vi "Cascade front panel 64.vi"() -> ()   [LabVIEW 2016]
uses:
  controls/KPro Header Control 1.ctl
  sdi_12/SDI-12/Sonde Vertical Graph.ctl
  controls/Vertical Chart.ctl
  sdi_12/Groundwater header.ctl
  controls/MCC DAQ Setup.ctl
  controls/Aux Sensor.ctl
  KPRO_2016 subvis/Control 2.ctl
  KPRO_2016 subvis/Graph Controls 2.ctl
  KPRO_2016 subvis/Ik control.ctl
  controls/MCC DAQ Readings.ctl
  controls/Kpro pressure measurement cluster.ctl
  controls/Kpro hydraulic measurement cluster.ctl
  Cascade/Waterloo DAQ/controls/Sonde Data Array Control 1.ctl
  Cascade/Waterloo DAQ/controls/Sonde Data Control 1.ctl
  sdi_12/Sonde Value Percent Tol.ctl
  activeXtest/activeXtest 2015 Folder/sample data row cluster.ctl
  activeXtest/activeXtest 2015 Folder/sonde cluster.ctl
  controls/Display Control 1.ctl
  KPRO_2016 subvis/Sensor Physical Measurements.ctl
  KPRO_2016 subvis/SS Control 7.ctl
  <vilib>/Utility/NIReport.llb/NI_report.lvclass
  controls/Action Control 1.ctl
  <extravilib>/ChannelInstances/One Element Stream-t'Action Control 1.ctl'/Instantiate.vi
  <extravilib>/ChannelInstances/One Element Stream-t'Action Control 1.ctl'/EndpointRead.vi
  KPRO_2016 subvis/Kpro Globals.vi
  <vilib>/Utility/file.llb/Write Delimited Spreadsheet (DBL).vi
  <vilib>/Utility/file.llb/Write Delimited Spreadsheet (string).vi
  <vilib>/ULx/Create Channel.llb/ULx Create Channel (AI-Voltage-Basic).vi
  <userlib>/_OpenG.lib/file/file.llb/Build Path - Traditional__ogtk.vi
  <userlib>/_OpenG.lib/file/file.llb/File Exists - Scalar__ogtk.vi
  <userlib>/_OpenG.lib/file/file.llb/Strip Path - Traditional__ogtk.vi
  KPRO_2016 subvis/Global_SIM_switch.vi
  <extravilib>/ChannelInstances/One Element Stream-t'Action Control 1.ctl'/Endpoint.vi
  C:/Program Files/National Instruments/LabVIEW 2016/vi.lib/ULx/ULx_LV.dll
  Program Files/National Instruments/LabVIEW 2016/vi.lib/ULx/ULx_LV.dll
  <vilib>/Utility/config.llb/NI_LVConfig.lvlib
  <extravilib>/ChannelInstances/One Element Stream-t'Action Control 1.ctl'.lvlib
panel:
  out "Zero Pressure\nIndicator":bool
  in  "Zero\nPressure":bool caption="Zero Pressure"
  in  "enable_IKMGS_file":bool
  in  "enable_slug_file":bool
  in  "enable_kpro_file":bool=TRUE
  in  "Simulate AD6B":bool
  out "KPRO Test\nIndicator":bool
  in  "Record DTW File":bool
  in  "Zero In-Line Pressure\n(F = leave as is)":bool=TRUE
  in  "Corrected Pressure Cluster":T1
  in  "Create Excel Files":bool
  out "Tab Page":i32
  out "Sonde Data":string[][](array[string])
  out "Current \nDepth (m)":sgl=-30.661383 format="%.2f"
  out "Sonde Recording":string[][](array[string])
  out "Column of Volume":i32
  in  "Input Variables and Slopes 2":T2={"Total Volume"=0.0, "String Pot Slope"=1.6619999408721924, "Flow Slope"=39.040000915527344, "Up Hole Pressure Slope"=48.27000045776367, "Depth to Water Table"=-0.0, "Atmospheric Pressure"=32.22022530555725, "DH Pressure Trans Slope"=42.0, "DH Pressure Offset"=0.0, "Up Hole  Pressure Offset"=0.0, "Aux 1 Slope"=1.0, "Aux 2 Slope"=1.0, "Aux 3 Slope"=1.0, "Aux 1 Offset"=0.0, "Aux 2 Offset"=0.0, "Aux 3 Offset"=0.0, "String Pot Offset"=0.0, "Flow Offset"=0.0, "Reservoir Pressure"=-0.004827000045779073, "Height of Sample Box"=0.0} {"Height of Sample Box" format="%.2f"; "Reservoir Pressure" format="%.2f"; "Flow Offset" format="%.2f"; "String Pot Offset" format="%.2f"; "Aux 3 Offset" format="%.2f"; "Aux 2 Offset" format="%.2f"; "Aux 1 Offset" format="%.2f"; "Aux 3 Slope" format="%.2f"; "Aux 2 Slope" format="%.2f"; "Aux 1 Slope" format="%.2f"; "Up Hole  Pressure Offset" format="%.2f"; "DH Pressure Offset" format="%.2f"; "DH Pressure Trans Slope" format="%.2f"; "Atmospheric Pressure" format="%.2f"; "Depth to Water Table" format="%.2f"; "Up Hole Pressure Slope" format="%.2f"; "Flow Slope" format="%.2f"; "String Pot Slope" format="%.2f"; "Total Volume" format="%.2f"}
  out "Select Worksheet Index":i32
  out "Number of Sample Sheets":i32
  out "NI_report out":refnum<class "NI_report.lvclass">
  out "Sonde":bool
  out "DAQ":bool
  in  "Depth mode":bool=TRUE caption="Use \nIncrement"
  in  "Increment Depth":bool
  in  "Finish Tests":bool
  in  "Start KPRO":bool
  in  "stop":bool
  in  "Write Data to Spreadsheet":bool
  in  "Sonde Sample Not Collected":bool
  in  "Record Single Sample":bool
  in  "Sample Sheet Data Row Cluster 2":T3={"Head\nPressure"=0.0, "Depth"=0.0, "comment "="", "Sonde Data Cluster"={"Cumulative\nVolume (ml)"=100.0, "Specific\nCond (mS)"=2.0, "Dissolved\nOxygen mg/L"=3.0, "pH"=4.0, "ORP"=5.0, "Temp deg C"=26.0, "Salinity"=7.0}, "Aux1"=0.0, "Aux2"=0.0, "Aux3"=0.0} {"Sonde Data Cluster"."Salinity" format="%_3g"; "Sonde Data Cluster"."Temp deg C" format="%_2g"; "Sonde Data Cluster"."ORP" format="%_4g"; "Sonde Data Cluster"."pH" format="%_4g"; "Sonde Data Cluster"."Dissolved\nOxygen mg/L" format="%_4g"; "Sonde Data Cluster"."Specific\nCond (mS)" format="%_4g"; "Sonde Data Cluster"."Cumulative\nVolume (ml)" format="%#_4g"; "Depth" format="%#.3g"; "Head\nPressure" format="%#.4g"}
  out "Current Time (s)":dbl
  in  "Tab Control":T5(tab)
  out "Height of Box Global":dbl
  out "Depth to Water Table Global":dbl
  out "Reservoir Pressure Global":dbl
  out "Atmospheric Pressure Global":dbl
  out "Current Depth Global":dbl
  out "Increment Global":dbl
  out "Distance Global":dbl
  out "Profile ID":string
  out "KPRO Box Global":dbl
  out "Ion Offset Global":dbl
  out "Ion Slope Global":dbl
  out "Flow Slope Global":dbl
  out "Pressure Slope Global":dbl
  out "String Pot  Slope Global":dbl
  in  "Config File Path":path=path "C:/Cascade/Data/config files/DAQ Setup Config.ini"
  in  "Read Configuration File?":bool
  in  "Save Configuration File?":bool
  out "12V Voltage Monitor":dbl format="%_3f"
  out "Found Quanta Sonde Com Port":refnum<visa-resource-name>
  out "Quanta Sonde found?":bool
  out "H-4191 Adapter found":bool
  out "Sonde Communication Error Out":errorcluster
  in  "Search for Comm Ports?":bool=TRUE
  in  "USB Serial Port Manual Entry":refnum<visa-resource-name>="COM13"
  in  "Sonde Parameters \nTolerance Limits":T6={"SC %"=10.0, "DO %"=10.0, "pH % "=10.0, "ORP % "=10.0, "Temp % "=10.0, "Salinity %"=10.0} {"Salinity %" format="%_2f%%"; "Temp %" format="%_2f%%"; "ORP %" format="%_2f%%"; "pH %" format="%_2f%%"; "DO %" format="%_2f%%"; "SC %" format="%_2f%%"}
  in  "Sonde Parameters \nInitial Values":T7 {"Salinity Initial" format="%_2f"; "Temp Initial" format="%_2f"; "ORP  Initial" format="%_2f"; "pH Initial" format="%_2f"; "DO Initial" format="%_2f"; "SC Initial" format="%_2f"}
  out "Sensor  Real \nMeasurements":T8 {"9V Monitor" format="%#.3g"; "Aux 3" format="%#.3g"; "Aux 2" format="%#.3g"; "Aux 1" format="%#.3g"; "String Pot" format="%#.3g"; "Top String Pot" format="%#_4g"; "Downhole Pressure" format="%#_4g"; "Flow" format="%#_4g"; "Uphole Pressure" format="%#_4g"}
  in  "MCC USB-DAQ Setup":T9={"Device Name in InstaCal"="Dev0", "Omega Pressure Sensor"={"DAQ Channel"=2.0, "Input Voltage Range"=1, "Enabled"=TRUE, "Description"="Uphole Pressure"}, "McMillian 102 Flowmeter"={"DAQ Channel"=11.0, "Input Voltage Range"=0, "Enabled"=TRUE, "Description"="Flow"}, "DHT Pressure Sensor"={"DAQ Channel"=3.0, "Input Voltage Range"=1, "Enabled"=TRUE, "Description"="Downhole Pressure"}, "Top String Pot"={"DAQ Channel"=0.0, "Input Voltage Range"=0, "Enabled"=TRUE, "Description"="Top String Pot"}, "String Pot Signal"={"DAQ Channel"=1.0, "Input Voltage Range"=0, "Enabled"=TRUE, "Description"="String Pot"}, "Aux Sensor 1"={"DAQ Channel"=5.0, "Input Voltage Range"=1, "Enabled"=TRUE, "Description"="Aux 1"}, "Aux Sensor 2"={"DAQ Channel"=6.0, "Input Voltage Range"=1, "Enabled"=TRUE, "Description"="Aux 2"}, "Aux Sensor 3"={"DAQ Channel"=7.0, "Input Voltage Range"=1, "Enabled"=TRUE, "Description"="Aux 3"}, "Voltage Monitor"={"DAQ Channel"=8.0, "Input Voltage Range"=0, "Enabled"=TRUE, "Description"="9V Monitor"}} {"Voltage Monitor"."Input Voltage Range" items=["+/-10 V Range", "+/-5 V Range", "+/-2.5V Range", "+/-1.25 V Range", "+/-0.625 V Range", "+/-0.3125 V Range", "+/-0.1562V Range", "+/-0.078125 V Range"]; "Aux Sensor 3"."Input Voltage Range" items=["+/-10 V Range", "+/-5 V Range", "+/-2.5V Range", "+/-1.25 V Range", "+/-0.625 V Range", "+/-0.3125 V Range", "+/-0.1562V Range", "+/-0.078125 V Range"]; "Aux Sensor 2"."Input Voltage Range" items=["+/-10 V Range", "+/-5 V Range", "+/-2.5V Range", "+/-1.25 V Range", "+/-0.625 V Range", "+/-0.3125 V Range", "+/-0.1562V Range", "+/-0.078125 V Range"]; "Aux Sensor 1"."Input Voltage Range" items=["+/-10 V Range", "+/-5 V Range", "+/-2.5V Range", "+/-1.25 V Range", "+/-0.625 V Range", "+/-0.3125 V Range", "+/-0.1562V Range", "+/-0.078125 V Range"]; "String Pot Signal"."Input Voltage Range" items=["+/-10 V Range", "+/-5 V Range", "+/-2.5V Range", "+/-1.25 V Range", "+/-0.625 V Range", "+/-0.3125 V Range", "+/-0.1562V Range", "+/-0.078125 V Range"]; "Top String Pot"."Input Voltage Range" items=["+/-10 V Range", "+/-5 V Range", "+/-2.5V Range", "+/-1.25 V Range", "+/-0.625 V Range", "+/-0.3125 V Range", "+/-0.1562V Range", "+/-0.078125 V Range"]; "DHT Pressure Sensor"."Input Voltage Range" items=["+/-10 V Range", "+/-5 V Range", "+/-2.5V Range", "+/-1.25 V Range", "+/-0.625 V Range", "+/-0.3125 V Range", "+/-0.1562V Range", "+/-0.078125 V Range"]; "McMillian 102 Flowmeter"."Input Voltage Range" items=["+/-10 V Range", "+/-5 V Range", "+/-2.5V Range", "+/-1.25 V Range", "+/-0.625 V Range", "+/-0.3125 V Range", "+/-0.1562V Range", "+/-0.078125 V Range"]; "Omega Pressure Sensor"."Input Voltage Range" items=["+/-10 V Range", "+/-5 V Range", "+/-2.5V Range", "+/-1.25 V Range", "+/-0.625 V Range", "+/-0.3125 V Range", "+/-0.1562V Range", "+/-0.078125 V Range"]}
  out "Rate":dbl=1000.0 caption="Channel\nSample Rate (Hz)"
  out "Number \nof Channels":u16
  in  "DAQ \nData Rate S/s":dbl=3720.0 format="%#_13g"
  out "Descriptions":string[](array[string])
  out "Raw Voltages":dbl[](array[numeric])
  out "9V Voltage Monitor":dbl format="%#_3g"
  in  "Record DAQ Raw Voltages":bool
  out "Sensor Voltage Cluster":T11 {"9V Monitor" format="%#.3g"; "Aux 3" format="%#_3g"; "Aux 2" format="%#.3g"; "Aux 1" format="%#.3g"; "String Pot" format="%#.3g"; "Top String Pot" format="%#_3g"; "Downhole Pressure" format="%#.3g"; "Flow" format="%#_3g"; "Uphole Pressure" format="%-#1.3g"}
  out "Worksheet Names":string[](array[string])
  out "row max value":i32
  out "last occupied cell's name":string
  out "column max value":i32
  in  "Current Sample Sheet":string="Sample 1"
  out "Columns":i32[](array[numeric])
  in  "Header path":path=path "C:/Cascade/templates/Fields for Excel sheets.xlsx"
  in  "template file path":path=path "C:/Cascade/templates/Groundwater Profiling Log_empty_labview_template.xlsx"
  in  "Data File Directory":path=path "C:/Cascade/Data/Excel Reports"
  in  "Excel report file path":path=path "C:/Cascade/Data/Excel Reports/Groundwater Profiling Log_ara1.xlsx"
  in  "Clear Groundwater Header Values":bool
  in  "Groundwater Header":T12
  out "Data Setup Indicator":string
  in  "Start Initialization":bool
  in  "Input Variables and Slopes":T2={"Total Volume"=0.0, "String Pot Slope"=1.6619999408721924, "Flow Slope"=39.040000915527344, "Up Hole Pressure Slope"=48.27000045776367, "Depth to Water Table"=-0.0, "Atmospheric Pressure"=32.22022530555725, "DH Pressure Trans Slope"=42.0, "DH Pressure Offset"=0.0, "Up Hole  Pressure Offset"=0.0, "Aux 1 Slope"=1.0, "Aux 2 Slope"=1.0, "Aux 3 Slope"=1.0, "Aux 1 Offset"=0.0, "Aux 2 Offset"=0.0, "Aux 3 Offset"=0.0, "String Pot Offset"=0.0, "Flow Offset"=0.0, "Reservoir Pressure"=-0.004827000045779073, "Height of Sample Box"=0.0} {"Height of Sample Box" format="%.2f"; "Reservoir Pressure" format="%.2f"; "Flow Offset" format="%.2f"; "String Pot Offset" format="%.2f"; "Aux 3 Offset" format="%.2f"; "Aux 2 Offset" format="%.2f"; "Aux 1 Offset" format="%.2f"; "Aux 3 Slope" format="%.2f"; "Aux 2 Slope" format="%.2f"; "Aux 1 Slope" format="%.2f"; "Up Hole  Pressure Offset" format="%.2f"; "DH Pressure Offset" format="%.2f"; "DH Pressure Trans Slope" format="%.2f"; "Atmospheric Pressure" format="%.2f"; "Depth to Water Table" format="%.2f"; "Up Hole Pressure Slope" format="%.2f"; "Flow Slope" format="%.2f"; "String Pot Slope" format="%.2f"; "Total Volume" format="%.2f"}
  out "appended path":path
  out "Down hole Pressure Transducer CSV data  path":path
  in  "Static IK path":path
  in  "Slopes File Path":path=path "C:/Cascade/Data/Output Files/slopes.csv"
  out "Output File Path":path
  out "KPRO SessionOutput File Path":path
  in  "Slopes History File Path":path=path "C:/Cascade/Data/Output Files/slopes-cal-record.csv"
  out "Sonde Recording Error file":path
  out "IK Recording Error file":path
  out "Sonde Output File Path":path
  out "KPRO Cumulative Output File Path":path
  in  "Temporary Data Files Directory":path=path "C:/Cascade/Data/Output Files"
  in  "Update Sonde":bool
  in  "Sonde Data Array":T13 {"Salinity"."%" format="%_2f%%"; "Salinity"."Value" format="%_4g"; "Temperature"."%" format="%_2f%%"; "Temperature"."Value" format="%_4g"; "ORP"."%" format="%_2f%%"; "ORP"."Value" format="%_4g"; "pH"."%" format="%_2f%%"; "pH"."Value" format="%_4g"; "Dissolved Oxygen"."%" format="%_2f%%"; "Dissolved Oxygen"."Value" format="%_4g"; "Sp. Conductance"."%" format="%_2f%%"; "Sp. Conductance"."Value" format="%_4g"; "Cumulative\nVolume" format="%#_4g"}
  out "Table Label":string="Data from Sample  %d from Excel File"
  out "Sonde Array Size":i32
  in  "Current Sonde Sample":i32=1
  out "Sonde Data Display":T16
  out "Temperature":cluster{"Y":dbl[], "Y":dbl[]}[](graph)
  in  "Record  Sonde Reason":bool
  in  "Select Reasons to Record Data":u16(ring) items=["Per Client Request", "Timed Out", "Sample stopped flowing", "Equipment Issue"]
  out "Sonde Recording Failure Path":path
  in  "Sonde IK Recording Failure Path":path
  out "Recording Reason Sonde array":string[][](array[string])
  out "IK Reason array":string[][](array[string])
  in  "Sonde Calibration History File":path
  out "SC Reference (uS/cm) Calibration Response":T18
  out "DO Reference % Calibration Response":T18
  out "Salinity Reference Calibration Response":T18
  out "ORP Reference Calibration Response":T18
  out "pH Reference Calibration Response":T18
  out "pH Zero Calibration Response":T18
  in  "Salinity \nReference":dbl
  in  "SC \nReference (uS/cm)":dbl
  in  "DO Reference %":dbl
  in  "ORP Reference":dbl
  in  "pH Reference":dbl
  in  "pH Zero":dbl
  in  "Record  SC Calibration":bool
  in  "Record DO Calibration":bool
  in  "Record Salinity Calibration":bool
  in  "Record ORP Calibration":bool
  in  "Record pH Calibration Reference":bool
  in  "Record pH Calibration Zero":bool
  out "KPRO Finish\nIndicator":bool
  in  "Input Depths \nand Parameters Cluster":T19={"Flow"=0.21081600494384767, "Zeroed \nPressure"=74.74207969932556, "Ik"=0.003788962123473114, "Current Depth"=-100.6, "Feet of Stainless"=40, "Start Depth"=0.0, "Abs Start Depth"=0.0} {"Abs Start Depth" format="%.2f"; "Start Depth" format="%.2f"; "Current Depth" format="%.2f"; "Ik" format="%.2f"; "Zeroed \nPressure" format="%.2f"; "Flow" format="%.2f"}
  out "Current Session":sgl[][](array[numeric]) format="%.2f"
  in  "KPRO session report header":T20=["Time(msecs)", "Uncorrected Depth", "Corrected Depth", "Drive_Rate", "Flow", "Feet_of Stainless", "Up Hole Pressure", "IK", "Corrected Pressure", "Atm Pressure", "Depth to water", "Height of box", "Res_Pressure", "Secs_since_1_JAN_1904", "Depth jumps more than 1_foot", "Down hole Pressure"]
  in  "Depth Cluster":T21
  out "Cumulative_data_from_file":sgl[][](array[numeric]) format="%.2f"
  in  "KPRO Culmulative \ntest report header 2":T20=["Time(msecs)", "Uncorrected Depth", "Corrected Depth", "Drive_Rate", "Flow", "Feet_of Stainless", "Up Hole Pressure", "IK", "Corrected Pressure", "Atm Pressure", "Depth to water", "Height of box", "Res_Pressure", "Secs_since_1_JAN_1904", "Depth jumps more than 1_foot", "Down hole Pressure"]
  out "Cumulative_data_ready":bool
  out "DHT IK":T22=0.003788962123473114 caption="Real Time - Depth vs. lk" format="%.2f"
  out "Depth to Water":sgl=-100.6 format="%.2f"
  out "Depth Rate\nft/min":T22 format="%#.2g"
  out "Ik":dbl=0.003788962123473114 caption="Real Time - Depth vs. lk" format="%.2f"
  out "Corrected\n Pressure (ft)":dbl format="%.2f"
  in  "New Depth":dbl min=-100.0 max=0.0
  in  "Update Depth":bool
  in  "Select Entry \nfor IK Log":u16(ring) items=["IK Increase", "IK stayed the Same", "IK decreased"]
  out "Large Depth IK Graph Cluster":T23={[0.003788962123473114, 0.0037174584307500765, 0.0037174584307500765, 0.0037174584307500765, 0.0037174584307500765, 0.003788962123473114], [-100.1, -100.2, -100.3, -100.4, -100.5, -100.6]}
  in  "Culmulative Graph Cluster":T24={"Cumulative - Depth vs. Ik"={[], []}, "Real Time - Depth vs. lk "={[0.003788962123473114, 0.0037174584307500765, 0.0037174584307500765, 0.0037174584307500765, 0.0037174584307500765, 0.003788962123473114], [-100.1, -100.2, -100.3, -100.4, -100.5, -100.6]}, "Cumulative - Depth vs. Drive Rate"={[], []}, "Real Time - Depth vs. Drive Rate"={[0.02036245163917736, 0.125, 0.16666666666666674, 0.16666666666666663, 0.16666666666666663, 0.16666666666666663], [-100.1, -100.2, -100.3, -100.4, -100.5, -100.6]}}
  out "Down hole Pressure (ft)":dbl format="%.2f"
  out "Flow":T22 format="%#.2g"
  out "Current Depth":sgl=-100.6 format="%.2f"
  in  "Read String Pot":bool=TRUE
  in  "Record IK Reason":bool
  out "Large Depth IK Graph":dbl(graph)
  out "DAQ Error":errorcluster
  out "Initialization Finished":bool=TRUE
  out "Stop":bool
  out "error out":errorcluster
  in  "error in (no error)":errorcluster
  out "producer loop":i32
  out "consumer loop":i32
  out "Active Channel Array":string[](array[string])
  out "Voltage Range":dbl[](array[numeric])
  out "delimited string":string
  out "Stop 2":bool
  out "output cluster":T4 caption="Cluster" {"Salinity" format="%_3g"; "Temp deg C" format="%_2g"; "ORP" format="%_4g"; "pH" format="%_4g"; "Dissolved\nOxygen mg/L" format="%_3g"; "Specific\nCond (mS)" format="%_4g"; "Cumulative\nVolume (ml)" format="%#_4g"}
  out "Serial Number/MISC":string
  out "subarray":string[][](array[string])
  out "Initialization":i32
  in  "Record Continuous Samples":bool
  # "Global Variables"
  # "ft. water"
  # "mL/min."
  # "ft. water"
  # "ft."
  # "ft."
  # "Instructions for Sonde Calibration:\n1.  Use the Record Single Point to Record the Data prior to start of\ncalibration procedure to record the initial points to the excel worksheet.\n2.  pH Calibration is a 2 step process:  A pH standard between 6.8 and 7.2 is treated as the “zero”\nand all other values are treated as the “slope”. First calibrate “zero”, then  add a second to calibrate “slope”. \n3.  Specific Conductance:  Wait for the specific conductance readings to stabilize in the calibration solution, which may\nrequire one or two minutes."
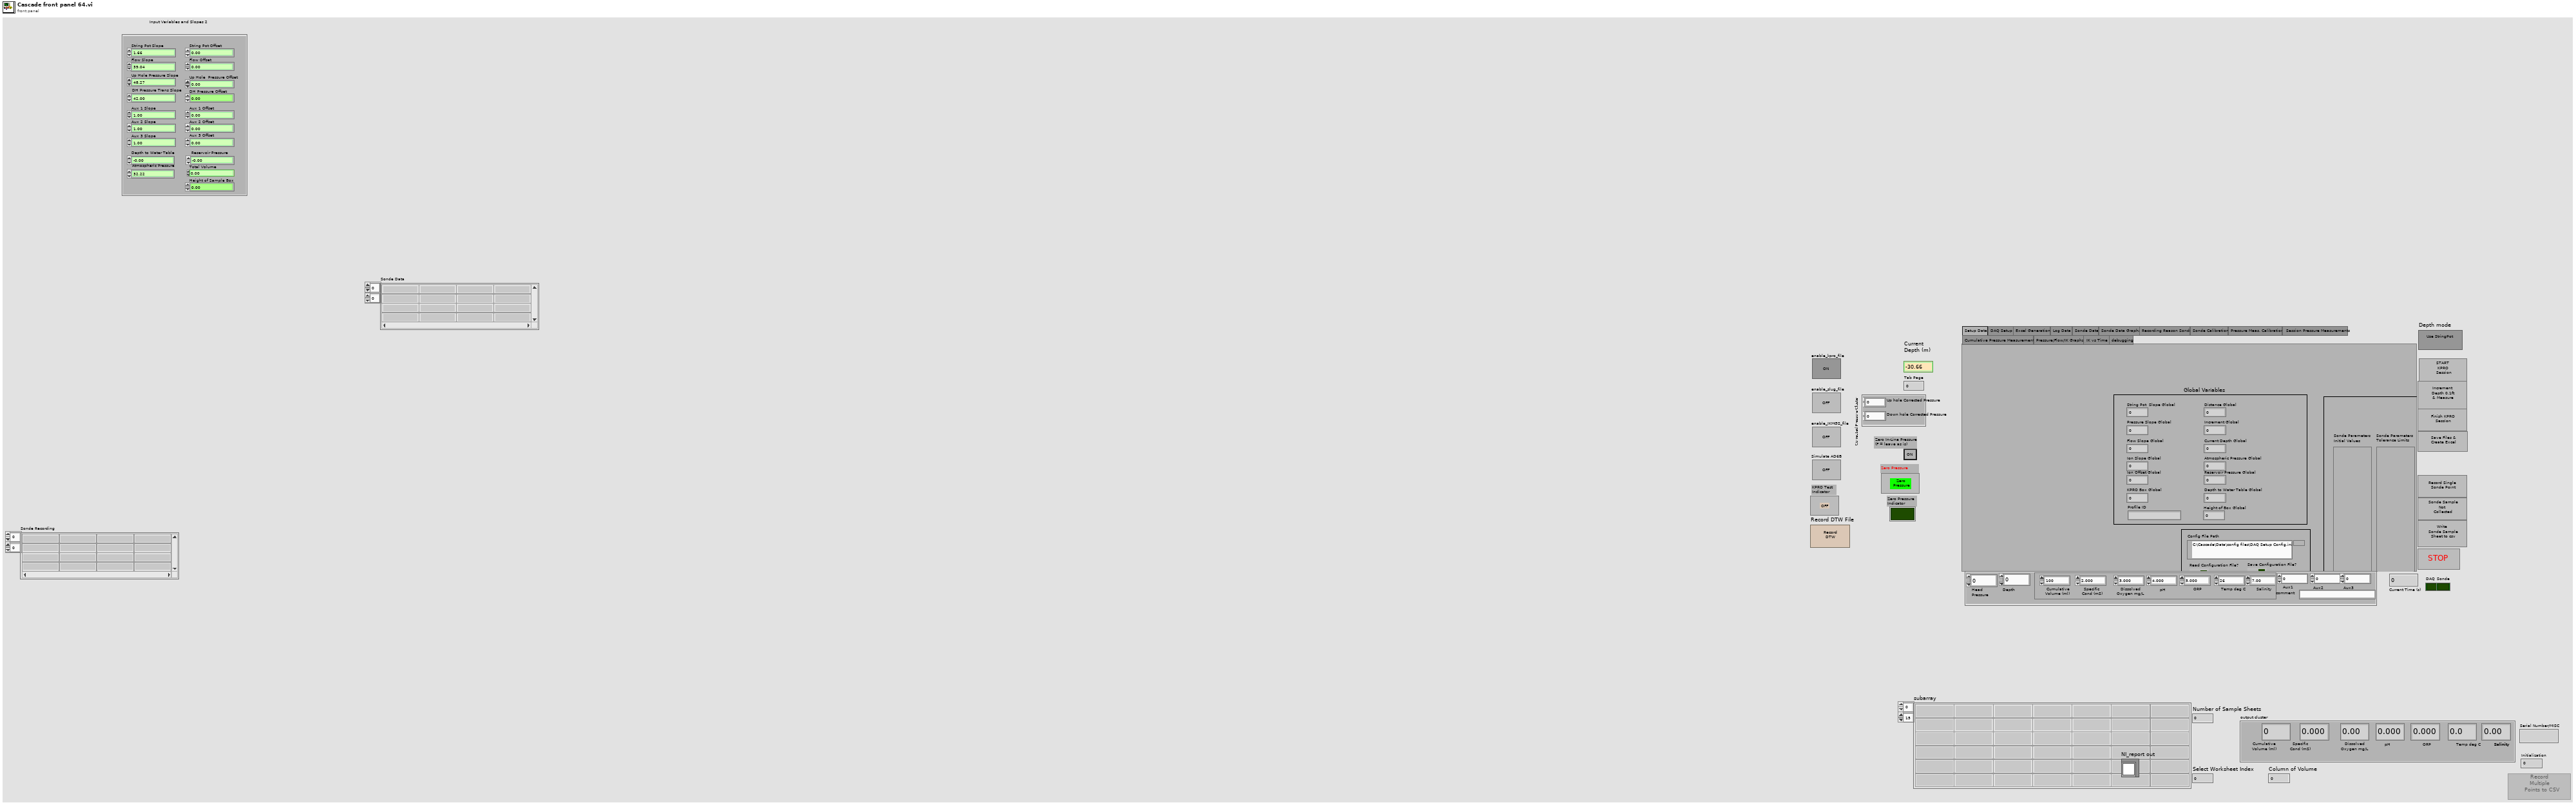
[diagram p1: front panel]
types:
  T1 = typedef "Kpro pressure measurement cluster.ctl" = cluster{"Up hole Corrected Pressure":dbl, "Down hole Corrected Pressure":dbl}
  T2 = typedef "Control 2.ctl" = cluster{"Total Volume":dbl, "String Pot Slope":dbl, "Flow Slope":dbl, "Up Hole Pressure Slope":dbl, "Depth to Water Table":dbl, "Atmospheric Pressure":dbl, "DH Pressure Trans Slope":dbl, "DH Pressure Offset":dbl, "Up Hole  Pressure Offset":dbl, "Aux 1 Slope":dbl, "Aux 2 Slope":dbl, "Aux 3 Slope":dbl, "Aux 1 Offset":dbl, "Aux 2 Offset":dbl, "Aux 3 Offset":dbl, "String Pot Offset":dbl, "Flow Offset":dbl, "Reservoir Pressure":dbl, "Height of Sample Box":dbl}
  T3 = typedef "sample data row cluster.ctl" = cluster{"Head\nPressure":dbl, "Depth":dbl, "comment ":string, "Sonde Data Cluster":T4, "Aux1":dbl, "Aux2":dbl, "Aux3":dbl}
  T4 = typedef "sonde cluster.ctl" = cluster{"Cumulative\nVolume (ml)":dbl, "Specific\nCond (mS)":dbl, "Dissolved\nOxygen mg/L":dbl, "pH":dbl, "ORP":dbl, "Temp deg C":dbl, "Salinity":dbl}
  T5 = enum32{"Setup Data", "DAQ Setup", "Excel Generation", "Log Data", "Sonde Data", "Sonde Data Graphs", "Recording Reason Sonde", "Sonde Calibration", "Pressure Meas. Calibration", " Session Pressure Measurements", "Cumulative Pressure Measurements", "Pressure/Flow/IK Graphs", "IK vs Time ", "debugging"}
  T6 = cluster{"SC %":dbl, "DO %":dbl, "pH % ":dbl, "ORP % ":dbl, "Temp % ":dbl, "Salinity %":dbl}
  T7 = cluster{"SC Initial ":dbl, "DO Initial ":dbl, "pH Initial  ":dbl, "ORP  Initial":dbl, "Temp Initial":dbl, "Salinity Initial ":dbl}
  T8 = typedef "Sensor Physical Measurements.ctl" = cluster{"Uphole Pressure":dbl, "Flow":dbl, "Downhole Pressure":dbl, "Top String Pot":dbl, "String Pot":dbl, "Aux 1":dbl, "Aux 2":dbl, "Aux 3":dbl, "9V Monitor":dbl}
  T9 = typedef "MCC DAQ Setup.ctl" = cluster{"Device Name in InstaCal":string, "Omega Pressure Sensor":T10, "McMillian 102 Flowmeter":T10, "DHT Pressure Sensor":T10, "Top String Pot":T10, "String Pot Signal":T10, "Aux Sensor 1":T10, "Aux Sensor 2":T10, "Aux Sensor 3":T10, "Voltage Monitor":T10}
  T10 = typedef "Aux Sensor.ctl" = cluster{"DAQ Channel":dbl, "Input Voltage Range":u16, "Enabled":bool, "Description":string}
  T11 = typedef "MCC DAQ Readings.ctl" = cluster{"Uphole Pressure":dbl, "Flow":dbl, "Downhole Pressure":dbl, "Top String Pot":dbl, "String Pot":dbl, "Aux 1":dbl, "Aux 2":dbl, "Aux 3":dbl, "9V Monitor":dbl}
  T12 = typedef "Groundwater header.ctl" = cluster{"Location":string, "Date Finished":string, "CTS":string, "sampler":string, "Kpro box Serial ":string, "Sonde Serial":string, "Drilling Contractor":string, "Ave Depth to Water":string, "Gas/Peri Pump":string, "Atmospheric Pressure":string, "KPRO N2 Pressure":string, "Gas Drive N2 Pressure":string, "Profile ID":string, "Client":string}
  T13 = typedef "Sonde Data Array Control 1.ctl" = T14[]
  T14 = typedef "Sonde Data Control 1.ctl" = cluster{"Head":dbl, "Depth":dbl, "Time":string, "Cumulative\nVolume":dbl, "Sp. Conductance":T15, "Dissolved Oxygen":T15, "pH":T15, "ORP":T15, "Temperature":T15, "Salinity":T15, "Final Tol.":bool, "Final":bool, "Time 2":timestamp, "Aux 1":dbl, "Aux 2":dbl, "Aux 3":dbl}
  T15 = typedef "Sonde Value Percent Tol.ctl" = cluster{"Value":dbl, "%":dbl, "Tol.":bool}
  T16 = typedef "Sonde Vertical Graph.ctl" = cluster{"pH":T17, "Conductance":T17, "Salinity":T17, "DO % Saturation":T17, "DO mg/L":T17, "ORP":T17}
  T17 = typedef "Vertical Chart.ctl" = cluster{"Y":dbl[], "Y":dbl[]}[]
  T18 = cluster{"Valid":bool, "Value":dbl, "\nString ":string}
  T19 = typedef "SS Control 7.ctl" = cluster{"Flow":dbl, "Zeroed \nPressure":dbl, "Ik":dbl, "Current Depth":sgl, "Feet of Stainless":i32, "Start Depth":sgl, "Abs Start Depth":sgl}
  T20 = typedef "KPro Header Control 1.ctl" = string[]
  T21 = typedef "Kpro hydraulic measurement cluster.ctl" = cluster{"Absolute Depth In":dbl, "Current Absolute Depth":dbl, "First Absolute Depth":dbl, "Previous Relative Depth":dbl, "Current Relative Depth":dbl, "First Relative Depth":dbl, "Last Filed Depth":dbl, "Total Volume In":dbl, "Total Volume Out":dbl, "Current Measurement Time":dbl, "Previous Measurement Time":dbl}
  T22 = typedef "Display Control 1.ctl" = dbl
  T23 = typedef "Ik control.ctl" = cluster{dbl[], dbl[]}
  T24 = typedef "Graph Controls 2.ctl" = cluster{"Cumulative - Depth vs. Ik":cluster{dbl[], dbl[]}, "Real Time - Depth vs. lk ":cluster{dbl[], dbl[]}, "Cumulative - Depth vs. Drive Rate":cluster{dbl[], dbl[]}, "Real Time - Depth vs. Drive Rate":cluster{dbl[], dbl[]}}
  T25 = typedef "NI_LVConfig.lvlib/Config Data RefNum.ctl" = refnum<k1>
  T26 = enum8{"Enabled", "Disabled", "Disabled and Grayed Out"}
  T27 = typedef "Action Control 1.ctl" = enum16{"TimeOut", "Continuous  Sonde Data", "Init", "Exit", "Acq. Single Sonde Point", "Write Sonde Sample Sheet", "Acq. DAQ data", "Sonde Sample Not Collected", "Record Sonde Reason", "pH Calibration Zero", "pH Calibration Standard", "ORP Calibration Standard", "Salinity Calibration Standard", "DO Calibration Standard", "SC Calibration Standard", "Increment Depth Manually", "Start KPRO Measurements", "Finish KPRO Measurements", "Update Depth", "IK vs Time", "Record IK Reason", "Create Excel Files"}
  T28 = typedef "One Element Stream-t'Action Control 1.ctl'.lvlib/)Channel.ctl" = refnum<queue>
  T29 = cluster{"Head":dbl, "Depth":dbl, "Time":string, "Cumulative\nVolume":dbl, "Sp. Conductance":T15, "Dissolved Oxygen":T15, "pH":T15, "ORP":T15, "Temperature":T15, "Salinity":T15, "Final Tol.":bool, "Final":bool, "Time 2":timestamp, "Aux 1":dbl, "Aux 2":dbl, "Aux 3":dbl}[]
  T30 = typedef "sonde cluster from excel.ctl" = cluster{"Head":dbl, "Depth":dbl, "Time":string, "Cumulative\nVolume":dbl, "Sp. Conductance":T15, "Dissolved Oxygen":T15, "pH":T15, "ORP":T15, "Temperature":T15, "Salinity":T15, "Final Tol.":bool, "Final":bool, "Time 2":timestamp, "Aux 1":dbl, "Aux 2":dbl, "Aux 3":dbl}
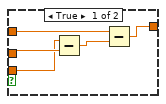
[diagram p9: hidden frame]
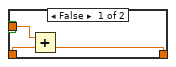
[diagram p16: hidden frame]
diagram:
  # "For calibrate command (XC) on SDI-12 address ‘a’, P is pH, C is specific conductance, S is\nsalinity or TDS, % is DO %Saturation, O is DO mg/L, R is ORP, D is depth, B is\nbarometric pressure, and t is TDS scale factor."
  n1 = flat-sequence {
    tunnel: [w20] -> w5
    tunnel: [w52] -> w7
    tunnel: w5 -> [w52]
    tunnel: [w48] -> w3
    tunnel: [w55] -> w14
    tunnel: w7 -> [w54]
    tunnel: [w55] -> w6
    tunnel: w14 -> [w108]
    tunnel: [w99] -> w12
    tunnel: [w103] -> w11
    tunnel: [w102] -> w8
    tunnel: [w100] -> w9
    tunnel: [w101] -> w10
    tunnel: [w104] -> _
    tunnel: [w106] -> w13
    tunnel: [w109] -> w2
    tunnel: [w110] -> w1
    frame #0 {
      n2 = invoke on="error out" class="Clust (strict)" method="Reinit To Default"(error in="error in (no error)") -> (error out=w18:errorcluster)  [unwired: 2 in, 2 out]
      n3 = flat-sequence {
        tunnel: [w24] -> w20
        tunnel: w18 -> [w23]
        frame #0 {
          n4 = case shown="False" "Read Configuration File?" {
            selector: "Read Configuration File?" -> [_ w31]
            tunnel: [w25 w36] -> w24
            tunnel: w23 -> [w25 w33]
            tunnel: "Config File Path" -> [_ w32]
            frame False {
            }
            frame True {
              n5 = call <vilib>:"Check if File or Folder Exists.vi"("error in (no error)"=w33, "path"=w32) -> ("error out"=w28:errorcluster, "file or folder exists?"=w29:bool, "dup path"=w27:path)  [unwired: 7 in]
              n6 = And(x=w31, y=w29) -> (x .and. y?=w30:bool)
              n7 = control-ref of="This VI"() -> (w34:refnum<vi>)
              n8 = case shown="True" w30 {
                selector: w30 -> [w37 _]
                tunnel: w27 -> [_ w42]
                tunnel: w28 -> [w38 w46]
                tunnel: [w38 w39] -> w35
                tunnel: w34 -> [_ w47]
                frame False {
                  n9 = local write "Read Configuration File?"(w37) -> ()
                }
                frame True {
                  n10 = call <vilib>:"Open Config Data.vi"("error in (no error)"=w46, "create file if necessary (T)"=FALSE, "configuration file path"=w42) -> ("error out"=w44:errorcluster, "refnum"=w45:T25)  [unwired: 6 in, 1 out]
                  n11 = call <userlib>:"Read Panel from INI__ogtk.vi"("error in (no error)"=w44, "VI ref"=w47, "refnum"=w45) -> ("error out"=w40:errorcluster, "refnum out"=w41:T25)  [unwired: 7 in]
                  n12 = call <vilib>:"Close Config Data.vi"("error in (no error)"=w40, "refnum"=w41) -> ("error out"=w39:errorcluster)  [unwired: 8 in, 1 out]
                }
              }
              n13 = call <vilib>:"Clear Errors.vi"("error in (no error)"=w35) -> ("error out"=w26:errorcluster)  [unwired: 5 in, 1 out]
              n14 = Merge Errors(w26) -> (w36:errorcluster)
            }
          }
        }
      }
    }
    frame #1 {
      n15 = control-ref of="Sonde Data Display"() -> ()  [unwired: 1 out]
      n16 = local write "Current Sonde Sample"(1 ("Current Sheet")) -> ()
      n17 = Get Date/Time In Seconds() -> (seconds since 1Jan1904=w49:timestamp)
      n18 = Get Date/Time In Seconds() -> (seconds since 1Jan1904=w48:timestamp)
      n19 = Subtract(x=w48, y=w49) -> (x-y=w50:dbl)
      n20 = To Double Precision Float(number=w50) -> (double precision float=→"Current Time (s)":dbl)
    }
    frame #2 {
      w66 = T26."Enabled" ("Disabled")
      w84 = T26."Disabled and Grayed Out" ("Disabled")
      n21 = invoke on="Current Sonde Sample" class="DigNum (strict)" method="Reinit To Default"(error in=w54) -> (error out=w78:errorcluster)  [unwired: 2 in, 2 out]
      n22 = local write "Initialization Finished"(FALSE ("Initialization Finished")) -> ()
      n23 = invoke on="Current Session" class="Arr (strict)" method="Reinit To Default"(error in=w54) -> ()  [unwired: 2 in, 3 out]
      n24 = invoke on="Sonde Sample Not Collected" class="Bool" method="Reinit To Default"(error in=w78) -> (error out=w81:errorcluster)  [unwired: 2 in, 2 out]
      n25 = invoke on="Record Continuous Samples" class="Bool" method="Reinit To Default"(error in=w81) -> (error out=w80:errorcluster)  [unwired: 2 in, 2 out]
      n26 = invoke on="Write Data to Spreadsheet" class="Bool" method="Reinit To Default"(error in=w80) -> (error out=w79:errorcluster)  [unwired: 2 in, 2 out]
      n27 = call "search for Quanta Sonde devices.vi"("VISA resource name"="USB Serial Port Manual Entry", "Search for Comm Ports?"="Search for Comm Ports?", "error in (no error)"=w54) -> ("12V monitor"=w65:dbl, "Com Port with Quanta Sonde devices"=w90:refnum<visa-resource-name>[], "Number of Quanta Sonde devices"=w89:i32, "Serial Number/MISC"=w68:string, "Number of Quanta Sonde devices > 0?"=→"Quanta Sonde found?":bool, "H-4191 Adapter found"=→"H-4191 Adapter found":bool, "Error Out"=w73:errorcluster)  [unwired: 4 in, 2 out]
      "12V Voltage Monitor" <- w65
      "Sonde Communication Error Out" <- w73
      "Serial Number/MISC" <- w68
      n28 = invoke on="Record Single Sample" class="Bool" method="Reinit To Default"(error in=w79) -> (error out=w58:errorcluster)  [unwired: 2 in, 2 out]
      n29 = property on="Record Continuous Samples" class="Bool"(error in=w58, "DisabledEnum"=w84) -> (error out=w85:errorcluster)  [unwired: 1 in, 1 out]
      n30 = local read "Groundwater Header"() -> (w67:T12)
      n31 = Greater Or Equal?(x=w65, y=11.75) -> (x >= y?=→"Sonde":bool)
      n32 = case shown="1" w89 {
        tunnel: w90 -> [_ w97]
        tunnel: [refnum<visa-resource-name> refnum ("RS232 Port Out") w95] -> w88
        frame 0, Default {
        }
        frame 1 {
          n33 = Index Array(array=w97, index=0) -> (element=w95:refnum<visa-resource-name>)
        }
      }
      "Found Quanta Sonde Com Port" <- w88
      n34 = property on="Record Single Sample" class="Bool"(error in=w85, "DisabledEnum"=w84) -> (error out=w86:errorcluster)  [unwired: 1 in, 1 out]
      n35 = invoke on="stop" class="Bool (strict)" method="Reinit To Default"(error in=w58) -> (error out=w83:errorcluster)  [unwired: 2 in, 2 out]
      n36 = Bundle By Name(cluster=w67, "Sonde Serial"=w68) -> (w69:T12)
      n37 = invoke on="Stop" class="Bool (strict)" method="Reinit To Default"(error in=w58) -> (error out=w75:errorcluster)  [unwired: 2 in, 2 out]
      n38 = property on="Sonde Sample Not Collected" class="Bool"(error in=w86, "DisabledEnum"=w84) -> (error out=w82:errorcluster)  [unwired: 1 in, 1 out]
      n39 = local write "Groundwater Header"(w69) -> ()
      n40 = property on="Write Data to Spreadsheet" class="Bool"(error in=w83, "DisabledEnum"=w84) -> (error out=w76:errorcluster)  [unwired: 1 in, 1 out]
      n41 = invoke on="Stop 2" class="Bool (strict)" method="Reinit To Default"(error in=w75) -> (error out=w74:errorcluster)  [unwired: 2 in, 2 out]
      n42 = call <vilib>:"Clear Errors.vi"("error in (no error)"=w73) -> ("error out"=w72:errorcluster)  [unwired: 5 in, 1 out]
      n43 = Merge Errors(w72, w74, w76, w82) -> (w56:errorcluster)
      n44 = flat-sequence {
        tunnel: [w93] -> w62
        tunnel: w56 -> [w93]
        frame #0 {
          n45 = local write "Tab Control"(T5."Log Data" ("Tab Control")) -> ()
        }
      }
      n46 = invoke on="Sonde Data Array" class="Arr (strict)" method="Reinit To Default"(error in=w62) -> (error out=w61:errorcluster)  [unwired: 2 in, 2 out]
      n47 = invoke on="Data Setup Indicator" class="Str" method="Reinit To Default"(error in=w61) -> (error out=w59:errorcluster)  [unwired: 2 in, 2 out]
      n48 = property on="Clear Groundwater Header Values" class="Bool"(error in=w59, "DisabledEnum"=w66) -> (error out=w60:errorcluster)  [unwired: 1 in, 1 out]
      n49 = property on="Start Initialization" class="Bool"(error in=w60, "DisabledEnum"=w66) -> (error out=w57:errorcluster)  [unwired: 1 in, 1 out]
      n50 = invoke on="Clear Groundwater Header Values" class="Bool" method="Reinit To Default"(error in=w57) -> (error out=w55:errorcluster)  [unwired: 2 in, 2 out]
    }
    frame #3 {
      n51 = while {
        tunnel: w108 -> [w129]
        tunnel: [w130] -> w105
        tunnel: [w135] -> _
        i -> [w135]
        stop <- w131 stop-if-true
        n52 = Get Date/Time In Seconds() -> (seconds since 1Jan1904=w120:timestamp)
        n53 = Format Date/Time String(seconds (now)=w120) -> (date/time string=w121:string)  [unwired: 2 in]
        n54 = local read "Groundwater Header"() -> (w128:T12)
        n55 = event shown="[1] \"Start Initialization\": Value Change" {
          selector: _ -> [_ _ _ _ _]
          dyn-events: _ -> [_ _ _ _ _]
          timeout: 100 -> [_ _ _ _ _]
          tunnel: [FALSE w154 TRUE ("Stop") w159 _] -> w124
          tunnel: w129 -> [_ _ _ _ w162]
          event Timeout {
            n56 = event-data() -> ()  [unwired: 1 in, 3 out]
          }
          event "Start Initialization": Value Change {
            n57 = event-data() -> ()  [unwired: 1 in, 3 out]
            n58 = case shown="True" "Start Initialization" {
              tunnel: [FALSE ("Stop") TRUE ("Stop")] -> w154
              frame False {
              }
              frame True {
                n59 = invoke on="Data Setup Indicator" class="Str" method="Reinit To Default"() -> ()  [unwired: 3 in, 3 out]
                n60 = invoke on="Start Initialization" class="Bool" method="Reinit To Default"() -> ()  [unwired: 3 in, 3 out]
              }
            }
          }
          event Panel Close? {
            n61 = event-data() -> ()  [unwired: 1 in, 4 out]
            n62 = event-data() -> ()  [unwired: 2 in, 1 out]
          }
          event "Stop": Value Change {
            n63 = event-data() -> ()  [unwired: 1 in, 6 out]
            n64 = local read "stop"() -> (w158:bool)
            n65 = case shown="True" w158 {
              selector: w158 -> [w160 _]
              tunnel: [w160 TRUE] -> w159
              tunnel: w158 -> [_ _]
              frame False {
              }
              frame True {
              }
            }
          }
          event "Clear Groundwater Header Values": Value Change {
            n66 = event-data() -> ()  [unwired: 1 in, 6 out]
            n67 = case shown="True" "Clear Groundwater Header Values" {
              tunnel: w162 -> [_ w164]
              frame False {
              }
              frame True {
                n68 = invoke on="Groundwater Header" class="Clust (strict)" method="Reinit To Default"(error in=w164) -> (error out=w165:errorcluster)  [unwired: 2 in, 2 out]
                n69 = flat-sequence {
                  tunnel: w165 -> [_]
                  frame #0 {
                    n70 = local read "Groundwater Header"() -> (w166:T12)
                    n71 = local read "Serial Number/MISC"() -> (w167:string)
                    n72 = Bundle By Name(cluster=w166, "Sonde Serial"=w167) -> (w168:T12)
                    n73 = local write "Groundwater Header"(w168) -> ()
                  }
                }
              }
            }
          }
        }
        n74 = Bundle By Name(cluster=w128, "Date Finished"=w121) -> (w122:T12)
        n75 = Cluster To Array(cluster=w122) -> (array=w127:string[])
        n76 = for {
          tunnel: w127 -> [w145] mode=indexing
          tunnel: [w140] -> w126 mode=indexing
          i -> [w142]
          n77 = call <vilib>:"Trim Whitespace.vi"("string"=w145) -> ("trimmed string"=w144:string)  [unwired: 1 in]
          n78 = Not Equal?(x=w144, y="") -> (x != y?=w141:bool)
          n79 = case shown="1" w142 {
            tunnel: w141 -> [w146 _]
            tunnel: [w146 TRUE] -> w140
            frame 0, Default {
            }
            frame 1 {
            }
          }
        }
        n80 = And Array Elements(Boolean array=w126) -> (logical AND=w118:bool)
        n81 = case shown="True" w118 {
          tunnel: ["  Empty fields in Header not allowed." ""] -> w117
          frame False {
          }
          frame True {
          }
        }
        n82 = Concatenate Strings("Hit the Start Key after Data Entry of Log Parameters and File Names." ("Data Setup Indicator"), w117) -> (→"Data Setup Indicator":string)
        n83 = call <userlib>:"Wait (ms)__ogtk.vi"("error in (no error)"=w129, "milliseconds to wait"=u32 100) -> ("error out"=w130:errorcluster)  [unwired: 8 in, 1 out]
        n84 = Quotient & Remainder(x=w135, y=100) -> (floor(x/y)=w132:i32)  [unwired: 1 out]
        n85 = case shown="1, Default" w132 {
          tunnel: w130 -> [w149 w151]
          frame 1, Default {
            n86 = property on="Data Setup Indicator" class="Str"(error in=w149, "Text.TextColor"=u32 0) -> ()  [unwired: 1 in, 2 out]
          }
          frame 0 {
            n87 = property on="Data Setup Indicator" class="Str"(error in=w151, "Text.TextColor"=u32 16716800) -> ()  [unwired: 1 in, 2 out]
          }
        }
        n88 = local read "stop"() -> (w123:bool)
        n89 = And(x=w118, y=w124) -> (x .and. y?=w125:bool)
        n90 = Compound Arithmetic op=OR(w130, w123, w125) -> (w131:bool)
      }
      n91 = invoke on="stop" class="Bool (strict)" method="Reinit To Default"(error in=w105) -> (error out=w98:errorcluster)  [unwired: 2 in, 2 out]
      n92 = flat-sequence {
        tunnel: w98 -> [w175]
        tunnel: [w169] -> w107
        frame #0 {
          w176 = T26."Disabled and Grayed Out" ("Disabled")
          n93 = local write "KPRO Finish\nIndicator"(FALSE ("KPRO Finish\nIndicator")) -> ()
          n94 = invoke on="Start KPRO" class="Bool" method="Reinit To Default"(error in=w175) -> (error out=w174:errorcluster)  [unwired: 2 in, 2 out]
          n95 = invoke on="Finish Tests" class="Bool" method="Reinit To Default"(error in=w174) -> (error out=w173:errorcluster)  [unwired: 2 in, 2 out]
          n96 = invoke on="Sonde Array Size" class="DigNum (strict)" method="Reinit To Default"() -> ()  [unwired: 3 in, 3 out]
          n97 = invoke on="Increment Depth" class="Bool" method="Reinit To Default"(error in=w173) -> (error out=w172:errorcluster)  [unwired: 2 in, 2 out]
          n98 = property on="Clear Groundwater Header Values" class="Bool"(error in=w172, "DisabledEnum"=w176) -> (error out=w171:errorcluster)  [unwired: 1 in, 1 out]
          n99 = property on="Start Initialization" class="Bool"(error in=w171, "DisabledEnum"=w176) -> (error out=w170:errorcluster)  [unwired: 1 in, 1 out]
          n100 = invoke on="Update Sonde" class="Bool (strict)" method="Reinit To Default"(error in=w170) -> (error out=w169:errorcluster)  [unwired: 2 in, 2 out]
        }
      }
      n101 = flat-sequence {
        tunnel: [w179] -> w110
        tunnel: [w179] -> w109
        tunnel: [w184] -> w106
        tunnel: w107 -> [w183]
        frame #0 {
          n102 = Unbundle By Name("Input Variables and Slopes") -> ("Depth to Water Table"=w189:dbl)
          n103 = local read "Input Depths \nand Parameters Cluster"() -> (w181:T19)
          n104 = Bundle By Name(cluster="Input Variables and Slopes", "Depth to Water Table"=w189) -> (w186:T2)
          n105 = call <vilib>:"Check if File or Folder Exists.vi"("error in (no error)"=w183, "path"="Slopes File Path") -> ("error out"=w182:errorcluster, "file or folder exists?"=w178:bool, "dup path"=w187:path)  [unwired: 7 in]
          n106 = case shown="True" w178 {
            tunnel: w187 -> [_ w205]
            tunnel: w186 -> [w193 w204]
            tunnel: [w193 w203] -> w185
            tunnel: w182 -> [w192 w199]
            tunnel: [w192 w199] -> w184
            frame False {
              n107 = local write "Data Setup Indicator"("Slope file not found." ("Data Setup Indicator")) -> ()
            }
            frame True {
              n108 = call "Get_SLOPE_data_from_file 2016.vi"("Slopes File Path"=w205) -> ("Last Aux 1 Slope"=w198:dbl, "Last_String_Pot_Slope"=w202:dbl, "DHT Offset"=w194:dbl, "DHT Slope"=w195:dbl, "Last_Flow_Slope"=w201:dbl, "Last Aux 2 Slope"=w197:dbl, "Last Aux 3 Slope"=w196:dbl, "Last_Pressure_Slope"=w200:dbl)  [unwired: 6 in, 1 out]
              n109 = Bundle By Name(cluster=w204, "String Pot Slope"=w202, "Flow Slope"=w201, "Up Hole Pressure Slope"=w200, "Aux 1 Slope"=w198, "Aux 2 Slope"=w197, "Aux 3 Slope"=w196, "DH Pressure Trans Slope"=w195, "DH Pressure Offset"=w194) -> (w203:T2)
            }
          }
          n110 = Unbundle By Name(w181) -> ("Feet of Stainless"=w179:i32)
          n111 = Bundle By Name(cluster=w181, "Feet of Stainless"=w179) -> (w180:T19)
          n112 = local write "Input Depths \nand Parameters Cluster"(w180) -> ()
          n113 = local write "Input Variables and Slopes"(w185) -> ()
        }
      }
      n114 = flat-sequence {
        tunnel: [w116] -> w104
        tunnel: [w115] -> w103
        tunnel: [w114] -> w102
        tunnel: [w113] -> w101
        tunnel: [w112] -> w100
        tunnel: [w111] -> w99
        frame #0 {
          n115 = local read "Column of Volume"() -> (w112:i32)
          n116 = local read "NI_report out"() -> (w111:refnum<class "NI_report.lvclass">)
          n117 = local read "Select Worksheet Index"() -> (w116:i32)
          n118 = local read "Number of Sample Sheets"() -> (w114:i32)
          n119 = local read "Columns"() -> (w113:i32[])
          n120 = local read "Worksheet Names"() -> (w115:string[])
        }
      }
    }
  }
  n121 = flat-sequence {
    tunnel: [w209] -> w17
    tunnel: w13 -> [w208]
    tunnel: [w207] -> w4
    frame #0 {
      w206 = Action_Control_1."Init"  # Event
      n122 = while {
        shift-right: [w217] -> w209
        shift-left: w208 -> [w217]
        shift-right: [w212] -> _
        shift-left: w206 -> [w210]
        tunnel: [w218] -> w207
        i -> [w216]
        stop <- w214 stop-if-true
        # "User Interface Producer Loop"
        n123 = First Call?() -> (First Call?: T/F=w211:bool)
        n124 = case shown="False" w211 {
          tunnel: w217 -> [w223 _]
          tunnel: [w221 FALSE ("Boolean")] -> w214
          tunnel: [w220 w415] -> w212
          tunnel: w210 -> [_ w415]
          frame False {
            w219 = Action_Control_1."TimeOut"  # Event
            n125 = event shown="[13] \"Sonde Sample Not Collected\": Value Change" {
              selector: _ -> [_ _ _ _ _ _ _ _ _ _ _ _ _ _ _ _ _ _ _ _]
              dyn-events: _ -> [_ _ _ _ _ _ _ _ _ _ _ _ _ _ _ _ _ _ _ _]
              timeout: 100 -> [_ _ _ _ _ _ _ _ _ _ _ _ _ _ _ _ _ _ _ _]
              tunnel: [w224 w230 w236 w249 w259 w268 w280 w292 w304 w316 w328 w341 w352 w362 w370 w378 w386 w395 w403 _] -> w220
              tunnel: [FALSE w229 w237 w250 w260 w269 w281 w293 w305 w317 w329 w340 w351 w363 w371 w379 w387 w396 w404 _] -> w221
              tunnel: w223 -> [_ w227 w239 w252 _ w271 w283 w295 w307 w319 w331 _ w348 _ _ _ _ _ _ _]
              tunnel: [_ w227 w238 w251 _ w270 w282 w294 w306 w318 w330 _ _ _ _ _ _ _ _ _] -> _
              tunnel: w219 -> [w224 w226 w235 w248 _ w267 w279 w291 w303 w315 w327 w339 w346 w360 w368 w377 w385 w394 w402 _]
              event Timeout {
                n126 = event-data() -> ()  [unwired: 1 in, 3 out]
              }
              event "stop": Value Change {
                n127 = event-data() -> ()  [unwired: 1 in, 6 out]
                n128 = case shown="False" "stop" {
                  tunnel: [w231 w233] -> w230
                  tunnel: [FALSE TRUE] -> w229
                  tunnel: w226 -> [w231 _]
                  frame False {
                  }
                  frame True {
                    w233 = Action_Control_1."Exit"  # Event
                  }
                }
              }
              event "Record DAQ Raw Voltages": Value Change {
                n129 = event-data() -> ()  [unwired: 1 in, 6 out]
                n130 = case shown="False" "Record DAQ Raw Voltages" {
                  tunnel: [w241 w244] -> w236
                  tunnel: [FALSE FALSE ("Boolean")] -> w237
                  tunnel: [w242 w245] -> w238
                  tunnel: w239 -> [w242 w245]
                  tunnel: w235 -> [w241 _]
                  frame False {
                  }
                  frame True {
                    w244 = Action_Control_1."Acq. DAQ data"  # Event
                  }
                }
              }
              event "Record pH Calibration Zero": Value Change {
                n131 = event-data() -> ()  [unwired: 1 in, 6 out]
                n132 = case shown="True" "Record pH Calibration Zero" {
                  tunnel: [w253 w256] -> w249
                  tunnel: [FALSE FALSE ("Boolean")] -> w250
                  tunnel: [w254 w257] -> w251
                  tunnel: w252 -> [w254 w257]
                  tunnel: w248 -> [w253 _]
                  frame False {
                  }
                  frame True {
                    w256 = Action_Control_1."pH Calibration Zero"  # Event
                  }
                }
              }
              event "Create Excel Files": Value Change {
                n133 = event-data() -> ()  [unwired: 1 in, 6 out]
                n134 = case shown="True" "Create Excel Files" {
                  selector: "Create Excel Files" -> [w263 _]
                  tunnel: [w263 TRUE] -> w260
                  tunnel: [w262 w264] -> w259
                  frame False {
                    w262 = Action_Control_1."TimeOut"  # Event
                  }
                  frame True {
                    w264 = Action_Control_1."Create Excel Files"  # Event
                  }
                }
              }
              event "Record pH Calibration Reference": Value Change {
                n135 = event-data() -> ()  [unwired: 1 in, 6 out]
                n136 = case shown="True" "Record pH Calibration Reference" {
                  tunnel: [w272 w275] -> w268
                  tunnel: [FALSE FALSE ("Boolean")] -> w269
                  tunnel: [w273 w276] -> w270
                  tunnel: w271 -> [w273 w276]
                  tunnel: w267 -> [w272 _]
                  frame False {
                  }
                  frame True {
                    w275 = Action_Control_1."pH Calibration Standard"  # Event
                  }
                }
              }
              event "Record ORP Calibration": Value Change {
                n137 = event-data() -> ()  [unwired: 1 in, 6 out]
                n138 = case shown="True" "Record ORP Calibration" {
                  tunnel: [w284 w287] -> w280
                  tunnel: [FALSE FALSE ("Boolean")] -> w281
                  tunnel: [w285 w288] -> w282
                  tunnel: w283 -> [w285 w288]
                  tunnel: w279 -> [w284 _]
                  frame False {
                  }
                  frame True {
                    w287 = Action_Control_1."ORP Calibration Standard"  # Event
                  }
                }
              }
              event "Record Salinity Calibration": Value Change {
                n139 = event-data() -> ()  [unwired: 1 in, 6 out]
                n140 = case shown="True" "Record Salinity Calibration" {
                  tunnel: [w296 w299] -> w292
                  tunnel: [FALSE FALSE ("Boolean")] -> w293
                  tunnel: [w297 w300] -> w294
                  tunnel: w295 -> [w297 w300]
                  tunnel: w291 -> [w296 _]
                  frame False {
                  }
                  frame True {
                    w299 = Action_Control_1."Salinity Calibration Standard"  # Event
                  }
                }
              }
              event "Record DO Calibration": Value Change {
                n141 = event-data() -> ()  [unwired: 1 in, 6 out]
                n142 = case shown="True" "Record DO Calibration" {
                  tunnel: [w308 w311] -> w304
                  tunnel: [FALSE FALSE ("Boolean")] -> w305
                  tunnel: [w309 w312] -> w306
                  tunnel: w307 -> [w309 w312]
                  tunnel: w303 -> [w308 _]
                  frame False {
                  }
                  frame True {
                    w311 = Action_Control_1."DO Calibration Standard"  # Event
                  }
                }
              }
              event "Record  SC Calibration": Value Change {
                n143 = event-data() -> ()  [unwired: 1 in, 6 out]
                n144 = case shown="True" "Record  SC Calibration" {
                  tunnel: [w320 w323] -> w316
                  tunnel: [FALSE FALSE ("Boolean")] -> w317
                  tunnel: [w321 w324] -> w318
                  tunnel: w319 -> [w321 w324]
                  tunnel: w315 -> [w320 _]
                  frame False {
                  }
                  frame True {
                    w323 = Action_Control_1."SC Calibration Standard"  # Event
                  }
                }
              }
              event "Increment Depth": Value Change {
                n145 = event-data() -> ()  [unwired: 1 in, 6 out]
                n146 = case shown="True" "Increment Depth" {
                  tunnel: [w332 w335] -> w328
                  tunnel: [FALSE FALSE ("Boolean")] -> w329
                  tunnel: [w333 w336] -> w330
                  tunnel: w331 -> [w333 w336]
                  tunnel: w327 -> [w332 _]
                  frame False {
                  }
                  frame True {
                    w335 = Action_Control_1."Increment Depth Manually"  # Event
                  }
                }
              }
              event "Record Single Sample": Value Change {
                n147 = event-data() -> ()  [unwired: 1 in, 6 out]
                n148 = case shown="True" "Record Single Sample" {
                  tunnel: [w342 w344] -> w341
                  tunnel: [FALSE FALSE] -> w340
                  tunnel: w339 -> [w342 _]
                  frame False {
                  }
                  frame True {
                    w344 = Action_Control_1."Acq. Single Sonde Point"  # Event
                  }
                }
              }
              event "Write Data to Spreadsheet": Value Change {
                n149 = event-data() -> ("OldVal"=w350:bool, "NewVal"=w353:bool)  [unwired: 1 in, 4 out]
                n150 = Not(x=w350) -> (.not. x?=w349:bool)
                n151 = And(x=w349, y=w353) -> (x .and. y?=w347:bool)
                n152 = case shown="True" w347 {
                  tunnel: [w354 w357] -> w352
                  tunnel: [FALSE FALSE ("Boolean")] -> w351
                  tunnel: [w355 w358] -> _
                  tunnel: w348 -> [w355 w358]
                  tunnel: w346 -> [w354 _]
                  frame False {
                  }
                  frame True {
                    w357 = Action_Control_1."Write Sonde Sample Sheet"  # Event
                  }
                }
              }
              event "Sonde Sample Not Collected": Value Change {
                n153 = event-data() -> ("NewVal"=w361:bool)  [unwired: 1 in, 5 out]
                n154 = case shown="True" w361 {
                  tunnel: [FALSE FALSE] -> w363
                  tunnel: [w364 w366] -> w362
                  tunnel: w360 -> [_ w366]
                  frame True {
                    w364 = Action_Control_1."Sonde Sample Not Collected"  # Event
                  }
                  frame False {
                  }
                }
              }
              event "Record  Sonde Reason": Value Change {
                n155 = event-data() -> ("NewVal"=w369:bool)  [unwired: 1 in, 5 out]
                n156 = case shown="True" w369 {
                  tunnel: [FALSE FALSE] -> w371
                  tunnel: [w372 w374] -> w370
                  tunnel: w368 -> [_ w374]
                  frame True {
                    w372 = Action_Control_1."Record Sonde Reason"  # Event
                  }
                  frame False {
                  }
                }
              }
              event "Start KPRO": Value Change {
                n157 = event-data() -> ()  [unwired: 1 in, 6 out]
                n158 = case shown="True" "Start KPRO" {
                  tunnel: [FALSE FALSE] -> w379
                  tunnel: [w381 w383] -> w378
                  tunnel: w377 -> [_ w383]
                  frame True {
                    w381 = Action_Control_1."Start KPRO Measurements"  # Event
                    n159 = local write "KPRO Finish\nIndicator"(FALSE ("KPRO Finish\nIndicator")) -> ()
                  }
                  frame False {
                  }
                }
              }
              event "Update Depth": Value Change {
                n160 = event-data() -> ()  [unwired: 1 in, 6 out]
                n161 = case shown="True" "Update Depth" {
                  tunnel: [FALSE FALSE] -> w387
                  tunnel: [w389 w391] -> w386
                  tunnel: w385 -> [_ w391]
                  frame True {
                    w389 = Action_Control_1."Update Depth"  # Event
                  }
                  frame False {
                  }
                }
              }
              event "Record IK Reason": Value Change {
                n162 = event-data() -> ()  [unwired: 1 in, 6 out]
                n163 = case shown="True" "Record IK Reason" {
                  tunnel: [FALSE FALSE] -> w396
                  tunnel: [w397 w399] -> w395
                  tunnel: w394 -> [_ w399]
                  frame True {
                    w397 = Action_Control_1."Record IK Reason"  # Event
                  }
                  frame False {
                  }
                }
              }
              event "Finish Tests": Value Change {
                n164 = event-data() -> ()  [unwired: 1 in, 6 out]
                n165 = case shown="True" "Finish Tests" {
                  tunnel: [FALSE FALSE] -> w404
                  tunnel: [w406 w408] -> w403
                  tunnel: w402 -> [_ w408]
                  frame True {
                    w406 = Action_Control_1."Finish KPRO Measurements"  # Event
                    "KPRO Finish\nIndicator" <- TRUE ("KPRO Finish\nIndicator")
                  }
                  frame False {
                  }
                }
              }
              event "Depth mode": Value Change {
                n166 = event-data() -> ()  [unwired: 1 in, 6 out]
                n167 = case shown="True" "Depth mode" {
                  tunnel: [FALSE ("Read String Pot") TRUE ("Read String Pot")] -> w410
                  frame False {
                  }
                  frame True {
                  }
                }
                n168 = local write "Read String Pot"(w410) -> ()
              }
            }
          }
          frame True {
          }
        }
        "Stop" <- w214
        n169 = local read "Stop"() -> (w215:bool)
        n170 = Or(x=w215, y=w214) -> ()  [unwired: 1 out]
        n171 = call <extravilib>:"Write With Abort.vi"("abort"=FALSE, "last element? (F)"=w214, "element"=w212) -> ("channel"=w218:T28)  [unwired: 6 in, 2 out]
        "producer loop" <- w216
      }
    }
  }
  n172 = flat-sequence {
    tunnel: [w441] -> w16
    tunnel: w13 -> [w440]
    tunnel: w12 -> [w417]
    tunnel: w11 -> [w439]
    tunnel: w10 -> [w437]
    tunnel: w9 -> [w436]
    tunnel: w8 -> [w434]
    tunnel: w6 -> [w433]
    tunnel: w4 -> [w432]
    tunnel: w3 -> [w430]
    tunnel: w2 -> [w429]
    tunnel: w1 -> [w428]
    frame #0 {
      w418 = dbl[][] []  # Cumulative Data over 1 string pot
      w419 = dbl[][] []  # Cumulative Sonde  Data Out
      w422 = T7 {"SC Initial "=0.0, "DO Initial "=0.0, "pH Initial  "=0.0, "ORP  Initial"=0.0, "Temp Initial"=0.0, "Salinity Initial "=0.0}  # Sonde Parameters  Initial Values
      w423 = FALSE  # Read String Pot
      w424 = T19 {"Flow"=0.21081600494384767, "Zeroed \nPressure"=74.74207969932556, "Ik"=0.003788962123473114, "Current Depth"=-100.6, "Feet of Stainless"=40, "Start Depth"=0.0, "Abs Start Depth"=0.0}  # Input Depths  and Parameters Cluster
      w425 = T21 {"Absolute Depth In"=0.0, "Current Absolute Depth"=0.0, "First Absolute Depth"=0.0, "Previous Relative Depth"=0.0, "Current Relative Depth"=0.0, "First Relative Depth"=0.0, "Last Filed Depth"=0.0, "Total Volume In"=0.0, "Total Volume Out"=0.0, "Current Measurement Time"=0.0, "Previous Measurement Time"=0.0}  # Depth Cluster
      w426 = dbl[][] []  # Cumulative Data From File
      w427 = dbl[] []  # Time Array
      w435 = cluster{"row":i32, "column":i32} {"row"=0, "column"=0}  # start of last occupied row
      w438 = 0  # row index
      n173 = Get Date/Time In Seconds() -> (seconds since 1Jan1904=w421:timestamp)
      n174 = To Double Precision Float(number=w421) -> (double precision float=w420:dbl)
      n175 = while {
        tunnel: w440 -> [w445]
        tunnel: [w489] -> w441
        tunnel: w432 -> [w469]
        shift-right: [w480] -> _
        shift-left: 1 ("Current Sonde Sample") -> [w444]
        tunnel: w439 -> [w482]
        tunnel: w437 -> [w488]
        tunnel: w436 -> [w487]
        shift-right: [w481] -> _
        shift-left: w438 -> [w486]
        shift-right: [w484] -> _
        shift-left: w435 -> [w483]
        tunnel: w434 -> [w479]
        shift-right: [w475] -> _
        shift-left: w427 -> [w476]
        shift-right: [w474] -> _
        shift-left: w426 -> [w473]
        tunnel: w420 -> [w472]
        tunnel: [w471] -> _
        tunnel: w433 -> [w459]
        shift-right: [w467] -> _
        shift-left: refnum<k24>[] [] -> [w458]
        tunnel: w430 -> [w443]
        shift-right: [w447] -> _
        shift-left: w429 -> [w448]
        shift-right: [w466] -> _
        shift-left: w428 -> [w466]
        shift-right: [w464] -> _
        shift-left: w423 -> [w463]
        shift-right: [w451] -> _
        shift-left: w425 -> [w462]
        shift-right: [w461] -> _
        shift-left: w424 -> [w460]
        shift-right: [w455] -> _
        shift-left: w422 -> [_]
        shift-right: [w453] -> _
        shift-left: w419 -> [w452]
        shift-right: [w450] -> _
        shift-left: w418 -> [w449]
        shift-right: [w485] -> _
        shift-left: w417 -> [w446]
        i -> [w456]
        stop <- w470 stop-if-true
        # "Consumer Data Handling Loop"
        n176 = flat-sequence {
          tunnel: [w493] -> w478
          tunnel: [w492] -> w477
          tunnel: w469 -> [w491]
          tunnel: [w490] -> w468
          frame #0 {
            n177 = call <extravilib>:"Read With Abort.vi"("abort"=FALSE, "channel"=w491) -> ("last element?"=w490:bool, "element"=w493:T27)  [unwired: 5 in, 3 out]
            n178 = feedback #1() -> (w492:T27)  [unwired: 1 in]
            n179 = feedback-in #1(w493) -> ()
          }
        }
        n180 = flat-sequence {
          tunnel: w445 -> [w511]
          tunnel: [w514] -> w465
          tunnel: w444 -> [w506]
          tunnel: w443 -> [w509]
          frame #0 {
            n181 = Get Date/Time In Seconds() -> (seconds since 1Jan1904=w507:timestamp)
            n182 = call <userlib>:"Wait (ms)__ogtk.vi"("error in (no error)"=w511, "milliseconds to wait"=u32 50) -> ("error out"=w510:errorcluster)  [unwired: 8 in, 1 out]
            n183 = Subtract(x=w507, y=w509) -> (x-y=w508:dbl)
            n184 = local write "Current Time (s)"(w508) -> ()
            n185 = call <vilib>:"Clear Errors.vi"("error in (no error)"=w510) -> ("error out"=w513:errorcluster)  [unwired: 5 in, 1 out]
            n186 = local write "Current Sonde Sample"(w506) -> ()
            n187 = Format Into String(format string="Data from Sample %d ", error in=w513, w506) -> (resulting string=→"Table Label":string, error out=w514:errorcluster)  [unwired: 1 in]
          }
        }
        n188 = flat-sequence {
          tunnel: w459 -> [w498]
          tunnel: w458 -> [w497]
          tunnel: [w496] -> w457
          tunnel: w456 -> [w495]
          frame #0 {
            n189 = case shown="1, Default" w495 {
              tunnel: w497 -> [w499 w505]
              tunnel: w498 -> [_ w504]
              tunnel: [w499 w502] -> w496
              frame 0 {
              }
              frame 1, Default {
                n190 = local read "Descriptions"() -> (w503:string[])
                n191 = call "Measure DAQ Voltages.vi"("error in (no error)"=w504, "Descriptions"=w503, "Array in"=w505) -> ("Raw Voltages"=w501:dbl[], "Array out"=w502:refnum<k24>[], "Sensor Cluster"=w500:T11)  [unwired: 6 in]
                n192 = local write "Sensor Voltage Cluster"(w500) -> ()
                n193 = local write "Raw Voltages"(w501) -> ()
              }
            }
            "consumer loop" <- w495
          }
        }
        n194 = case shown="\"Start KPRO Measurements\"" w478 {
          selector: w478 -> [_ _ _ _ _ _ _ _ _ _ _ _ _ _ _ _ _ w2269 _ _ _ _]
          tunnel: w465 -> [w519 w722 w757 w800 w825 w965 w1137 w1154 w1190 w1243 w1274 w1394 w1532 w1685 w1835 w1985 w2129 w2275 w2400 w2849 w2860 w2924]
          tunnel: [w519 w722 w757 w800 w821 w964 w1137 w1154 w1190 w1242 w1272 w1392 w1530 w1683 w1833 w1983 w2127 w2259 w2400 w2849 w2873 w2925] -> w489
          tunnel: w468 -> [_ _ _ _ _ _ _ _ _ _ _ _ _ _ _ _ _ _ _ _ _ _]
          tunnel: w446 -> [w546 w712 w756 w799 w842 w986 w1136 w1153 w1189 w1237 w1281 w1409 w1546 w1698 w1849 w1998 w2142 w2276 w2407 w2848 w2859 _]
          tunnel: [w545 w721 w755 w798 w841 w985 w1135 w1152 w1188 w1236 w1270 w1389 w1527 w1680 w1830 w1980 w2124 w2264 w2406 w2847 w2878 w2941] -> w481
          tunnel: w488 -> [_ _ _ _ _ _ _ _ _ _ w1279 w1407 w1544 w1696 w1847 w1996 w2140 _ _ _ _ _]
          tunnel: w487 -> [_ _ _ _ _ _ _ _ _ _ w1278 w1406 w1543 w1695 w1846 w1995 w2139 _ _ _ _ _]
          tunnel: w486 -> [w545 w721 w755 w798 w841 w985 w1135 w1152 w1188 w1236 w1248 w1390 w1528 w1681 w1831 w1981 w2125 w2253 w2406 w2847 w2878 w2941]
          tunnel: [w546 w712 w756 w799 w842 w986 w1136 w1153 w1189 w1237 w1275 w1395 w1533 w1686 w1836 w1986 w2130 w2274 w2407 w2848 w2879 w2923] -> w485
          tunnel: w444 -> [w544 w720 w754 w797 w829 w970 w1134 w1151 w1187 w1235 w1258 w1403 w1540 w1692 w1843 w1992 w2136 w2271 w2405 w2846 w2877 w2940]
          tunnel: [w544 w720 w754 w797 w829 w970 w1134 w1151 w1187 w1235 w1258 w1403 w1540 w1692 w1843 w1992 w2136 w2270 w2405 w2846 w2877 w2940] -> w480
          tunnel: [w543 w719 w753 w796 w840 w984 w1133 w1150 w1186 w1234 w1271 w1391 w1529 w1682 w1832 w1982 w2126 w2267 w2404 w2845 w2876 w2939] -> w484
          tunnel: w483 -> [w543 w719 w753 w796 w840 w984 w1133 w1150 w1186 w1234 w1250 w1371 w1509 w1660 w1810 w1962 w2106 w2250 w2404 w2845 w2876 w2939]
          tunnel: w482 -> [_ _ _ _ _ _ _ _ _ _ _ _ _ _ _ _ _ w2273 _ _ _ _]
          tunnel: w479 -> [_ _ _ _ _ _ _ _ _ _ _ _ _ _ _ _ _ w2272 _ _ _ _]
          tunnel: w477 -> [_ _ _ _ _ _ _ _ _ _ _ _ _ _ _ _ _ w2268 _ _ _ _]
          tunnel: w476 -> [w532 w718 w752 w795 w839 w983 w1132 w1149 w1185 w1233 w1269 w1388 w1526 w1679 w1829 w1979 w2123 w2263 w2403 w2844 w2875 w2938]
          tunnel: [w531 w718 w752 w795 w839 w983 w1132 w1149 w1185 w1233 w1268 w1387 w1525 w1678 w1828 w1978 w2122 w2263 w2403 w2844 w2875 w2938] -> w475
          tunnel: [w526 w706 w751 w794 w827 w968 w1131 w1148 w1184 w1232 w1246 w1386 w1524 w1668 w1827 w1977 w2121 w2262 w2392 w2843 w2874 w2937] -> w474
          tunnel: w473 -> [w527 w707 w751 w794 w833 w975 w1131 w1148 w1184 w1232 w1246 w1385 w1523 w1668 w1826 w1976 w2120 w2262 w2393 w2843 w2874 w2937]
          tunnel: w472 -> [_ _ _ _ _ _ _ _ _ _ w1257 w1384 w1522 w1677 w1825 w1975 w2119 _ _ _ _ _]
          tunnel: w457 -> [w518 w717 w750 w793 w836 w980 w1130 w1147 w1183 w1231 w1266 w1382 w1520 w1675 w1823 w1973 w2117 w2261 _ w2841 w2868 w2934]
          tunnel: [w542 w716 w749 w792 w815 w963 w1129 w1138 w1182 w1230 w1267 w1383 w1521 w1676 w1824 w1974 w2118 w2260 w2399 _ w2869 w2935] -> w471
          tunnel: w459 -> [w542 w716 w749 w792 w816 w963 w1129 w1139 w1182 w1230 w1267 w1383 w1521 w1676 w1824 w1974 w2118 w2260 w2401 w2840 w2872 w2926]
          tunnel: [_ _ _ _ _ _ _ _ _ _ _ _ _ _ _ _ _ _ FALSE ("aborted?") FALSE ("aborted?") w2871 w2936] -> w470
          tunnel: [w535 w717 w750 w793 w836 w980 w1130 w1147 w1183 w1231 w1266 w1382 w1520 w1675 w1823 w1973 w2117 w2261 w2391 w2839 w2868 w2934] -> w467
          tunnel: [w541 w715 w748 w791 w838 w982 w1128 w1146 w1181 w1229 w1264 w1380 w1518 w1673 w1821 w1971 w2115 w2258 "Read String Pot" w2838 w2867 w2933] -> w464
          tunnel: w463 -> [w541 w715 w748 w791 w838 w982 w1128 w1146 w1181 w1229 w1264 w1380 w1518 w1673 w1821 w1971 w2115 w2258 _ w2838 w2867 w2933]
          tunnel: [w524 w708 w743 w787 w831 w972 w1127 w1145 w1180 w1228 w1263 w1379 w1517 w1672 w1820 w1970 w2114 w2257 w2396 w2837 w2866 w2932] -> w451
          tunnel: w462 -> [w525 w708 w744 w787 w808 w973 w1127 w1145 w1180 w1228 w1263 w1379 w1517 w1672 w1820 w1970 w2114 w2257 w2383 w2837 w2866 w2932]
          tunnel: [w540 w714 w747 w790 w837 w981 w1126 w1144 w1179 w1227 w1262 w1378 w1516 w1671 w1819 w1969 w2113 w2256 w2395 w2836 w2865 w2931] -> w461
          tunnel: w460 -> [w540 w714 w747 w790 w837 w981 w1126 w1144 w1179 w1227 w1262 w1378 w1516 w1671 w1819 w1969 w2113 w2256 _ w2836 w2865 w2931]
          tunnel: [w539 w713 w746 w789 w826 w967 w1125 w1143 w1178 w1226 w1255 w1377 w1515 w1670 w1818 w1968 w2112 w2255 w2387 w2835 w2864 w2930] -> w455
          tunnel: "Sonde Parameters \nInitial Values" -> [w539 w713 w746 w789 w826 w967 w1125 w1143 w1178 w1226 w1260 w1377 w1515 w1670 w1818 w1968 w2112 w2255 w2387 w2835 w2864 w2930]
          tunnel: w448 -> [w521 w710 w745 w788 w824 w957 w1124 w1142 w1177 w1225 w1259 w1376 w1514 w1669 w1817 w1967 w2111 w2254 w2386 w2834 w2863 w2929]
          tunnel: [w520 w709 w745 w788 w803 w958 w1124 w1142 w1177 w1225 w1259 w1376 w1514 w1669 w1817 w1967 w2111 w2254 w2386 w2834 w2863 w2929] -> w447
          tunnel: [w530 w711 w742 w786 w809 w961 w1123 w1141 w1176 w1224 w1256 w1375 w1513 w1667 w1816 w1966 w2110 w2252 w2384 w2833 w2862 w2928] -> w453
          tunnel: w452 -> [w529 w711 w742 w786 w809 w961 w1123 w1141 w1176 w1224 w1256 w1375 w1513 w1666 w1816 w1966 w2110 w2252 w2384 w2833 w2862 w2928]
          tunnel: [w522 w699 w741 w785 w805 w960 w1122 w1140 w1175 w1223 w1254 w1374 w1512 w1665 w1815 w1965 w2109 w2251 w2381 w2832 w2861 w2927] -> w450
          tunnel: w449 -> [w523 w700 w741 w785 w806 w959 w1122 w1140 w1175 w1223 w1254 w1374 w1512 w1665 w1815 w1965 w2109 w2251 w2381 w2832 w2861 w2927]
          frame "TimeOut", Default {
            n195 = flat-sequence {
              tunnel: [w686] -> _
              tunnel: [w690] -> w517
              tunnel: [w698] -> _
              tunnel: [w697] -> _
              tunnel: w518 -> [w696]
              tunnel: [w695] -> _
              frame #0 {
                n196 = local read "Input Variables and Slopes"() -> (w688:T2)
                n197 = local read "Input Variables and Slopes"() -> (w692:T2)
                n198 = local read "Sample Sheet Data Row Cluster 2"() -> (w685:T3)
                n199 = local read "Zero In-Line Pressure\n(F = leave as is)"() -> (w691:bool)
                n200 = Unbundle By Name(w692) -> ("DH Pressure Trans Slope"=w698:dbl, "DH Pressure Offset"=w697:dbl)
                n201 = local read "Sensor Voltage Cluster"() -> (w693:T11)
                n202 = local read "Descriptions"() -> (w694:string[])
                n203 = local read "Sensor  Real \nMeasurements"() -> (w689:T8)
                n204 = global write "Kpro Globals.vi" "Atmospheric Pressure"(0.0 ("Atmospheric Pressure")) -> ()
                n205 = global write "Kpro Globals.vi" "Reservoir Pressure"(0.0 ("Reservoir Pressure")) -> ()
                n206 = global read "Kpro Globals.vi" "Current Depth"() -> (w686:sgl)
                n207 = call "DHT Pressure 2016.vi"("Sensor Cluster"=w693, "DHT Pressure Offset"=w697, "Array in"=w696, "DHT Pressure \nSlope"=w698, "Descriptions"=w694, "Zero Pressure\n(F = leave as is)"=w691) -> ("Array out"=w695:refnum<k24>[], "DHT Pressure (ft/H20)"=w690:dbl, "Sensor Cluster 2"=w687:T11)  [unwired: 6 in, 1 out]
                n208 = local write "Sensor Voltage Cluster"(w687) -> ()
                n209 = call "convert sensor voltage to real measurements.vi"("Input Variables and Slopes"=w688, "Sensor  Real Measurements in"=w689, "Sensor Cluster"=w687) -> ("Sensor  Real Measurements out"=w683:T11)  [unwired: 8 in]
                n210 = Unbundle By Name(w683) -> ("Aux 1"=w682:dbl, "Aux 2"=w681:dbl, "Aux 3"=w680:dbl)
                n211 = Bundle By Name(cluster=w685, "Aux1"=w682, "Aux2"=w681, "Aux3"=w680) -> (w684:T3)
                n212 = local write "Sensor  Real \nMeasurements"(w683) -> ()
                n213 = local write "Down hole Pressure (ft)"(w690) -> ()
                n214 = local write "Sample Sheet Data Row Cluster 2"(w684) -> ()
                n215 = Add(x=w690, y=w686) -> ()  [unwired: 1 out]
              }
            }
            n216 = flat-sequence {
              tunnel: w519 -> [w547]
              frame #0 {
                n217 = property on="Cumulative_data_from_file" class="Arr (strict)"(error in=w547) -> (error out=w548:errorcluster, "Index Values"=w550:u32[])  [unwired: 1 in, 1 out]
                n218 = property on="Current Session" class="Arr (strict)"(error in=w547) -> (error out=w559:errorcluster, "Index Values"=w558:u32[])  [unwired: 1 in, 1 out]
                n219 = Index Array(array=w558, index=1) -> (element=w556:u32)
                n220 = Index Array(array=w550, index=1) -> (element=w552:u32)
                n221 = Build Array(w556, u32 0 ("element")) -> (w555:u32[])
                n222 = Build Array(w552, u32 0 ("element")) -> (w549:u32[])
                n223 = property on="KPRO session report header" class="Arr (strict)"(error in=w559, "Index Values"=w555) -> ()  [unwired: 1 in, 2 out]
                n224 = property on="KPRO Culmulative \ntest report header 2" class="Arr (strict)"(error in=w548, "Index Values"=w549) -> ()  [unwired: 1 in, 2 out]
              }
            }
            n225 = flat-sequence {
              tunnel: w518 -> [_]
              tunnel: w517 -> [_]
              frame #0 {
                n226 = global read "Kpro Globals.vi" "Flow Slope"() -> (→"Flow Slope Global":dbl)
                n227 = global read "Kpro Globals.vi" "Ion Offset"() -> (→"Ion Offset Global":dbl)
                n228 = global read "Kpro Globals.vi" "Profile ID"() -> (→"Profile ID":string)
                n229 = global read "Kpro Globals.vi" "Ion Slope"() -> (→"Ion Slope Global":dbl)
                n230 = global read "Kpro Globals.vi" "Distance"() -> (→"Distance Global":dbl)
                n231 = global read "Kpro Globals.vi" "increment_amount"() -> (→"Increment Global":dbl)
                n232 = global read "Kpro Globals.vi" "KPRO Box Number"() -> (→"KPRO Box Global":dbl)
                n233 = global read "Kpro Globals.vi" "Reservoir Pressure"() -> (→"Reservoir Pressure Global":dbl)
                n234 = global read "Kpro Globals.vi" "String Pot \nSlope"() -> (→"String Pot  Slope Global":dbl)
                n235 = global read "Kpro Globals.vi" "Pressure \nSlope"() -> (→"Pressure Slope Global":dbl)
                n236 = global read "Kpro Globals.vi" "Current Depth"() -> (→"Current Depth Global":sgl)
                n237 = global read "Kpro Globals.vi" "height_of_box"() -> (→"Height of Box Global":dbl)
                n238 = global read "Kpro Globals.vi" "Atmospheric Pressure"() -> (→"Atmospheric Pressure Global":dbl)
                n239 = global read "Kpro Globals.vi" "Depth to Water Table"() -> (→"Depth to Water Table Global":dbl)
              }
            }
            n240 = case shown="True" "Update Sonde" {
              tunnel: w532 -> [w575 w582]
              tunnel: [w575 w581] -> w531
              tunnel: [w574 w580] -> w530
              tunnel: w529 -> [w574 w579]
              frame False {
              }
              frame True {
                n241 = local read "Sonde Communication Error Out"() -> (w578:errorcluster)
                n242 = local read "Current Time (s)"() -> (w576:dbl)
                n243 = flat-sequence {
                  tunnel: w578 -> [w600]
                  tunnel: [w599] -> w577
                  tunnel: w582 -> [w598]
                  tunnel: [w597] -> w581
                  tunnel: [w596] -> w580
                  tunnel: w579 -> [w595]
                  tunnel: [w585] -> _
                  tunnel: [w594] -> _
                  tunnel: w576 -> [w593]
                  frame #0 {
                    n244 = local read "Sample Sheet Data Row Cluster 2"() -> (w586:T3)
                    n245 = control-ref of="Found Quanta Sonde Com Port"() -> (w592:refnum<vi>)
                    n246 = control-ref of="Current Time (s)"() -> (w588:refnum<vi>)
                    n247 = control-ref of="Temperature"() -> (w589:refnum<vi>)
                    n248 = control-ref of="Sonde Data Display"() -> (w591:refnum<vi>)
                    n249 = control-ref of="Sonde Data Display"() -> (w590:refnum<vi>)
                    n250 = Unbundle By Name(w586) -> ("Sonde Data Cluster.Cumulative\nVolume (ml)"=w583:dbl)
                    n251 = call "Sonde Single Measurement Subvi.vi"("VISAResourceName in"=w592, "Time Array"=w598, "Cumulative Sonde Data"=w595, "Previous time"=w593, "Sonde Data Display"=w591, "Sonde Graph in"=w590, "Temp Graph 3"=w589, "error in (no error)"=w600, "Row Cluster Input"=w586, "reference 5"=w588) -> ("seconds since 1Jan1904"=w594:timestamp, "Cumulative Sonde \nData Out"=w596:dbl[][], "Sample Sheet Data Row Cluster 2"=w585:T3, "output cluster"=w587:T4, "time array out"=w597:dbl[], "error out"=w599:errorcluster)
                    n252 = Bundle By Name(cluster=w585, "Sonde Data Cluster.Cumulative\nVolume (ml)"=w583) -> (w584:T3)
                    n253 = local write "Sample Sheet Data Row Cluster 2"(w584) -> ()
                    n254 = local write "output cluster"(w587) -> ()
                  }
                }
                n255 = local write "Sonde Communication Error Out"(w577) -> ()
              }
            }
            n256 = flat-sequence {
              tunnel: w518 -> [w672]
              tunnel: [w668] -> w538
              tunnel: [w667] -> w537
              frame #0 {
                n257 = local read "Input Variables and Slopes"() -> (w675:T2)
                n258 = Unbundle By Name(w675) -> ("Up Hole Pressure Slope"=w674:dbl, "Up Hole  Pressure Offset"=w671:dbl)
                n259 = local write "Input Variables and Slopes"(w675) -> ()
                n260 = local read "Sensor Voltage Cluster"() -> (w676:T11)
                n261 = local read "Descriptions"() -> (w668:string[])
                n262 = local read "Corrected Pressure Cluster"() -> (w670:T1)
                n263 = call "up hole Pressure 2016.vi"("Sensor Cluster"=w676, "Pressure Offset"=w671, "Array in"=w672, "Pressure \nSlope"=w674, "Descriptions"=w668, "Zero Pressure\n(F = leave as is)"=TRUE) -> ("Array out"=w667:refnum<k24>[], "Uphole Pressure"=w666:dbl, "Sensor Cluster 2"=w673:T11)  [unwired: 6 in, 1 out]
                n264 = local write "Corrected\n Pressure (ft)"(w666) -> ()
                n265 = Bundle By Name(cluster=w670, "Up hole Corrected Pressure"=w666) -> (w669:T1)
                n266 = local write "Sensor Voltage Cluster"(w673) -> ()
                n267 = local write "Corrected Pressure Cluster"(w669) -> ()
              }
            }
            n268 = flat-sequence {
              tunnel: w538 -> [w659]
              tunnel: w537 -> [w662]
              tunnel: [w658] -> w534
              tunnel: [w659] -> w536
              tunnel: [w655] -> w533
              tunnel: [w657] -> w535
              frame #0 {
                w663 = 0.0  # Offset
                n269 = local read "Input Variables and Slopes"() -> (w661:T2)
                n270 = local read "Input Depths \nand Parameters Cluster"() -> (w654:T19)
                n271 = Unbundle By Name(w661) -> ("Flow Slope"=w660:dbl)
                n272 = local read "Input Depths \nand Parameters Cluster"() -> (w665:T19)
                n273 = Unbundle By Name(w654) -> ("Feet of Stainless"=w653:i32)
                n274 = call "Flow 2016.vi"("Descriptions"=w659, "Array in"=w662, "Flow Slope"=w660, "Offset"=w663) -> ("Sensor Cluster"=w658:T11, "Flow (ml/min)"=w655:dbl, "Array out"=w657:refnum<k24>[])  [unwired: 4 in]
                n275 = local write "Sensor Voltage Cluster"(w658) -> ()
                n276 = call "pressure and IK2 2016.vi"("Ft. of SS"=w653, "flow"=w655) -> ("IK"=→"Large Depth IK Graph":dbl)  [unwired: 1 in, 1 out]
                n277 = Bundle By Name(cluster=w665, "Flow"=w655) -> (w664:T19)
                n278 = local write "Input Depths \nand Parameters Cluster"(w664) -> ()
              }
            }
            n279 = flat-sequence {
              tunnel: w536 -> [w641]
              tunnel: w527 -> [w620]
              tunnel: w534 -> [w640]
              tunnel: w525 -> [w625]
              tunnel: [w639] -> w524
              tunnel: w533 -> [w638]
              tunnel: w535 -> [w632]
              tunnel: [w631] -> _
              tunnel: [w612] -> w526
              tunnel: w517 -> [w617]
              tunnel: w519 -> [w614]
              tunnel: w523 -> [w613]
              tunnel: [w610] -> w522
              tunnel: w521 -> [w607]
              tunnel: [w606] -> w520
              frame #0 {
                # "Timeout"
                n280 = Unbundle By Name(w625) -> ("Current Relative Depth"=w624:dbl)
                n281 = local read "Input Depths \nand Parameters Cluster"() -> (w635:T19)
                n282 = local read "Culmulative Graph Cluster"() -> (w630:T24)
                n283 = local read "Depth mode"() -> (w622:bool)
                n284 = local read "Input Variables and Slopes"() -> (w637:T2)
                n285 = local read "KPRO Finish\nIndicator"() -> (w619:bool)
                n286 = local read "Sensor Voltage Cluster"() -> (w603:T11)
                n287 = local read "Sensor  Real \nMeasurements"() -> (w604:T8)
                n288 = Unbundle By Name(w637) -> ("String Pot Slope"=w636:dbl)
                n289 = Unbundle By Name(w635) -> ()  [unwired: 1 out]
                n290 = Unbundle By Name(w603) -> ("Downhole Pressure"=w601:dbl)
                n291 = Unbundle By Name(w604) -> ("Downhole Pressure"=w602:dbl)
                n292 = local write "Corrected\n Pressure (ft)"(w602) -> ()
                n293 = call "Kpro Read String Pot 2016.vi"("Read String Pot"=w622, "Feet of\nStainless to be\nUsed (Count) in"=w607, "Session Array in"=w613, "Flow"=w638, "Manual Depth In"=w624, "Finished In"=w619, "Depth Cluster in"=w625, "error in (no error)"=w614, "String Pot \nSlope in"=w636, "Sensor Cluster In in"=w640, "Descriptions"=w641, "Pressure in"=w602, "Array in"=w632, "Downhole Pressure Sensor"=w617, "Initial Measurement Input"=FALSE, "Downhole Pressure (V)"=w601) -> ("Sensor Cluster 2"=w633:T11, "IK"=w616:dbl, "Array out"=w631:refnum<k24>[], "Generate Array Calc IK"=w621:bool, "Feet of\nStainless to be\nUsed (Count) out"=w606:i32, "Depth Cluster out"=w639:T21, "Single String Pot Session Array out"=w610:dbl[][])  [unwired: 3 in, 2 out]
                n294 = local write "Ik"(w616) -> ()
                n295 = local write "Sensor Voltage Cluster"(w633) -> ()
                n296 = Unbundle By Name(w639) -> ("Current Absolute Depth"=w623:dbl)
                n297 = And(x=w621, y=w622) -> ()  [unwired: 1 out]
                n298 = Bundle By Name(cluster=w635, "Feet of Stainless"=w606) -> (w634:T19)
                n299 = local write "Input Depths \nand Parameters Cluster"(w634) -> ()
                n300 = flat-sequence {
                  tunnel: w623 -> [w647]
                  frame #0 {
                    n301 = global write "Kpro Globals.vi" "Current Depth"(w647) -> ()
                    n302 = local write "Current Depth"(w647) -> ()
                    n303 = Divide(x=w647, y=3.281) -> (x/y=w648:dbl)
                    n304 = local read "Sample Sheet Data Row Cluster 2"() -> (w651:T3)
                    n305 = local read "Corrected Pressure Cluster"() -> (w649:T1)
                    n306 = Unbundle By Name(w649) -> ("Up hole Corrected Pressure"=w646:dbl)
                    "Corrected\n Pressure (ft)" <- w646
                    n307 = Bundle By Name(cluster=w651, "Depth"=w647, "Head\nPressure"=w646) -> (w650:T3)
                    n308 = local write "Sample Sheet Data Row Cluster 2"(w650) -> ()
                    n309 = local write "Current \nDepth (m)"(w648) -> ()
                  }
                }
                n310 = case shown="True" FALSE {
                  tunnel: w620 -> [w642 w645]
                  tunnel: w610 -> [_ w643]
                  tunnel: [w642 w644] -> w612
                  frame False {
                  }
                  frame True {
                    n311 = Build Array (concatenate)(w645, w643) -> (w644:dbl[][])
                  }
                }
                n312 = call "Array to Plot 2016.vi"("Input Cumulative Array"=w612, "Input Real Time Array"=w610) -> ("Cumulative - Depth vs.Drive Rate"=w608:cluster{dbl[], dbl[]}, "Cumulative - Depth vs. Ik"=w628:cluster{dbl[], dbl[]}, "Real Time - Depth vs. Drive Rate"=w609:cluster{dbl[], dbl[]}, "Real Time - Depth vs. Ik"=w618:cluster{dbl[], dbl[]}, "Depth Rate"=w615:dbl)  [unwired: 2 in, 1 out]
                n313 = Bundle By Name(cluster=w630, "Cumulative - Depth vs. Ik"=w628, "Real Time - Depth vs. lk"=w618, "Cumulative - Depth vs. Drive Rate"=w608, "Real Time - Depth vs. Drive Rate"=w609) -> (w629:T24)
                n314 = local write "Large Depth IK Graph Cluster"(w618) -> ()
                n315 = local write "Culmulative Graph Cluster"(w629) -> ()
                n316 = local write "Depth Rate\nft/min"(w615) -> ()
                n317 = local write "Current Session"(w610) -> ()
                n318 = local read "Input Depths \nand Parameters Cluster"() -> (w627:T19)
                n319 = local write "Cumulative_data_from_file"(w612) -> ()
                n320 = Unbundle By Name(w627) -> ("Flow"=→"Flow":dbl)
              }
            }
          }
          frame "Finish KPRO Measurements" {
            w705 = T26."Enabled" ("Disabled")
            n321 = property on="Start KPRO" class="Bool"("DisabledEnum"=w705) -> ()  [unwired: 2 in, 2 out]
            n322 = property on="stop" class="Bool (strict)"("DisabledEnum"=w705) -> ()  [unwired: 2 in, 2 out]
            n323 = flat-sequence {
              tunnel: w708 -> [w728]
              tunnel: w707 -> [w732]
              tunnel: w700 -> [w730]
              tunnel: w710 -> [w729]
              tunnel: [w726] -> w709
              tunnel: [w735] -> w704
              tunnel: [w727] -> w703
              tunnel: w704 -> [w737]
              tunnel: w703 -> [w736]
              tunnel: [w737] -> w702
              tunnel: [w736] -> w701
              tunnel: [w739] -> _
              tunnel: [w740] -> w706
              tunnel: w702 -> [w740]
              tunnel: w701 -> [w739]
              tunnel: [w738] -> w699
              frame #0 {
                n324 = local read "Input Depths \nand Parameters Cluster"() -> (w734:T19)
                n325 = local read "KPRO Cumulative Output File Path"() -> (w723:path)
                n326 = Build Array (concatenate)(w732, w730) -> (w731:dbl[][])
                n327 = local read "KPRO Culmulative \ntest report header 2"() -> (w725:T20)
                n328 = call "Finished Collection Write File.vi"("Replace File"=TRUE, "Cluster in"=w728, "KPRO Culmulative \ntest report header 2"=w725, "Corrected Array in"=w731, "Feet of\nStainless to be\nUsed (Count) in"=w729, "Output KPRO"=w723) -> ("Corrected Array out"=w735:dbl[][], "Depth to \nbe Used \n(Feet)"=w727:sgl, "Feet of\nStainless to be\nUsed (Count) out"=w726:i32)  [unwired: 3 in]
                n329 = Bundle By Name(cluster=w734, "Feet of Stainless"=w726) -> (w733:T19)
                n330 = local write "Current Depth"(w727) -> ()
                n331 = local write "Input Depths \nand Parameters Cluster"(w733) -> ()
              }
              frame #1 {
                n332 = invoke on="Current Session" class="Arr (strict)" method="Reinit To Default"() -> ()  [unwired: 3 in, 3 out]
              }
              frame #2 {
                n333 = local read "Current Session"() -> (w738:sgl[][])
              }
            }
          }
          frame "Update Depth" {
            n334 = flat-sequence {
              tunnel: w744 -> [w769]
              tunnel: [w766] -> w743
              frame #0 {
                n335 = Unbundle By Name(w769) -> ("First Absolute Depth"=w767:dbl)
                n336 = local read "Current Depth"() -> (w763:sgl)
                n337 = local read "Sensor  Real \nMeasurements"() -> (w770:T8)
                n338 = Greater?(x="New Depth", y=w763) -> (0:w762:bool)
                n339 = case shown="False" w762 {
                  tunnel: [w779 w784] -> w768
                  tunnel: w767 -> [w778 w783]
                  tunnel: "New Depth" -> [w776 w781]
                  tunnel: w763 -> [w775 w780]
                  frame True {
                    n340 = Subtract(x=w775, y=w776) -> (x-y=w777:dbl)
                    n341 = Subtract(x=w778, y=w777) -> (x-y=w779:dbl)
                  }
                  frame False {
                    # "Reverse inputs \non Subtraction"
                    n342 = Subtract(x=w781, y=w780) -> (x-y=w782:dbl)
                    n343 = Subtract(x=w783, y=w782) -> (x-y=w784:dbl)
                  }
                }
                n344 = Unbundle By Name(w770) -> ("String Pot"=w759:dbl)
                n345 = Bundle By Name(cluster=w769, "Absolute Depth In"="New Depth", "Current Absolute Depth"="New Depth", "First Absolute Depth"=w768) -> (w761:T21)
                n346 = local read "Read String Pot"() -> (w758:bool)
                n347 = case shown="True" w758 {
                  tunnel: w761 -> [w771 w774]
                  tunnel: [w771 w773] -> w760
                  tunnel: w759 -> [_ w772]
                  frame False {
                  }
                  frame True {
                    n348 = Bundle By Name(cluster=w774, "Current Relative Depth"=w772) -> (w773:T21)
                  }
                }
                n349 = call "calculate current depth.vi"("Cluster in"=w760) -> ("Cluster out"=w766:T21)  [unwired: 10 in]
                n350 = Unbundle By Name(w766) -> ("Current Absolute Depth"=w765:dbl)
                n351 = local write "Current Depth"(w765) -> ()
                n352 = global write "Kpro Globals.vi" "Current Depth"(w765) -> ()
              }
            }
          }
          frame "IK vs Time" {
          }
          frame "Start KPRO Measurements" {
            n353 = flat-sequence {
              tunnel: w825 -> [w853]
              tunnel: w824 -> [w852]
              tunnel: [w851] -> w823
              tunnel: [w850] -> w822
              tunnel: [w847] -> w804
              frame #0 {
                n354 = local read "Input Variables and Slopes"() -> (w845:T2)
                n355 = Unbundle By Name(w845) -> ("Depth to Water Table"=w846:dbl)
                n356 = local read "Input Depths \nand Parameters Cluster"() -> (w849:T19)
                n357 = call <vilib>:"Clear Errors.vi"("error in (no error)"=w853) -> ("error out"=w844:errorcluster)  [unwired: 5 in, 1 out]
                n358 = call "New Stainless Correction Pop Up 2016.vi"("error in (no error)"=w844, "New Feet\n of Stainless\n(Count)"=w852, "Depth to \nWater Table\nInput"=w846) -> ("error in (no error) 2"=w850:errorcluster, "Feet of\nStainless to be\nUsed (Count)"=w847:i32, "Depth to \nWater Table\nOutput"=w843:dbl)  [unwired: 6 in]
                n359 = local write "Depth to Water"(w843) -> ()
                n360 = Bundle By Name(cluster=w845, "Depth to Water Table"=w843) -> (w851:T2)
                n361 = Bundle By Name(cluster=w849, "Feet of Stainless"=w847) -> (w848:T19)
                n362 = local write "Input Depths \nand Parameters Cluster"(w848) -> ()
              }
            }
            n363 = flat-sequence {
              tunnel: w836 -> [w882]
              tunnel: [w881] -> w835
              tunnel: w823 -> [w880]
              tunnel: w822 -> [w879]
              tunnel: [w878] -> w821
              tunnel: [w870] -> w820
              tunnel: [w866] -> w802
              frame #0 {
                w868 = T26."Disabled and Grayed Out" ("Disabled")
                n364 = control-ref of="Input Variables and Slopes"() -> (w867:refnum<vi>)
                n365 = control-ref of="Sensor Voltage Cluster"() -> (w874:refnum<vi>)
                n366 = control-ref of="Zero In-Line Pressure\n(F = leave as is)"() -> (w873:refnum<vi>)
                n367 = control-ref of="Output File Path"() -> (w876:refnum<vi>)
                n368 = control-ref of="Descriptions"() -> (w875:refnum<vi>)
                n369 = call "measure down hole pressure and save to csv file.vi"("Path in"=w876, "reference 3"=w875, "Input Variables and Slopes Reference"=w867, "reference 4"=w874, "reference 5"=w873, "Record DTW File"="Record DTW File", "error in (no error)"=w879, "Array in"=w882, "Input Variables and Slopes"=w880) -> ("Array out"=w881:refnum<k24>[], "Down Hole Pressure\n(ft/H20)"=w870:dbl, "DHT Pressure (V)"=w866:dbl, "error out"=w878:errorcluster)  [unwired: 2 in, 1 out]
                "Down hole Pressure (ft)" <- w870
                n370 = local read "Corrected Pressure Cluster"() -> (w872:T1)
                n371 = property on="Start KPRO" class="Bool"("DisabledEnum"=w868) -> ()  [unwired: 2 in, 2 out]
                n372 = property on="stop" class="Bool (strict)"("DisabledEnum"=w868) -> ()  [unwired: 2 in, 2 out]
                n373 = Bundle By Name(cluster=w872, "Down hole Corrected Pressure"=w870) -> (w871:T1)
                n374 = invoke on="Update Sonde" class="Bool (strict)" method="Reinit To Default"() -> ()  [unwired: 3 in, 3 out]
                n375 = local write "Corrected Pressure Cluster"(w871) -> ()
                n376 = property on="Large Depth IK Graph" class="WFChart (strict)"("History Data"=dbl[] []) -> ()  [unwired: 2 in, 2 out]
              }
            }
            n377 = control-ref of="Input Variables and Slopes"() -> ()  [unwired: 1 out]
            n378 = flat-sequence {
              tunnel: w835 -> [w951]
              tunnel: [w947] -> w819
              tunnel: [w946] -> w818
              tunnel: [w945] -> w801
              frame #0 {
                n379 = local read "Input Variables and Slopes"() -> (w954:T2)
                n380 = Unbundle By Name(w954) -> ("Up Hole Pressure Slope"=w953:dbl, "Up Hole  Pressure Offset"=w950:dbl)
                n381 = local write "Input Variables and Slopes"(w954) -> ()
                n382 = local read "Sensor Voltage Cluster"() -> (w955:T11)
                n383 = local read "Descriptions"() -> (w947:string[])
                n384 = local read "Corrected Pressure Cluster"() -> (w949:T1)
                n385 = call "up hole Pressure 2016.vi"("Sensor Cluster"=w955, "Pressure Offset"=w950, "Array in"=w951, "Pressure \nSlope"=w953, "Descriptions"=w947, "Zero Pressure\n(F = leave as is)"=TRUE) -> ("Array out"=w946:refnum<k24>[], "Uphole Pressure"=w945:dbl, "Sensor Cluster 2"=w952:T11)  [unwired: 6 in, 1 out]
                n386 = Bundle By Name(cluster=w949, "Up hole Corrected Pressure"=w945) -> (w948:T1)
                n387 = local write "Sensor Voltage Cluster"(w952) -> ()
                n388 = local write "Corrected Pressure Cluster"(w948) -> ()
                n389 = local write "Corrected\n Pressure (ft)"(w945) -> ()
              }
            }
            n390 = local read "Input Variables and Slopes"() -> (w814:T2)
            n391 = Unbundle By Name(w814) -> ("String Pot Slope"=w813:dbl)
            n392 = call "depth read from string pot 2016.vi"("Descriptions"=w819, "error in (no error)"=w816, "String Pot \nSlope"=w813, "Array in"=w818) -> ("Array out"=w817:refnum<k24>[], "Depth"=w811:dbl, "error out"=w815:errorcluster)  [unwired: 12 in, 1 out]
            n393 = flat-sequence {
              tunnel: w811 -> [w855]
              tunnel: [w854] -> w810
              frame #0 {
                w856 = 15  # Filter Size
                # "Functional Global in \nBoxcar Integrator\nInitialize filter array to \ncurrent string pot value"
                n394 = call "Boxcar filter2016.vi"("Initialize"=TRUE, "Filter Size"=w856, "Filter Input"=w855) -> ("Filter Output"=w854:dbl)
              }
            }
            n395 = flat-sequence {
              tunnel: [w858] -> w812
              frame #0 {
                n396 = Tick Count (ms)() -> (millisecond timer value=w860:u32)
                n397 = Divide(x=w860, y=u32 1000) -> (x/y=w858:dbl)
              }
            }
            n398 = flat-sequence {
              tunnel: [w865] -> w807
              tunnel: w810 -> [w862]
              tunnel: w812 -> [w864]
              tunnel: w808 -> [w863]
              frame #0 {
                n399 = local read "Current Depth"() -> (w861:sgl)
                n400 = Bundle By Name(cluster=w863, "Previous Relative Depth"=w862, "Current Relative Depth"=w862, "First Relative Depth"=w862, "Current Measurement Time"=w864, "Previous Measurement Time"=w864, "Absolute Depth In"=w861, "Current Absolute Depth"=w861, "First Absolute Depth"=w861) -> (w865:T21)
              }
            }
            n401 = flat-sequence {
              tunnel: w819 -> [w938]
              tunnel: w817 -> [w941]
              tunnel: [w936] -> w832
              tunnel: [w938] -> w834
              tunnel: [w937] -> w830
              tunnel: [w935] -> w828
              frame #0 {
                w942 = 0.0  # Offset
                n402 = local read "Input Variables and Slopes"() -> (w940:T2)
                n403 = Unbundle By Name(w940) -> ("Flow Slope"=w939:dbl)
                n404 = local read "Input Depths \nand Parameters Cluster"() -> (w944:T19)
                n405 = call "Flow 2016.vi"("Descriptions"=w938, "Array in"=w941, "Flow Slope"=w939, "Offset"=w942) -> ("Sensor Cluster"=w936:T11, "Flow (ml/min)"=w937:dbl, "Array out"=w935:refnum<k24>[])  [unwired: 4 in]
                n406 = local write "Sensor Voltage Cluster"(w936) -> ()
                n407 = Bundle By Name(cluster=w944, "Flow"=w937) -> (w943:T19)
                n408 = local write "Input Depths \nand Parameters Cluster"(w943) -> ()
              }
            }
            n409 = flat-sequence {
              tunnel: w834 -> [w920]
              tunnel: w833 -> [w902]
              tunnel: w832 -> [w919]
              tunnel: w807 -> [w918]
              tunnel: [w917] -> w831
              tunnel: w830 -> [w916]
              tunnel: w828 -> [w910]
              tunnel: [w909] -> _
              tunnel: [w893] -> w827
              tunnel: w820 -> [w884]
              tunnel: w806 -> [w897]
              tunnel: [w894] -> w805
              tunnel: w804 -> [w890]
              tunnel: [w889] -> w803
              tunnel: w802 -> [w885]
              tunnel: w801 -> [w883]
              frame #0 {
                n410 = local read "Sensor  Real \nMeasurements"() -> (w886:T8)
                n411 = local read "Culmulative Graph Cluster"() -> (w908:T24)
                n412 = local read "Input Depths \nand Parameters Cluster"() -> (w913:T19)
                n413 = Unbundle By Name(w886) -> ()  [unwired: 1 out]
                n414 = local read "Input Variables and Slopes"() -> (w915:T2)
                n415 = local read "KPRO Finish\nIndicator"() -> (w905:bool)
                n416 = local read "Depth mode"() -> (w903:bool)
                n417 = Unbundle By Name(w915) -> ("String Pot Slope"=w914:dbl)
                n418 = Unbundle By Name(w913) -> ()  [unwired: 1 out]
                n419 = call "Kpro Read String Pot 2016.vi"("Read String Pot"=w903, "Feet of\nStainless to be\nUsed (Count) in"=w890, "Session Array in"=dbl[][] [], "Flow"=w916, "Finished In"=w905, "Depth Cluster in"=w918, "String Pot \nSlope in"=w914, "Sensor Cluster In in"=w919, "Descriptions"=w920, "Pressure in"=w883, "Array in"=w910, "Downhole Pressure Sensor"=w884, "Initial Measurement Input"=TRUE, "Downhole Pressure (V)"=w885) -> ("Sensor Cluster 2"=w911:T11, "Array out"=w909:refnum<k24>[], "Generate Array Calc IK"=w895:bool, "Feet of\nStainless to be\nUsed (Count) out"=w889:i32, "Depth Cluster out"=w917:T21, "Single String Pot Session Array out"=w894:dbl[][])  [unwired: 5 in, 3 out]
                n420 = local write "Current Session"(w894) -> ()
                n421 = Build Array (concatenate)(w902, w897) -> (w898:dbl[][])
                n422 = local write "Sensor Voltage Cluster"(w911) -> ()
                n423 = Unbundle By Name(w917) -> ("Current Absolute Depth"=w901:dbl)
                n424 = Bundle By Name(cluster=w913, "Feet of Stainless"=w889) -> (w912:T19)
                n425 = local write "Input Depths \nand Parameters Cluster"(w912) -> ()
                n426 = flat-sequence {
                  tunnel: w901 -> [w928]
                  frame #0 {
                    n427 = global write "Kpro Globals.vi" "Current Depth"(w928) -> ()
                    n428 = local write "Current Depth"(w928) -> ()
                    n429 = Divide(x=w928, y=3.281) -> (x/y=w929:dbl)
                    n430 = local read "Sample Sheet Data Row Cluster 2"() -> (w933:T3)
                    n431 = local read "Corrected Pressure Cluster"() -> (w931:T1)
                    n432 = Unbundle By Name(w931) -> ("Up hole Corrected Pressure"=w930:dbl)
                    n433 = Bundle By Name(cluster=w933, "Depth"=w928, "Head\nPressure"=w930) -> (w932:T3)
                    n434 = local write "Sample Sheet Data Row Cluster 2"(w932) -> ()
                    n435 = local write "Current \nDepth (m)"(w929) -> ()
                  }
                }
                n436 = case shown="True" FALSE {
                  tunnel: w894 -> [_ w927]
                  tunnel: [w924 w926] -> w893
                  tunnel: w898 -> [w924 w925]
                  frame False {
                  }
                  frame True {
                    n437 = Build Array (concatenate)(w925, w927) -> (w926:dbl[][])
                  }
                }
                n438 = call "Array to Plot 2016.vi"("Input Cumulative Array"=w893, "Input Real Time Array"=w894) -> ("Cumulative - Depth vs.Drive Rate"=w892:cluster{dbl[], dbl[]}, "Cumulative - Depth vs. Ik"=w906:cluster{dbl[], dbl[]}, "Real Time - Depth vs. Drive Rate"=w891:cluster{dbl[], dbl[]}, "Real Time - Depth vs. Ik"=w904:cluster{dbl[], dbl[]}, "Depth Rate"=w900:dbl)  [unwired: 2 in, 1 out]
                n439 = Bundle By Name(cluster=w908, "Cumulative - Depth vs. Ik"=w906, "Real Time - Depth vs. lk"=w904, "Cumulative - Depth vs. Drive Rate"=w892, "Real Time - Depth vs. Drive Rate"=w891) -> (w907:T24)
                n440 = local write "Culmulative Graph Cluster"(w907) -> ()
                n441 = local write "Large Depth IK Graph Cluster"(w904) -> ()
                n442 = local write "Depth Rate\nft/min"(w900) -> ()
                n443 = local write "Cumulative_data_from_file"(w893) -> ()
                n444 = case shown="True" FALSE {
                  tunnel: w895 -> [_ w922]
                  tunnel: w893 -> [_ w921]
                  frame False {
                  }
                  frame True {
                    n445 = control-ref of="KPRO SessionOutput File Path"() -> (w923:refnum<vi>)
                    n446 = call "write KPRO file.vi"("Corrected Array in"=w921, "Generate Array Calc IK"=w922, "Path in"=w923) -> ()  [unwired: 7 in, 2 out]
                  }
                }
              }
            }
          }
          frame "Increment Depth Manually" {
            n447 = local read "Input Variables and Slopes"() -> (w966:T2)
            n448 = flat-sequence {
              tunnel: w980 -> [w1089]
              tunnel: [w1088] -> w979
              tunnel: w966 -> [w1087]
              tunnel: w965 -> [w1086]
              tunnel: [w1085] -> w964
              tunnel: [w1081] -> w962
              frame #0 {
                n449 = flat-sequence {
                  tunnel: [w1106] -> w1094
                  tunnel: [w1095] -> w1093
                  tunnel: [w1105] -> w1092
                  tunnel: [w1104] -> w1091
                  tunnel: [w1103] -> w1090
                  tunnel: w1089 -> [w1102]
                  tunnel: [w1101] -> w1088
                  tunnel: w1087 -> [w1097]
                  tunnel: [w1095] -> w1081
                  frame #0 {
                    n450 = local read "Zero In-Line Pressure\n(F = leave as is)"() -> (w1096:bool)
                    n451 = Unbundle By Name(w1097) -> ("DH Pressure Trans Slope"=w1104:dbl, "DH Pressure Offset"=w1103:dbl)
                    n452 = local read "Sensor Voltage Cluster"() -> (w1099:T11)
                    n453 = local write "Input Variables and Slopes"(w1097) -> ()
                    n454 = local read "Descriptions"() -> (w1100:string[])
                    n455 = global read "Kpro Globals.vi" "Current Depth"() -> (w1106:sgl)
                    n456 = call "DHT Pressure 2016.vi"("Sensor Cluster"=w1099, "DHT Pressure Offset"=w1103, "Array in"=w1102, "DHT Pressure \nSlope"=w1104, "Descriptions"=w1100, "Zero Pressure\n(F = leave as is)"=w1096) -> ("Array out"=w1101:refnum<k24>[], "DHT Pressure (ft/H20)"=w1105:dbl, "Sensor Cluster 2"=w1098:T11)  [unwired: 6 in, 1 out]
                    n457 = local write "Sensor Voltage Cluster"(w1098) -> ()
                    n458 = Add(x=w1105, y=w1106) -> (x+y=w1095:dbl)
                    n459 = local write "Down hole Pressure (ft)"(w1095) -> ()
                  }
                }
                n460 = local read "Record DTW File"() -> (w1084:bool)
                n461 = case shown="True" w1084 {
                  selector: w1084 -> [w1108 _]
                  tunnel: [w1108 FALSE ("Boolean")] -> _
                  tunnel: w1093 -> [_ w1116]
                  tunnel: w1094 -> [_ w1117]
                  tunnel: w1090 -> [_ w1114]
                  tunnel: w1092 -> [_ w1115]
                  tunnel: w1091 -> [_ w1113]
                  tunnel: w1086 -> [w1107 w1112]
                  tunnel: [w1107 w1111] -> w1085
                  frame False {
                  }
                  frame True {
                    n462 = Build Array(w1117, w1116, w1115, w1114, w1113) -> (w1120:dbl[])
                    n463 = local read "Down hole Pressure Transducer CSV data  path"() -> (w1109:path)
                    n464 = call-poly <vilib>:"Write Delimited Spreadsheet.vi"("file path (dialog if empty)"=w1109, "1D data"=w1120, "append to file? (new file:F)"=TRUE, "error in (no error)"=w1112, "delimiter (\\t)"="," ("delimiter (\\t)")) -> ("error out"=w1111:errorcluster)  [unwired: 9 in, 1 out]
                  }
                }
                n465 = local read "Corrected Pressure Cluster"() -> (w1082:T1)
                n466 = Bundle By Name(cluster=w1082, "Down hole Corrected Pressure"=w1081) -> (w1083:T1)
                n467 = local write "Corrected Pressure Cluster"(w1083) -> ()
              }
            }
            n468 = flat-sequence {
              tunnel: w979 -> [w1075]
              tunnel: [w1071] -> w978
              tunnel: [w1070] -> w977
              frame #0 {
                n469 = local read "Input Variables and Slopes"() -> (w1078:T2)
                n470 = Unbundle By Name(w1078) -> ("Up Hole Pressure Slope"=w1077:dbl, "Up Hole  Pressure Offset"=w1074:dbl)
                n471 = local write "Input Variables and Slopes"(w1078) -> ()
                n472 = local read "Sensor Voltage Cluster"() -> (w1079:T11)
                n473 = local read "Descriptions"() -> (w1071:string[])
                n474 = local read "Corrected Pressure Cluster"() -> (w1073:T1)
                n475 = call "up hole Pressure 2016.vi"("Sensor Cluster"=w1079, "Pressure Offset"=w1074, "Array in"=w1075, "Pressure \nSlope"=w1077, "Descriptions"=w1071, "Zero Pressure\n(F = leave as is)"=TRUE) -> ("Array out"=w1070:refnum<k24>[], "Uphole Pressure"=w1069:dbl, "Sensor Cluster 2"=w1076:T11)  [unwired: 6 in, 1 out]
                n476 = Bundle By Name(cluster=w1073, "Up hole Corrected Pressure"=w1069) -> (w1072:T1)
                n477 = local write "Sensor Voltage Cluster"(w1076) -> ()
                n478 = local write "Corrected Pressure Cluster"(w1072) -> ()
                n479 = local write "Corrected\n Pressure (ft)"(w1069) -> ()
              }
            }
            n480 = flat-sequence {
              tunnel: w978 -> [w1062]
              tunnel: w977 -> [w1065]
              tunnel: [w1060] -> w974
              tunnel: [w1062] -> w976
              tunnel: [w1061] -> w971
              tunnel: [w1059] -> w969
              frame #0 {
                w1066 = 0.0  # Offset
                n481 = local read "Input Variables and Slopes"() -> (w1064:T2)
                n482 = Unbundle By Name(w1064) -> ("Flow Slope"=w1063:dbl)
                n483 = local read "Input Depths \nand Parameters Cluster"() -> (w1068:T19)
                n484 = call "Flow 2016.vi"("Descriptions"=w1062, "Array in"=w1065, "Flow Slope"=w1063, "Offset"=w1066) -> ("Sensor Cluster"=w1060:T11, "Flow (ml/min)"=w1061:dbl, "Array out"=w1059:refnum<k24>[])  [unwired: 4 in]
                n485 = local write "Sensor Voltage Cluster"(w1060) -> ()
                n486 = Bundle By Name(cluster=w1068, "Flow"=w1061) -> (w1067:T19)
                n487 = local write "Input Depths \nand Parameters Cluster"(w1067) -> ()
              }
            }
            n488 = flat-sequence {
              tunnel: w976 -> [w1039]
              tunnel: w975 -> [w1009]
              tunnel: w974 -> [w1038]
              tunnel: w973 -> [w996]
              tunnel: [w1037] -> w972
              tunnel: w971 -> [w1036]
              tunnel: w969 -> [w1030]
              tunnel: [w1029] -> _
              tunnel: [w1002] -> w968
              tunnel: w963 -> [w1025]
              tunnel: w962 -> [w1018]
              tunnel: [w1001] -> w960
              tunnel: w959 -> [w1007]
              tunnel: w957 -> [w998]
              tunnel: [w997] -> w958
              frame #0 {
                n489 = Unbundle By Name(w996) -> ("Current Relative Depth"=w1019:dbl)
                n490 = local read "Sensor Voltage Cluster"() -> (w990:T11)
                n491 = Unbundle By Name(w996) -> ("Current Absolute Depth"=w995:dbl)
                n492 = local read "Input Depths \nand Parameters Cluster"() -> (w1021:T19)
                n493 = Unbundle By Name(w1021) -> ("Start Depth"=w1020:sgl)
                n494 = global read "Kpro Globals.vi" "increment_amount"() -> (w1023:dbl)
                n495 = local read "Sensor  Real \nMeasurements"() -> (w989:T8)
                n496 = local read "Culmulative Graph Cluster"() -> (w1028:T24)
                n497 = local read "Input Depths \nand Parameters Cluster"() -> (w1033:T19)
                n498 = Equal?(x=w995, y=w1020) -> (x = y?=w1015:bool)
                n499 = And(x=w1015, y=FALSE) -> (x .and. y?=w1016:bool)
                n500 = First Call?() -> ()  [unwired: 1 out]
                n501 = Unbundle By Name(w990) -> ("Downhole Pressure"=w988:dbl)
                n502 = local read "Input Variables and Slopes"() -> (w1035:T2)
                n503 = local read "KPRO Finish\nIndicator"() -> (w1022:bool)
                n504 = local read "Depth mode"() -> (w1006:bool)
                n505 = Unbundle By Name(w989) -> ("Downhole Pressure"=w987:dbl)
                n506 = case shown="True" w1016 {
                  tunnel: w1019 -> [w1046 w1047]
                  tunnel: [w1045 w1047] -> w1024
                  tunnel: w1023 -> [w1044 _]
                  frame False {
                    n507 = Add(x=w1044, y=w1046) -> (x+y=w1045:dbl)
                  }
                  frame True {
                  }
                }
                n508 = local write "Corrected\n Pressure (ft)"(w987) -> ()
                n509 = Unbundle By Name(w1033) -> ()  [unwired: 2 out]
                n510 = Unbundle By Name(w1035) -> ("String Pot Slope"=w1034:dbl)
                n511 = call "Kpro Read String Pot 2016.vi"("Read String Pot"=w1006, "Feet of\nStainless to be\nUsed (Count) in"=w998, "Session Array in"=w1007, "Flow"=w1036, "Manual Depth In"=w1024, "Finished In"=w1022, "Depth Cluster in"=w996, "error in (no error)"=w1025, "String Pot \nSlope in"=w1034, "Sensor Cluster In in"=w1038, "Descriptions"=w1039, "Pressure in"=w987, "Array in"=w1030, "Downhole Pressure Sensor"=w1018, "Initial Measurement Input"=FALSE, "Downhole Pressure (V)"=w988) -> ("Sensor Cluster 2"=w1031:T11, "IK"=w1008:dbl, "Array out"=w1029:refnum<k24>[], "Generate Array Calc IK"=w993:bool, "Depth Rate"=→"Depth Rate\nft/min":dbl, "Feet of\nStainless to be\nUsed (Count) out"=w997:i32, "Depth Cluster out"=w1037:T21, "Single String Pot Session Array out"=w1001:dbl[][])  [unwired: 3 in, 1 out]
                "Ik" <- w1008
                n512 = And(x=w1006, y=w993) -> ()  [unwired: 1 out]
                n513 = local write "Sensor Voltage Cluster"(w1031) -> ()
                n514 = Unbundle By Name(w1037) -> ("Current Absolute Depth"=w1011:dbl)
                n515 = Bundle By Name(cluster=w1033, "Feet of Stainless"=w997) -> (w1032:T19)
                n516 = local write "Ik"(w1008) -> ()
                n517 = local write "Input Depths \nand Parameters Cluster"(w1032) -> ()
                n518 = flat-sequence {
                  tunnel: w1011 -> [w1052]
                  frame #0 {
                    n519 = local read "Corrected Pressure Cluster"() -> (w1055:T1)
                    n520 = global write "Kpro Globals.vi" "Current Depth"(w1052) -> ()
                    n521 = local write "Current Depth"(w1052) -> ()
                    n522 = Divide(x=w1052, y=3.281) -> (x/y=w1053:dbl)
                    n523 = local read "Sample Sheet Data Row Cluster 2"() -> (w1057:T3)
                    n524 = local write "Current \nDepth (m)"(w1053) -> ()
                    n525 = Unbundle By Name(w1055) -> ("Up hole Corrected Pressure"=w1054:dbl)
                    n526 = Bundle By Name(cluster=w1057, "Depth"=w1052, "Head\nPressure"=w1054) -> (w1056:T3)
                    n527 = local write "Sample Sheet Data Row Cluster 2"(w1056) -> ()
                  }
                }
                n528 = case shown="True" FALSE {
                  tunnel: w1001 -> [_ w1049]
                  tunnel: [w1048 w1050] -> w1002
                  tunnel: w1009 -> [w1048 w1051]
                  frame False {
                  }
                  frame True {
                    n529 = Build Array (concatenate)(w1051, w1049) -> (w1050:dbl[][])
                  }
                }
                n530 = call "Array to Plot 2016.vi"("Input Cumulative Array"=w1002, "Input Real Time Array"=w1001) -> ("Cumulative - Depth vs.Drive Rate"=w999:cluster{dbl[], dbl[]}, "Cumulative - Depth vs. Ik"=w1026:cluster{dbl[], dbl[]}, "Real Time - Depth vs. Drive Rate"=w1000:cluster{dbl[], dbl[]}, "Real Time - Depth vs. Ik"=w1013:cluster{dbl[], dbl[]}, "Depth Rate"=w1010:dbl)  [unwired: 2 in, 1 out]
                n531 = Bundle By Name(cluster=w1028, "Cumulative - Depth vs. Ik"=w1026, "Real Time - Depth vs. lk"=w1013, "Cumulative - Depth vs. Drive Rate"=w999, "Real Time - Depth vs. Drive Rate"=w1000) -> (w1027:T24)
                n532 = local write "Culmulative Graph Cluster"(w1027) -> ()
                n533 = local write "Large Depth IK Graph Cluster"(w1013) -> ()
                n534 = local write "Depth Rate\nft/min"(w1010) -> ()
                n535 = local write "Current Session"(w1001) -> ()
                n536 = local write "Cumulative_data_from_file"(w1002) -> ()
                n537 = local read "KPRO session report header"() -> (w991:T20)
                n538 = control-ref of="KPRO SessionOutput File Path"() -> (w1003:refnum<vi>)
                n539 = call "write KPRO file.vi"("KPRO session report header"=w991, "Corrected Array in"=w1001, "Generate Array Calc IK"=w993, "Path in"=w1003) -> ("paths ok"=w1014:bool, "appended path"=w1017:path)  [unwired: 6 in]
                n540 = case shown="True" FALSE {
                  tunnel: w1002 -> [_ w1042]
                  tunnel: w993 -> [_ w1040]
                  frame False {
                  }
                  frame True {
                    n541 = control-ref of="KPRO Cumulative Output File Path"() -> (w1041:refnum<vi>)
                    n542 = call "write KPRO file.vi"("Corrected Array in"=w1042, "Generate Array Calc IK"=w1040, "Path in"=w1041) -> ()  [unwired: 7 in, 2 out]
                  }
                }
                n543 = case shown="True" w1014 {
                  tunnel: w1017 -> [_ w1043]
                  frame False {
                  }
                  frame True {
                    n544 = local write "KPRO SessionOutput File Path"(w1043) -> ()
                  }
                }
              }
            }
          }
          frame "Sonde Sample Not Collected" {
            n545 = local write "Tab Control"(T5."Recording Reason Sonde" ("Tab Control")) -> ()
          }
          frame "Record Sonde Reason" {
            n546 = flat-sequence {
              tunnel: w1139 -> [w1157]
              tunnel: [w1156] -> w1138
              frame #0 {
                n547 = local write "Tab Control"(6) -> ()
              }
              frame #1 {
                n548 = local read "Sample Sheet Data Row Cluster 2"() -> (w1174:T3)
                n549 = property on="Select Reasons to Record Data" class="Ring (strict)"() -> ("Strings []"=w1166:string[])  [unwired: 2 in, 2 out]
                n550 = Get Date/Time In Seconds() -> (seconds since 1Jan1904=w1173:timestamp)
                n551 = Unbundle By Name(w1174) -> ("Head\nPressure"=w1172:dbl, "Depth"=w1171:dbl)
                n552 = local read "Recording Reason Sonde array"() -> (w1161:string[][])
                n553 = local read "Sonde Recording Error file"() -> (w1158:path)
                n554 = Index Array(array=w1166, index="Select Reasons to Record Data") -> (element=w1164:string)
                n555 = Format Date/Time String(seconds (now)=w1173) -> (date/time string=w1170:string)  [unwired: 2 in]
                n556 = Format Into String(w1172) -> (resulting string=w1169:string)  [unwired: 3 in, 1 out]
                n557 = Format Into String(w1171) -> (resulting string=w1168:string)  [unwired: 3 in, 1 out]
                n558 = Format Into String("Select Reasons to Record Data") -> (resulting string=w1167:string)  [unwired: 3 in, 1 out]
                n559 = Build Array(w1170, w1169, w1168, w1167, w1164) -> (w1159:string[])
                n560 = Build Array (concatenate)(w1161, w1159) -> (→"Recording Reason Sonde array":string[][])
                n561 = call-poly <vilib>:"Write Delimited Spreadsheet.vi"("file path (dialog if empty)"=w1158, "1D data"=w1159, "append to file? (new file:F)"=TRUE, "error in (no error)"=w1157, "delimiter (\\t)"="," ("delimiter (\\t)")) -> ("error out"=w1156:errorcluster)  [unwired: 9 in, 1 out]
              }
            }
          }
          frame "Record IK Reason" {
            n562 = flat-sequence {
              frame #0 {
                w1191 = "%3.4f" ("format string")
                n563 = local read "Input Depths \nand Parameters Cluster"() -> (w1200:T19)
                n564 = local read "Down hole Pressure (ft)"() -> (w1192:dbl)
                n565 = Unbundle By Name(w1200) -> ("Flow"=w1199:dbl, "Zeroed \nPressure"=w1197:dbl, "Feet of Stainless"=w1194:i32)
                n566 = local read "Select Entry \nfor IK Log"() -> (w1206:u16)
                n567 = property on="Select Entry \nfor IK Log" class="Ring (strict)"() -> ("Strings []"=w1205:string[])  [unwired: 2 in, 2 out]
                n568 = local read "Sample Sheet Data Row Cluster 2"() -> (w1218:T3)
                n569 = local write "Tab Control"(T5."Pressure/Flow/IK Graphs" ("Tab Control")) -> ()
                n570 = Get Date/Time In Seconds() -> (seconds since 1Jan1904=w1217:timestamp)
                n571 = Unbundle By Name(w1218) -> ("Head\nPressure"=w1216:dbl, "Depth"=w1215:dbl)
                n572 = Format Into String(format string=w1191, w1199) -> (resulting string=w1198:string)  [unwired: 2 in, 1 out]
                n573 = Format Into String(format string=w1191, w1197) -> (resulting string=w1196:string)  [unwired: 2 in, 1 out]
                n574 = Index Array(array=w1205, index=w1206) -> (element=w1209:string)
                n575 = Format Into String(w1194) -> (resulting string=w1195:string)  [unwired: 3 in, 1 out]
                n576 = Format Date/Time String(seconds (now)=w1217) -> (date/time string=w1213:string)  [unwired: 2 in]
                n577 = Format Into String(format string=w1191, w1192) -> (resulting string=w1193:string)  [unwired: 2 in, 1 out]
                n578 = Format Into String(format string=w1191, w1216) -> (resulting string=w1212:string)  [unwired: 2 in, 1 out]
                n579 = Format Into String(format string=w1191, w1215) -> (resulting string=w1211:string)  [unwired: 2 in, 1 out]
                n580 = Format Into String(w1206) -> (resulting string=w1210:string)  [unwired: 3 in, 1 out]
                n581 = Build Array(w1213, w1212, w1211, w1210, w1209, w1198, w1196, w1195, w1193) -> (w1208:string[])
                n582 = local read "IK Reason array"() -> (w1202:string[][])
                n583 = Build Array (concatenate)(w1202, w1208) -> (→"IK Reason array":string[][])
                n584 = call-poly <vilib>:"Write Delimited Spreadsheet.vi"("file path (dialog if empty)"="Sonde IK Recording Failure Path", "1D data"=w1208, "append to file? (new file:F)"=TRUE, "delimiter (\\t)"="," ("delimiter (\\t)")) -> ()  [unwired: 10 in, 2 out]
              }
            }
          }
          frame "Continuous  Sonde Data" {
            n585 = local read "Found Quanta Sonde Com Port"() -> (w1241:refnum<visa-resource-name>)
            n586 = control-ref of="Sonde Data Display"() -> (w1244:refnum<vi>)
            n587 = local read "Sample Sheet Data Row Cluster 2"() -> (w1222:T3)
            n588 = Unbundle By Name(w1222) -> ("Sonde Data Cluster.Cumulative\nVolume (ml)"=w1221:dbl)
            n589 = call "SDI-12 Continuous Operations.vi"("RS232 Port In"=w1241, "Sensor Address In"="0", "Sonde Data Ctl Refnum"=w1244, "Error In (No Error)"=w1243) -> ("output cluster"=w1220:T4, "Temperature"=w1239:cluster{"Y":dbl[], "Y":dbl[]}[], "Sonde Data Display"=w1238:T16, "Error Out"=w1242:errorcluster)  [unwired: 8 in, 4 out]
            n590 = Bundle By Name(cluster=w1220, "Cumulative\nVolume (ml)"=w1221) -> (w1219:T4)
            n591 = Bundle By Name(cluster=w1222, "Sonde Data Cluster"=w1219) -> (w1240:T3)
            n592 = local write "Temperature"(w1239) -> ()
            n593 = local write "Sonde Data Display"(w1238) -> ()
            n594 = local write "Sample Sheet Data Row Cluster 2"(w1240) -> ()
          }
          frame "Acq. Single Sonde Point" {
            n595 = invoke on="Record Single Sample" class="Bool" method="Reinit To Default"(error in=w1274) -> (error out=w1273:errorcluster)  [unwired: 2 in, 2 out]
            n596 = call <vilib>:"Clear Errors.vi"("error in (no error)"=w1273) -> ("error out"=w1265:errorcluster)  [unwired: 5 in, 1 out]
            n597 = case shown="False" FALSE {
              tunnel: w1281 -> [w1284 w1292]
              tunnel: [w1283 w1288] -> w1280
              tunnel: [w1284 w1287] -> w1277
              tunnel: [w1282 w1286] -> w1276
              tunnel: w1265 -> [w1283 w1285]
              tunnel: w1250 -> [w1282 _]
              frame False {
              }
              frame True {
                n598 = call "get sample sheet data cells.vi"("error in (no error)"=w1285, "NI_report in"=w1292) -> ("error out"=w1289:errorcluster, "data"=w1291:string[][], "NI_report out"=w1287:refnum<class "NI_report.lvclass">, "left edge output cluster"=w1290:cluster{"row":i32, "column":i32})  [unwired: 5 in, 1 out]
                n599 = flat-sequence {
                  tunnel: w1289 -> [w1304]
                  tunnel: [w1297] -> _
                  tunnel: w1290 -> [w1302]
                  tunnel: [w1301] -> w1288
                  tunnel: [w1300] -> _
                  tunnel: [w1299] -> w1286
                  tunnel: w1291 -> [w1297]
                  frame #0 {
                    n600 = Array Subset(array=w1297, index (col)=2 ("index")) -> (w1293:string[][])  [unwired: 3 in]
                    n601 = local write "subarray"(w1293) -> ()
                    n602 = local read "Current Sample Sheet"() -> (w1296:string)
                    n603 = call "find last occupied cell.vi"("data"=w1297, "Active Sheet"=w1296, "Header Rows to remove"=3, "sub array start"=w1302, "error in (no error)"=w1304) -> ("row max value"=w1300:i32, "column max value"=w1295:i32, 13:"start of last occupied row"=w1299:cluster{"row":i32, "column":i32}, 14:"start of last occupied row"=w1294:string, "error out"=w1301:errorcluster)  [unwired: 4 in, 2 out]
                    n604 = local write "last occupied cell's name"(w1294) -> ()
                    n605 = local write "row max value"(w1295) -> ()
                  }
                }
              }
            }
            n606 = flat-sequence {
              tunnel: w1280 -> [w1370]
              tunnel: [w1369] -> w1253
              tunnel: w1269 -> [w1368]
              tunnel: [w1367] -> w1268
              tunnel: [w1359] -> w1261
              tunnel: [w1356] -> _
              tunnel: w1257 -> [w1366]
              tunnel: [w1355] -> _
              frame #0 {
                n607 = local read "Corrected\n Pressure (ft)"() -> (w1353:dbl)
                n608 = local read "Current Depth"() -> (w1352:sgl)
                n609 = local read "Depth Cluster"() -> (w1351:T21)
                n610 = Unbundle By Name(w1351) -> ("Total Volume Out"=w1350:dbl)
                n611 = local read "Sample Sheet Data Row Cluster 2"() -> (w1358:T3)
                n612 = control-ref of="Found Quanta Sonde Com Port"() -> (w1365:refnum<vi>)
                n613 = control-ref of="Current Time (s)"() -> (w1361:refnum<vi>)
                n614 = Bundle By Name(cluster=w1358, "Head\nPressure"=w1353, "Depth"=w1352, "Sonde Data Cluster.Cumulative\nVolume (ml)"=w1350) -> (w1354:T3)
                n615 = control-ref of="Sonde Data Display"() -> (w1364:refnum<vi>)
                n616 = control-ref of="Sonde Data Display"() -> (w1363:refnum<vi>)
                n617 = local write "Tab Control"(T5."Sonde Data" ("Tab Control")) -> ()
                n618 = control-ref of="Temperature"() -> (w1362:refnum<vi>)
                n619 = call "Sonde Single Measurement Subvi.vi"("VISAResourceName in"=w1365, "Time Array"=w1368, "Previous time"=w1366, "Sonde Data Display"=w1364, "Sonde Graph in"=w1363, "Temp Graph 3"=w1362, "error in (no error)"=w1370, "Row Cluster Input"=w1354, "reference 5"=w1361) -> ("seconds since 1Jan1904"=w1356:timestamp, "Sample Sheet Data Row Cluster 2"=w1359:T3, "output cluster"=→"output cluster":T4, "time array out"=w1367:dbl[], "error out"=w1369:errorcluster)  [unwired: 1 in, 1 out]
                n620 = local write "Sample Sheet Data Row Cluster 2"(w1359) -> ()
                n621 = To Double Precision Float(number=w1356) -> (double precision float=w1355:dbl)
              }
            }
            n622 = flat-sequence {
              tunnel: w1261 -> [w1349]
              tunnel: w1260 -> [w1346]
              tunnel: w1248 -> [w1337]
              tunnel: [w1343] -> w1255
              tunnel: w1253 -> [w1342]
              tunnel: [w1341] -> w1252
              tunnel: [w1340] -> w1247
              frame #0 {
                n623 = Increment(x=w1337) -> (x+1=w1340:i32)
                n624 = local read "Sonde Data Array"() -> (w1345:T13)
                n625 = call "populate sonde row cluster from sonde data cluster.vi"("Initialize \nInitial Value \nCluster"=TRUE ("Initialize \nInitial Value \nCluster"), "error in (no error)"=w1342, "Sonde Parameters \nInitial Values"=w1346, "Sample Sheet Data Row Cluster"=w1349, "Sonde Parameters \nTolerance Limits"="Sonde Parameters \nTolerance Limits") -> ("error out"=w1341:errorcluster, "Cluster"=w1338:T30, "Sonde Parameters \nInitial Values Out"=w1343:T7)  [unwired: 4 in]
                n626 = local write "Sonde Parameters \nInitial Values"(w1343) -> ()
                n627 = Array Subset(array=w1345, length=w1337) -> (w1339:T13)  [unwired: 1 in]
                n628 = local write "Sonde Array Size"(w1337) -> ()
                n629 = Build Array (concatenate)(w1339, w1338) -> (w1344:T30[])
                n630 = local write "Sonde Data Array"(w1344) -> ()
              }
            }
            n631 = case shown="False" FALSE {
              tunnel: w1279 -> [_ w1321]
              tunnel: w1278 -> [_ w1320]
              tunnel: w1277 -> [w1307 w1319]
              tunnel: w1276 -> [w1308 w1318]
              tunnel: [w1307 w1316] -> w1275
              tunnel: [w1306 w1315] -> w1272
              tunnel: [w1308 w1314] -> w1271
              tunnel: [w1305 w1313] -> w1270
              tunnel: w1261 -> [_ w1312]
              tunnel: w1247 -> [w1305 w1311]
              tunnel: w1252 -> [w1306 w1310]
              frame False {
              }
              frame True {
                n632 = call "write out sonde row.vi"("NI_report in"=w1319, "Columns"=w1321, "Column of Volume"=w1320, "Sample Sheet Data Row Cluster"=w1312, "row index"=w1311, "error in (no error)"=w1310, "start of last occupied row"=w1318) -> ("NI_report out"=w1317:refnum<class "NI_report.lvclass">, "row index out"=w1313:i32, "error out"=w1309:errorcluster)  [unwired: 6 in]
                n633 = flat-sequence {
                  tunnel: w1309 -> [w1336]
                  tunnel: w1317 -> [w1335]
                  tunnel: [w1334] -> w1316
                  tunnel: [w1329] -> w1315
                  tunnel: [w1327] -> w1314
                  frame #0 {
                    n634 = local read "Current Sample Sheet"() -> (w1325:string)
                    n635 = call <vilib>:"Clear Errors.vi"("error in (no error)"=w1336) -> ("error out"=w1323:errorcluster)  [unwired: 5 in, 1 out]
                    n636 = call "get sample sheet data cells.vi"("error in (no error)"=w1323, "NI_report in"=w1335) -> ("error out"=w1330:errorcluster, "data"=w1331:string[][], "NI_report out"=w1334:refnum<class "NI_report.lvclass">, "left edge output cluster"=w1328:cluster{"row":i32, "column":i32})  [unwired: 5 in, 1 out]
                    n637 = call "find last occupied cell.vi"("data"=w1331, "Active Sheet"=w1325, "Header Rows to remove"=3, "sub array start"=w1328, "error in (no error)"=w1330) -> ("row max value"=w1326:i32, 13:"start of last occupied row"=w1327:cluster{"row":i32, "column":i32}, 14:"start of last occupied row"=w1324:string, "error out"=w1329:errorcluster)  [unwired: 4 in, 3 out]
                    n638 = Array Subset(array=w1331, index (col)=2 ("index")) -> (w1322:string[][])  [unwired: 3 in]
                    n639 = local write "row max value"(w1326) -> ()
                    n640 = local write "last occupied cell's name"(w1324) -> ()
                    n641 = local write "subarray"(w1322) -> ()
                  }
                }
              }
            }
          }
          frame "pH Calibration Zero" {
            n642 = invoke on="Record Single Sample" class="Bool" method="Reinit To Default"(error in=w1394) -> (error out=w1393:errorcluster)  [unwired: 2 in, 2 out]
            n643 = call <vilib>:"Clear Errors.vi"("error in (no error)"=w1393) -> ("error out"=w1381:errorcluster)  [unwired: 5 in, 1 out]
            n644 = case shown="True" FALSE {
              tunnel: w1409 -> [w1412 w1420]
              tunnel: [w1411 w1416] -> w1408
              tunnel: [w1412 w1415] -> w1404
              tunnel: [w1410 w1414] -> w1402
              tunnel: w1381 -> [w1411 w1413]
              tunnel: w1371 -> [w1410 _]
              frame False {
              }
              frame True {
                n645 = call "get sample sheet data cells.vi"("error in (no error)"=w1413, "NI_report in"=w1420) -> ("error out"=w1417:errorcluster, "data"=w1419:string[][], "NI_report out"=w1415:refnum<class "NI_report.lvclass">, "left edge output cluster"=w1418:cluster{"row":i32, "column":i32})  [unwired: 5 in, 1 out]
                n646 = flat-sequence {
                  tunnel: w1417 -> [w1430]
                  tunnel: [w1424] -> _
                  tunnel: w1418 -> [w1428]
                  tunnel: [w1427] -> w1416
                  tunnel: [w1426] -> _
                  tunnel: [w1425] -> w1414
                  tunnel: w1419 -> [w1424]
                  frame #0 {
                    n647 = local read "Current Sample Sheet"() -> (w1423:string)
                    n648 = call "find last occupied cell.vi"("data"=w1424, "Active Sheet"=w1423, "Header Rows to remove"=3, "sub array start"=w1428, "error in (no error)"=w1430) -> ("row max value"=w1426:i32, "column max value"=w1422:i32, 13:"start of last occupied row"=w1425:cluster{"row":i32, "column":i32}, 14:"start of last occupied row"=w1421:string, "error out"=w1427:errorcluster)  [unwired: 4 in, 2 out]
                    n649 = local write "row max value"(w1422) -> ()
                    n650 = local write "last occupied cell's name"(w1421) -> ()
                  }
                }
              }
            }
            n651 = local read "Found Quanta Sonde Com Port"() -> (w1398:refnum<visa-resource-name>)
            n652 = Equal?(x=w1398, y=refnum<visa-resource-name> refnum ("RS232 Port Out")) -> (x = y?=w1400:bool)
            n653 = case shown="False" w1400 {
              tunnel: w1398 -> [w1461 _]
              tunnel: [w1469 w1503] -> w1401
              tunnel: w1408 -> [w1454 w1506]
              tunnel: [w1472 w1506] -> w1405
              tunnel: w1388 -> [w1460 w1505]
              tunnel: [w1468 w1493] -> w1387
              tunnel: [w1467 w1492] -> w1386
              tunnel: w1385 -> [w1458 w1504]
              tunnel: w1384 -> [_ w1489]
              frame False {
                w1466 = "0" ("Sensor Address In")
                n654 = flat-sequence {
                  tunnel: w1461 -> [w1486]
                  tunnel: [w1485] -> _
                  tunnel: w1454 -> [w1483]
                  tunnel: [w1482] -> w1453
                  tunnel: w1458 -> [w1481]
                  tunnel: [w1480] -> w1457
                  tunnel: w1460 -> [w1479]
                  tunnel: [w1478] -> w1459
                  tunnel: [w1477] -> w1456
                  tunnel: [w1476] -> w1455
                  frame #0 {
                    w1476 = TRUE ("Save File")
                    n655 = local read "Sonde Calibration History File"() -> (w1477:path)
                    n656 = control-ref of="Sonde Data Display"() -> (w1485:refnum<vi>)
                    n657 = call "SDI-12 Single Operation with output cluster.vi"("RS232 Port In"=w1486, "Sensor Address In"="0", "Sonde Data Ctl Refnum"=w1485, "Error In (No Error)"=w1483, "file directory (dialog if empty)"=w1477, "Save File"=w1476, "Time Array In"=w1479, "Measurement Array In"=w1481) -> ("time array out"=w1478:dbl[], "Measurement  array Out"=w1480:dbl[][], "Error Out"=w1482:errorcluster)  [unwired: 10 in, 7 out]
                  }
                }
                n658 = control-ref of="Sonde Data Display"() -> (w1473:refnum<vi>)
                n659 = local read "Sample Sheet Data Row Cluster 2"() -> (w1470:T3)
                n660 = call "Calibrate pH Sensor.vi"("Calibration Standard"="pH Zero", "Error In (No Error)"=w1453, "Sensor Address In"=w1466, "RS232 Port In"=w1461) -> ("Error Out"=w1465:errorcluster, "RS232 Port Out"=w1464:refnum<visa-resource-name>, "Calibration Response"=→"pH Zero Calibration Response":T18)  [unwired: 2 in, 3 out]
                n661 = call "SDI-12 Single Operation with output cluster.vi"("RS232 Port In"=w1464, "Sensor Address In"=w1466, "Sonde Data Ctl Refnum"=w1473, "Error In (No Error)"=w1465, "file directory (dialog if empty)"=w1456, "Save File"=w1455, "Time Array In"=w1459, "Measurement Array In"=w1457) -> ("time array out"=w1468:dbl[], "Measurement  array Out"=w1467:dbl[][], "output cluster"=w1471:T4, "Temperature"=w1475:cluster{"Y":dbl[], "Y":dbl[]}[], "Sonde Data Display"=w1474:T16, "Error Out"=w1472:errorcluster)  [unwired: 10 in, 4 out]
                n662 = local write "Temperature"(w1475) -> ()
                n663 = local write "Sonde Data Display"(w1474) -> ()
                n664 = Bundle By Name(cluster=w1470, "Sonde Data Cluster"=w1471) -> (w1469:T3)
              }
              frame True {
                n665 = Get Date/Time In Seconds() -> (seconds since 1Jan1904=w1495:timestamp)
                n666 = To Double Precision Float(number=w1495) -> (double precision float=w1494:dbl)
                n667 = local read "Sample Sheet Data Row Cluster 2"() -> (w1503:T3)
                n668 = Subtract(x=w1494, y=w1489) -> (x-y=w1487:dbl)
                n669 = local write "Current Time (s)"(w1487) -> ()
                n670 = Unbundle By Name(w1503) -> ("Sonde Data Cluster.Temp deg C"=w1488:dbl, "Sonde Data Cluster.pH"=w1502:dbl, "Sonde Data Cluster.Specific\nCond (mS)"=w1501:dbl, "Sonde Data Cluster.Salinity"=w1500:dbl, "Sonde Data Cluster.Dissolved\nOxygen mg/L"=w1499:dbl, "Sonde Data Cluster.ORP"=w1498:dbl)  [unwired: 1 out]
                n671 = Build Array(w1488, w1502, w1501, w1500, w1499, 0.0 ("element"), w1498) -> (w1496:dbl[])
                n672 = Build Array (concatenate)(w1504, w1496) -> (w1492:dbl[][])
                n673 = Build Array (concatenate)(w1505, w1487) -> (w1493:dbl[])
                n674 = call "format into Sonde Vertical Graph Data Input.vi"("Sonde Measurement Array"=w1492, "Time Array"=w1493) -> ("Sonde Data Display"=w1491:T16, "Temperature"=w1490:cluster{"X":dbl[], "Y":dbl[]}[])  [unwired: 8 in]
                n675 = local write "Temperature"(w1490) -> ()
                n676 = local write "Sonde Data Display"(w1491) -> ()
              }
            }
            n677 = local write "Sample Sheet Data Row Cluster 2"(w1401) -> ()
            n678 = call "write out sonde row.vi"("NI_report in"=w1404, "Columns"=w1407, "Column of Volume"=w1406, "Sample Sheet Data Row Cluster"=w1401, "row index"=w1390, "error in (no error)"=w1405, "start of last occupied row"=w1402) -> ("NI_report out"=w1396:refnum<class "NI_report.lvclass">, "row index out"=w1389:i32, "error out"=w1397:errorcluster)  [unwired: 6 in]
            n679 = case shown="False" FALSE {
              tunnel: w1397 -> [w1432 w1438]
              tunnel: w1396 -> [w1433 w1437]
              tunnel: [w1433 w1436] -> w1395
              tunnel: [w1432 w1435] -> w1392
              tunnel: [w1431 w1434] -> w1391
              tunnel: w1371 -> [w1431 _]
              frame False {
              }
              frame True {
                n680 = flat-sequence {
                  tunnel: w1438 -> [w1452]
                  tunnel: w1437 -> [w1451]
                  tunnel: [w1450] -> w1436
                  tunnel: [w1445] -> w1435
                  tunnel: [w1443] -> w1434
                  frame #0 {
                    n681 = call <vilib>:"Clear Errors.vi"("error in (no error)"=w1452) -> ("error out"=w1439:errorcluster)  [unwired: 5 in, 1 out]
                    n682 = local read "Current Sample Sheet"() -> (w1441:string)
                    n683 = call "get sample sheet data cells.vi"("error in (no error)"=w1439, "NI_report in"=w1451) -> ("error out"=w1446:errorcluster, "data"=w1447:string[][], "NI_report out"=w1450:refnum<class "NI_report.lvclass">, "left edge output cluster"=w1444:cluster{"row":i32, "column":i32})  [unwired: 5 in, 1 out]
                    n684 = call "find last occupied cell.vi"("data"=w1447, "Active Sheet"=w1441, "Header Rows to remove"=3, "sub array start"=w1444, "error in (no error)"=w1446) -> ("row max value"=w1442:i32, 13:"start of last occupied row"=w1443:cluster{"row":i32, "column":i32}, 14:"start of last occupied row"=w1440:string, "error out"=w1445:errorcluster)  [unwired: 4 in, 3 out]
                    n685 = Array Subset(array=w1447, index (col)=2 ("index")) -> ()  [unwired: 3 in, 1 out]
                    n686 = local write "row max value"(w1442) -> ()
                    n687 = local write "last occupied cell's name"(w1440) -> ()
                  }
                }
              }
            }
          }
          frame "pH Calibration Standard" {
            n688 = invoke on="Record Single Sample" class="Bool" method="Reinit To Default"(error in=w1532) -> (error out=w1531:errorcluster)  [unwired: 2 in, 2 out]
            n689 = call <vilib>:"Clear Errors.vi"("error in (no error)"=w1531) -> ("error out"=w1519:errorcluster)  [unwired: 5 in, 1 out]
            n690 = case shown="True" FALSE {
              tunnel: w1546 -> [w1562 w1570]
              tunnel: [w1561 w1566] -> w1545
              tunnel: [w1562 w1565] -> w1541
              tunnel: [w1560 w1564] -> w1508
              tunnel: w1519 -> [w1561 w1563]
              tunnel: w1509 -> [w1560 _]
              frame False {
              }
              frame True {
                n691 = call "get sample sheet data cells.vi"("error in (no error)"=w1563, "NI_report in"=w1570) -> ("error out"=w1567:errorcluster, "data"=w1569:string[][], "NI_report out"=w1565:refnum<class "NI_report.lvclass">, "left edge output cluster"=w1568:cluster{"row":i32, "column":i32})  [unwired: 5 in, 1 out]
                n692 = flat-sequence {
                  tunnel: w1567 -> [w1581]
                  tunnel: [w1574] -> _
                  tunnel: w1568 -> [w1579]
                  tunnel: [w1578] -> w1566
                  tunnel: [w1577] -> _
                  tunnel: [w1576] -> w1564
                  tunnel: w1569 -> [w1574]
                  frame #0 {
                    n693 = local read "Current Sample Sheet"() -> (w1573:string)
                    n694 = Array Subset(array=w1574, index (col)=2 ("index")) -> ()  [unwired: 3 in, 1 out]
                    n695 = call "find last occupied cell.vi"("data"=w1574, "Active Sheet"=w1573, "Header Rows to remove"=3, "sub array start"=w1579, "error in (no error)"=w1581) -> ("row max value"=w1577:i32, "column max value"=w1572:i32, 13:"start of last occupied row"=w1576:cluster{"row":i32, "column":i32}, 14:"start of last occupied row"=w1571:string, "error out"=w1578:errorcluster)  [unwired: 4 in, 2 out]
                    n696 = local write "last occupied cell's name"(w1571) -> ()
                    n697 = local write "row max value"(w1572) -> ()
                  }
                }
              }
            }
            n698 = local read "Found Quanta Sonde Com Port"() -> (w1536:refnum<visa-resource-name>)
            n699 = Equal?(x=w1536, y=refnum<visa-resource-name> refnum ("RS232 Port Out")) -> (x = y?=w1538:bool)
            n700 = case shown="False" w1538 {
              tunnel: w1536 -> [w1612 _]
              tunnel: [w1620 w1655] -> w1539
              tunnel: w1545 -> [w1611 w1658]
              tunnel: [w1623 w1658] -> w1542
              tunnel: w1526 -> [w1606 w1657]
              tunnel: [w1619 w1645] -> w1525
              tunnel: [w1618 w1644] -> w1524
              tunnel: w1523 -> [w1608 w1656]
              tunnel: w1522 -> [_ w1641]
              frame False {
                n701 = flat-sequence {
                  tunnel: w1612 -> [w1638]
                  tunnel: [w1637] -> _
                  tunnel: w1611 -> [w1635]
                  tunnel: [w1634] -> w1610
                  tunnel: w1608 -> [w1633]
                  tunnel: [w1632] -> w1607
                  tunnel: w1606 -> [w1631]
                  tunnel: [w1630] -> w1605
                  tunnel: [w1629] -> w1609
                  tunnel: [w1628] -> w1604
                  frame #0 {
                    w1628 = TRUE ("Save File")
                    n702 = local read "Sonde Calibration History File"() -> (w1629:path)
                    n703 = control-ref of="Sonde Data Display"() -> (w1637:refnum<vi>)
                    n704 = call "SDI-12 Single Operation with output cluster.vi"("RS232 Port In"=w1638, "Sensor Address In"="0", "Sonde Data Ctl Refnum"=w1637, "Error In (No Error)"=w1635, "file directory (dialog if empty)"=w1629, "Save File"=w1628, "Time Array In"=w1631, "Measurement Array In"=w1633) -> ("time array out"=w1630:dbl[], "Measurement  array Out"=w1632:dbl[][], "Error Out"=w1634:errorcluster)  [unwired: 10 in, 7 out]
                  }
                }
                n705 = control-ref of="Sonde Data Display"() -> (w1624:refnum<vi>)
                n706 = call "Calibrate pH Sensor.vi"("Calibration Standard"="pH Reference", "Error In (No Error)"=w1610, "Sensor Address In"="0", "RS232 Port In"=w1612) -> ("Error Out"=w1616:errorcluster, "RS232 Port Out"=w1614:refnum<visa-resource-name>, "Calibration Response"=→"pH Reference Calibration Response":T18)  [unwired: 2 in, 3 out]
                n707 = local read "Sample Sheet Data Row Cluster 2"() -> (w1621:T3)
                n708 = call "SDI-12 Single Operation with output cluster.vi"("RS232 Port In"=w1614, "Sensor Address In"="0", "Sonde Data Ctl Refnum"=w1624, "Error In (No Error)"=w1616, "file directory (dialog if empty)"=w1609, "Save File"=w1604, "Time Array In"=w1605, "Measurement Array In"=w1607) -> ("time array out"=w1619:dbl[], "Measurement  array Out"=w1618:dbl[][], "output cluster"=w1622:T4, "Temperature"=w1626:cluster{"Y":dbl[], "Y":dbl[]}[], "Sonde Data Display"=w1625:T16, "Error Out"=w1623:errorcluster)  [unwired: 10 in, 4 out]
                n709 = Bundle By Name(cluster=w1621, "Sonde Data Cluster"=w1622) -> (w1620:T3)
                n710 = local write "Temperature"(w1626) -> ()
                n711 = local write "Sonde Data Display"(w1625) -> ()
              }
              frame True {
                n712 = Get Date/Time In Seconds() -> (seconds since 1Jan1904=w1647:timestamp)
                n713 = To Double Precision Float(number=w1647) -> (double precision float=w1646:dbl)
                n714 = local read "Sample Sheet Data Row Cluster 2"() -> (w1655:T3)
                n715 = Subtract(x=w1646, y=w1641) -> (x-y=w1639:dbl)
                n716 = local write "Current Time (s)"(w1639) -> ()
                n717 = Unbundle By Name(w1655) -> ("Sonde Data Cluster.Temp deg C"=w1640:dbl, "Sonde Data Cluster.pH"=w1654:dbl, "Sonde Data Cluster.Specific\nCond (mS)"=w1653:dbl, "Sonde Data Cluster.Salinity"=w1652:dbl, "Sonde Data Cluster.Dissolved\nOxygen mg/L"=w1651:dbl, "Sonde Data Cluster.ORP"=w1650:dbl)  [unwired: 1 out]
                n718 = Build Array(w1640, w1654, w1653, w1652, w1651, 0.0 ("element"), w1650) -> (w1648:dbl[])
                n719 = Build Array (concatenate)(w1656, w1648) -> (w1644:dbl[][])
                n720 = Build Array (concatenate)(w1657, w1639) -> (w1645:dbl[])
                n721 = call "format into Sonde Vertical Graph Data Input.vi"("Sonde Measurement Array"=w1644, "Time Array"=w1645) -> ("Sonde Data Display"=w1643:T16, "Temperature"=w1642:cluster{"X":dbl[], "Y":dbl[]}[])  [unwired: 8 in]
                n722 = local write "Temperature"(w1642) -> ()
                n723 = local write "Sonde Data Display"(w1643) -> ()
              }
            }
            n724 = case shown="False" FALSE {
              tunnel: w1544 -> [_ w1559]
              tunnel: w1543 -> [_ w1558]
              tunnel: w1542 -> [w1549 w1557]
              tunnel: w1541 -> [w1548 w1556]
              tunnel: w1539 -> [_ w1555]
              tunnel: [w1549 w1554] -> w1535
              tunnel: [w1548 w1553] -> w1534
              tunnel: w1528 -> [w1547 w1552]
              tunnel: [w1547 w1551] -> w1527
              tunnel: w1508 -> [_ w1550]
              frame False {
              }
              frame True {
                n725 = call "write out sonde row.vi"("NI_report in"=w1556, "Columns"=w1559, "Column of Volume"=w1558, "Sample Sheet Data Row Cluster"=w1555, "row index"=w1552, "error in (no error)"=w1557, "start of last occupied row"=w1550) -> ("NI_report out"=w1553:refnum<class "NI_report.lvclass">, "row index out"=w1551:i32, "error out"=w1554:errorcluster)  [unwired: 6 in]
              }
            }
            n726 = local write "Sample Sheet Data Row Cluster 2"(w1539) -> ()
            n727 = case shown="False" FALSE {
              tunnel: w1535 -> [w1583 w1589]
              tunnel: w1534 -> [w1584 w1588]
              tunnel: [w1584 w1587] -> w1533
              tunnel: [w1583 w1586] -> w1530
              tunnel: [w1582 w1585] -> w1529
              tunnel: w1508 -> [w1582 _]
              frame False {
              }
              frame True {
                n728 = flat-sequence {
                  tunnel: w1589 -> [w1603]
                  tunnel: w1588 -> [w1602]
                  tunnel: [w1601] -> w1587
                  tunnel: [w1596] -> w1586
                  tunnel: [w1594] -> w1585
                  frame #0 {
                    n729 = call <vilib>:"Clear Errors.vi"("error in (no error)"=w1603) -> ("error out"=w1590:errorcluster)  [unwired: 5 in, 1 out]
                    n730 = local read "Current Sample Sheet"() -> (w1592:string)
                    n731 = call "get sample sheet data cells.vi"("error in (no error)"=w1590, "NI_report in"=w1602) -> ("error out"=w1597:errorcluster, "data"=w1598:string[][], "NI_report out"=w1601:refnum<class "NI_report.lvclass">, "left edge output cluster"=w1595:cluster{"row":i32, "column":i32})  [unwired: 5 in, 1 out]
                    n732 = call "find last occupied cell.vi"("data"=w1598, "Active Sheet"=w1592, "Header Rows to remove"=3, "sub array start"=w1595, "error in (no error)"=w1597) -> ("row max value"=w1593:i32, 13:"start of last occupied row"=w1594:cluster{"row":i32, "column":i32}, 14:"start of last occupied row"=w1591:string, "error out"=w1596:errorcluster)  [unwired: 4 in, 3 out]
                    n733 = Array Subset(array=w1598, index (col)=2 ("index")) -> ()  [unwired: 3 in, 1 out]
                    n734 = local write "row max value"(w1593) -> ()
                    n735 = local write "last occupied cell's name"(w1591) -> ()
                  }
                }
              }
            }
          }
          frame "ORP Calibration Standard" {
            n736 = invoke on="Record Single Sample" class="Bool" method="Reinit To Default"(error in=w1685) -> (error out=w1684:errorcluster)  [unwired: 2 in, 2 out]
            n737 = call <vilib>:"Clear Errors.vi"("error in (no error)"=w1684) -> ("error out"=w1674:errorcluster)  [unwired: 5 in, 1 out]
            n738 = case shown="True" FALSE {
              tunnel: w1698 -> [w1700 w1709]
              tunnel: [w1701 w1705] -> w1697
              tunnel: [w1700 w1704] -> w1693
              tunnel: w1674 -> [w1701 w1703]
              tunnel: [w1699 w1702] -> w1663
              tunnel: w1660 -> [w1699 _]
              frame False {
              }
              frame True {
                n739 = call "get sample sheet data cells.vi"("error in (no error)"=w1703, "NI_report in"=w1709) -> ("error out"=w1706:errorcluster, "data"=w1708:string[][], "NI_report out"=w1704:refnum<class "NI_report.lvclass">, "left edge output cluster"=w1707:cluster{"row":i32, "column":i32})  [unwired: 5 in, 1 out]
                n740 = flat-sequence {
                  tunnel: w1706 -> [w1720]
                  tunnel: [w1713] -> _
                  tunnel: w1707 -> [w1718]
                  tunnel: [w1717] -> w1705
                  tunnel: [w1716] -> _
                  tunnel: [w1715] -> w1702
                  tunnel: w1708 -> [w1713]
                  frame #0 {
                    n741 = local read "Current Sample Sheet"() -> (w1712:string)
                    n742 = Array Subset(array=w1713, index (col)=2 ("index")) -> ()  [unwired: 3 in, 1 out]
                    n743 = call "find last occupied cell.vi"("data"=w1713, "Active Sheet"=w1712, "Header Rows to remove"=3, "sub array start"=w1718, "error in (no error)"=w1720) -> ("row max value"=w1716:i32, "column max value"=w1711:i32, 13:"start of last occupied row"=w1715:cluster{"row":i32, "column":i32}, 14:"start of last occupied row"=w1710:string, "error out"=w1717:errorcluster)  [unwired: 4 in, 2 out]
                    n744 = local write "last occupied cell's name"(w1710) -> ()
                    n745 = local write "row max value"(w1711) -> ()
                  }
                }
              }
            }
            n746 = local read "Found Quanta Sonde Com Port"() -> (w1689:refnum<visa-resource-name>)
            n747 = Equal?(x=w1689, y=refnum<visa-resource-name> refnum ("RS232 Port Out")) -> (x = y?=w1690:bool)
            n748 = case shown="False" w1690 {
              tunnel: w1689 -> [w1760 _]
              tunnel: [w1771 w1806] -> w1691
              tunnel: w1697 -> [w1763 w1809]
              tunnel: [w1774 w1809] -> w1694
              tunnel: w1679 -> [w1761 w1808]
              tunnel: [w1770 w1796] -> w1678
              tunnel: [w1769 w1795] -> w1667
              tunnel: w1666 -> [w1759 w1807]
              tunnel: w1677 -> [_ w1792]
              frame False {
                n749 = flat-sequence {
                  tunnel: w1760 -> [w1789]
                  tunnel: [w1788] -> _
                  tunnel: w1763 -> [w1786]
                  tunnel: [w1785] -> w1762
                  tunnel: w1759 -> [w1784]
                  tunnel: [w1783] -> w1758
                  tunnel: w1761 -> [w1782]
                  tunnel: [w1781] -> _
                  tunnel: [w1780] -> w1757
                  tunnel: [w1779] -> w1756
                  frame #0 {
                    w1779 = TRUE ("Save File")
                    n750 = local read "Sonde Calibration History File"() -> (w1780:path)
                    n751 = control-ref of="Sonde Data Display"() -> (w1788:refnum<vi>)
                    n752 = call "SDI-12 Single Operation with output cluster.vi"("RS232 Port In"=w1789, "Sensor Address In"="0", "Sonde Data Ctl Refnum"=w1788, "Error In (No Error)"=w1786, "file directory (dialog if empty)"=w1780, "Save File"=w1779, "Time Array In"=w1782, "Measurement Array In"=w1784) -> ("time array out"=w1781:dbl[], "Measurement  array Out"=w1783:dbl[][], "Error Out"=w1785:errorcluster)  [unwired: 10 in, 7 out]
                  }
                }
                n753 = control-ref of="Sonde Data Display"() -> (w1775:refnum<vi>)
                n754 = call "Calibrate ORP Sensor2.vi"("Calibration Standard"="ORP Reference", "Error In (No Error)"=w1762, "Sensor Address In"="0", "RS232 Port In"=w1760) -> ("Error Out"=w1766:errorcluster, "RS232 Port Out"=w1765:refnum<visa-resource-name>, "Calibration Response"=→"ORP Reference Calibration Response":T18)  [unwired: 2 in, 3 out]
                n755 = local read "Sample Sheet Data Row Cluster 2"() -> (w1772:T3)
                n756 = call "SDI-12 Single Operation with output cluster.vi"("RS232 Port In"=w1765, "Sensor Address In"="0", "Sonde Data Ctl Refnum"=w1775, "Error In (No Error)"=w1766, "file directory (dialog if empty)"=w1757, "Save File"=w1756, "Time Array In"=w1761, "Measurement Array In"=w1758) -> ("time array out"=w1770:dbl[], "Measurement  array Out"=w1769:dbl[][], "output cluster"=w1773:T4, "Temperature"=w1777:cluster{"Y":dbl[], "Y":dbl[]}[], "Sonde Data Display"=w1776:T16, "Error Out"=w1774:errorcluster)  [unwired: 10 in, 4 out]
                n757 = Bundle By Name(cluster=w1772, "Sonde Data Cluster"=w1773) -> (w1771:T3)
                n758 = local write "Temperature"(w1777) -> ()
                n759 = local write "Sonde Data Display"(w1776) -> ()
              }
              frame True {
                n760 = Get Date/Time In Seconds() -> (seconds since 1Jan1904=w1798:timestamp)
                n761 = To Double Precision Float(number=w1798) -> (double precision float=w1797:dbl)
                n762 = local read "Sample Sheet Data Row Cluster 2"() -> (w1806:T3)
                n763 = Subtract(x=w1797, y=w1792) -> (x-y=w1790:dbl)
                n764 = local write "Current Time (s)"(w1790) -> ()
                n765 = Unbundle By Name(w1806) -> ("Sonde Data Cluster.Temp deg C"=w1791:dbl, "Sonde Data Cluster.pH"=w1805:dbl, "Sonde Data Cluster.Specific\nCond (mS)"=w1804:dbl, "Sonde Data Cluster.Salinity"=w1803:dbl, "Sonde Data Cluster.Dissolved\nOxygen mg/L"=w1802:dbl, "Sonde Data Cluster.ORP"=w1801:dbl)  [unwired: 1 out]
                n766 = Build Array(w1791, w1805, w1804, w1803, w1802, 0.0 ("element"), w1801) -> (w1799:dbl[])
                n767 = Build Array (concatenate)(w1807, w1799) -> (w1795:dbl[][])
                n768 = Build Array (concatenate)(w1808, w1790) -> (w1796:dbl[])
                n769 = call "format into Sonde Vertical Graph Data Input.vi"("Sonde Measurement Array"=w1795, "Time Array"=w1796) -> ("Sonde Data Display"=w1794:T16, "Temperature"=w1793:cluster{"X":dbl[], "Y":dbl[]}[])  [unwired: 8 in]
                n770 = local write "Temperature"(w1793) -> ()
                n771 = local write "Sonde Data Display"(w1794) -> ()
              }
            }
            n772 = case shown="False" FALSE {
              tunnel: w1696 -> [_ w1733]
              tunnel: w1695 -> [_ w1732]
              tunnel: w1694 -> [w1723 w1731]
              tunnel: w1693 -> [w1722 w1730]
              tunnel: w1691 -> [_ w1729]
              tunnel: [w1723 w1728] -> w1688
              tunnel: [w1722 w1727] -> w1687
              tunnel: w1681 -> [w1721 w1726]
              tunnel: [w1721 w1725] -> w1680
              tunnel: w1663 -> [_ w1724]
              frame False {
              }
              frame True {
                n773 = call "write out sonde row.vi"("NI_report in"=w1730, "Columns"=w1733, "Column of Volume"=w1732, "Sample Sheet Data Row Cluster"=w1729, "row index"=w1726, "error in (no error)"=w1731, "start of last occupied row"=w1724) -> ("NI_report out"=w1727:refnum<class "NI_report.lvclass">, "row index out"=w1725:i32, "error out"=w1728:errorcluster)  [unwired: 6 in]
              }
            }
            n774 = local write "Sample Sheet Data Row Cluster 2"(w1691) -> ()
            n775 = case shown="False" FALSE {
              tunnel: w1688 -> [w1735 w1741]
              tunnel: w1687 -> [w1736 w1740]
              tunnel: [w1736 w1739] -> w1686
              tunnel: [w1735 w1738] -> w1683
              tunnel: [w1734 w1737] -> w1682
              tunnel: w1663 -> [w1734 _]
              frame False {
              }
              frame True {
                n776 = flat-sequence {
                  tunnel: w1741 -> [w1755]
                  tunnel: w1740 -> [w1754]
                  tunnel: [w1753] -> w1739
                  tunnel: [w1748] -> w1738
                  tunnel: [w1746] -> w1737
                  frame #0 {
                    n777 = call <vilib>:"Clear Errors.vi"("error in (no error)"=w1755) -> ("error out"=w1742:errorcluster)  [unwired: 5 in, 1 out]
                    n778 = local read "Current Sample Sheet"() -> (w1744:string)
                    n779 = call "get sample sheet data cells.vi"("error in (no error)"=w1742, "NI_report in"=w1754) -> ("error out"=w1749:errorcluster, "data"=w1750:string[][], "NI_report out"=w1753:refnum<class "NI_report.lvclass">, "left edge output cluster"=w1747:cluster{"row":i32, "column":i32})  [unwired: 5 in, 1 out]
                    n780 = call "find last occupied cell.vi"("data"=w1750, "Active Sheet"=w1744, "Header Rows to remove"=3, "sub array start"=w1747, "error in (no error)"=w1749) -> ("row max value"=w1745:i32, 13:"start of last occupied row"=w1746:cluster{"row":i32, "column":i32}, 14:"start of last occupied row"=w1743:string, "error out"=w1748:errorcluster)  [unwired: 4 in, 3 out]
                    n781 = Array Subset(array=w1750, index (col)=2 ("index")) -> ()  [unwired: 3 in, 1 out]
                    n782 = local write "row max value"(w1745) -> ()
                    n783 = local write "last occupied cell's name"(w1743) -> ()
                  }
                }
              }
            }
          }
          frame "Salinity Calibration Standard" {
            n784 = invoke on="Record Single Sample" class="Bool" method="Reinit To Default"(error in=w1835) -> (error out=w1834:errorcluster)  [unwired: 2 in, 2 out]
            n785 = call <vilib>:"Clear Errors.vi"("error in (no error)"=w1834) -> ("error out"=w1822:errorcluster)  [unwired: 5 in, 1 out]
            n786 = case shown="False" FALSE {
              tunnel: w1849 -> [w1852 w1860]
              tunnel: [w1851 w1856] -> w1848
              tunnel: [w1852 w1855] -> w1844
              tunnel: w1822 -> [w1851 w1854]
              tunnel: [w1850 w1853] -> w1812
              tunnel: w1810 -> [w1850 _]
              frame False {
              }
              frame True {
                n787 = call "get sample sheet data cells.vi"("error in (no error)"=w1854, "NI_report in"=w1860) -> ("error out"=w1857:errorcluster, "data"=w1859:string[][], "NI_report out"=w1855:refnum<class "NI_report.lvclass">, "left edge output cluster"=w1858:cluster{"row":i32, "column":i32})  [unwired: 5 in, 1 out]
                n788 = flat-sequence {
                  tunnel: w1857 -> [w1871]
                  tunnel: [w1864] -> _
                  tunnel: w1858 -> [w1869]
                  tunnel: [w1868] -> w1856
                  tunnel: [w1867] -> _
                  tunnel: [w1866] -> w1853
                  tunnel: w1859 -> [w1864]
                  frame #0 {
                    n789 = Array Subset(array=w1864, index (col)=2 ("index")) -> ()  [unwired: 3 in, 1 out]
                    n790 = local read "Current Sample Sheet"() -> (w1863:string)
                    n791 = call "find last occupied cell.vi"("data"=w1864, "Active Sheet"=w1863, "Header Rows to remove"=3, "sub array start"=w1869, "error in (no error)"=w1871) -> ("row max value"=w1867:i32, "column max value"=w1862:i32, 13:"start of last occupied row"=w1866:cluster{"row":i32, "column":i32}, 14:"start of last occupied row"=w1861:string, "error out"=w1868:errorcluster)  [unwired: 4 in, 2 out]
                    n792 = local write "last occupied cell's name"(w1861) -> ()
                    n793 = local write "row max value"(w1862) -> ()
                  }
                }
              }
            }
            n794 = local read "Found Quanta Sonde Com Port"() -> (w1839:refnum<visa-resource-name>)
            n795 = Equal?(x=w1839, y=refnum<visa-resource-name> refnum ("RS232 Port Out")) -> (x = y?=w1841:bool)
            n796 = case shown="False" w1841 {
              tunnel: w1839 -> [w1912 _]
              tunnel: [w1923 w1958] -> w1842
              tunnel: w1848 -> [w1915 w1961]
              tunnel: [w1926 w1961] -> w1845
              tunnel: w1829 -> [w1914 w1960]
              tunnel: [w1922 w1948] -> w1828
              tunnel: [w1921 w1947] -> w1827
              tunnel: w1826 -> [w1911 w1959]
              tunnel: w1825 -> [_ w1944]
              frame False {
                n797 = flat-sequence {
                  tunnel: w1912 -> [w1941]
                  tunnel: [w1940] -> _
                  tunnel: w1915 -> [w1938]
                  tunnel: [w1937] -> w1909
                  tunnel: w1911 -> [w1936]
                  tunnel: [w1935] -> w1910
                  tunnel: w1914 -> [w1934]
                  tunnel: [w1933] -> w1913
                  tunnel: [w1932] -> w1908
                  tunnel: [w1931] -> w1907
                  frame #0 {
                    w1931 = TRUE ("Save File")
                    n798 = local read "Sonde Calibration History File"() -> (w1932:path)
                    n799 = control-ref of="Sonde Data Display"() -> (w1940:refnum<vi>)
                    n800 = call "SDI-12 Single Operation with output cluster.vi"("RS232 Port In"=w1941, "Sensor Address In"="0", "Sonde Data Ctl Refnum"=w1940, "Error In (No Error)"=w1938, "file directory (dialog if empty)"=w1932, "Save File"=w1931, "Time Array In"=w1934, "Measurement Array In"=w1936) -> ("time array out"=w1933:dbl[], "Measurement  array Out"=w1935:dbl[][], "Error Out"=w1937:errorcluster)  [unwired: 10 in, 7 out]
                  }
                }
                n801 = call "Calibrate Salinity Sensor2.vi"("Calibration Standard"="Salinity \nReference", "Error In (No Error)"=w1909, "Sensor Address In"="0", "RS232 Port In"=w1912) -> ("Error Out"=w1918:errorcluster, "RS232 Port Out"=w1919:refnum<visa-resource-name>, "Calibration Response"=→"Salinity Reference Calibration Response":T18)  [unwired: 2 in, 3 out]
                n802 = control-ref of="Sonde Data Display"() -> (w1927:refnum<vi>)
                n803 = local read "Sample Sheet Data Row Cluster 2"() -> (w1924:T3)
                n804 = call "SDI-12 Single Operation with output cluster.vi"("RS232 Port In"=w1919, "Sensor Address In"="0", "Sonde Data Ctl Refnum"=w1927, "Error In (No Error)"=w1918, "file directory (dialog if empty)"=w1908, "Save File"=w1907, "Time Array In"=w1913, "Measurement Array In"=w1910) -> ("time array out"=w1922:dbl[], "Measurement  array Out"=w1921:dbl[][], "output cluster"=w1925:T4, "Temperature"=w1929:cluster{"Y":dbl[], "Y":dbl[]}[], "Sonde Data Display"=w1928:T16, "Error Out"=w1926:errorcluster)  [unwired: 10 in, 4 out]
                n805 = local write "Temperature"(w1929) -> ()
                n806 = local write "Sonde Data Display"(w1928) -> ()
                n807 = Bundle By Name(cluster=w1924, "Sonde Data Cluster"=w1925) -> (w1923:T3)
              }
              frame True {
                n808 = Get Date/Time In Seconds() -> (seconds since 1Jan1904=w1950:timestamp)
                n809 = To Double Precision Float(number=w1950) -> (double precision float=w1949:dbl)
                n810 = local read "Sample Sheet Data Row Cluster 2"() -> (w1958:T3)
                n811 = Subtract(x=w1949, y=w1944) -> (x-y=w1942:dbl)
                n812 = local write "Current Time (s)"(w1942) -> ()
                n813 = Unbundle By Name(w1958) -> ("Sonde Data Cluster.Temp deg C"=w1943:dbl, "Sonde Data Cluster.pH"=w1957:dbl, "Sonde Data Cluster.Specific\nCond (mS)"=w1956:dbl, "Sonde Data Cluster.Salinity"=w1955:dbl, "Sonde Data Cluster.Dissolved\nOxygen mg/L"=w1954:dbl, "Sonde Data Cluster.ORP"=w1953:dbl)  [unwired: 1 out]
                n814 = Build Array(w1943, w1957, w1956, w1955, w1954, 0.0 ("element"), w1953) -> (w1951:dbl[])
                n815 = Build Array (concatenate)(w1959, w1951) -> (w1947:dbl[][])
                n816 = Build Array (concatenate)(w1960, w1942) -> (w1948:dbl[])
                n817 = call "format into Sonde Vertical Graph Data Input.vi"("Sonde Measurement Array"=w1947, "Time Array"=w1948) -> ("Sonde Data Display"=w1946:T16, "Temperature"=w1945:cluster{"X":dbl[], "Y":dbl[]}[])  [unwired: 8 in]
                n818 = local write "Temperature"(w1945) -> ()
                n819 = local write "Sonde Data Display"(w1946) -> ()
              }
            }
            n820 = local write "Sample Sheet Data Row Cluster 2"(w1842) -> ()
            n821 = case shown="False" FALSE {
              tunnel: w1847 -> [_ w1884]
              tunnel: w1846 -> [_ w1883]
              tunnel: w1845 -> [w1874 w1882]
              tunnel: w1844 -> [w1872 w1881]
              tunnel: w1812 -> [_ w1880]
              tunnel: w1842 -> [_ w1879]
              tunnel: [w1874 w1878] -> w1838
              tunnel: [w1872 w1877] -> w1837
              tunnel: w1831 -> [w1873 w1876]
              tunnel: [w1873 w1875] -> w1830
              frame False {
              }
              frame True {
                n822 = call "write out sonde row.vi"("NI_report in"=w1881, "Columns"=w1884, "Column of Volume"=w1883, "Sample Sheet Data Row Cluster"=w1879, "row index"=w1876, "error in (no error)"=w1882, "start of last occupied row"=w1880) -> ("NI_report out"=w1877:refnum<class "NI_report.lvclass">, "row index out"=w1875:i32, "error out"=w1878:errorcluster)  [unwired: 6 in]
              }
            }
            n823 = case shown="False" FALSE {
              tunnel: w1838 -> [w1887 w1892]
              tunnel: w1837 -> [w1886 w1891]
              tunnel: [w1886 w1890] -> w1836
              tunnel: [w1887 w1889] -> w1833
              tunnel: [w1885 w1888] -> w1832
              tunnel: w1812 -> [w1885 _]
              frame False {
              }
              frame True {
                n824 = flat-sequence {
                  tunnel: w1892 -> [w1906]
                  tunnel: w1891 -> [w1905]
                  tunnel: [w1904] -> w1890
                  tunnel: [w1899] -> w1889
                  tunnel: [w1897] -> w1888
                  frame #0 {
                    n825 = call <vilib>:"Clear Errors.vi"("error in (no error)"=w1906) -> ("error out"=w1893:errorcluster)  [unwired: 5 in, 1 out]
                    n826 = local read "Current Sample Sheet"() -> (w1895:string)
                    n827 = call "get sample sheet data cells.vi"("error in (no error)"=w1893, "NI_report in"=w1905) -> ("error out"=w1900:errorcluster, "data"=w1901:string[][], "NI_report out"=w1904:refnum<class "NI_report.lvclass">, "left edge output cluster"=w1898:cluster{"row":i32, "column":i32})  [unwired: 5 in, 1 out]
                    n828 = call "find last occupied cell.vi"("data"=w1901, "Active Sheet"=w1895, "Header Rows to remove"=3, "sub array start"=w1898, "error in (no error)"=w1900) -> ("row max value"=w1896:i32, 13:"start of last occupied row"=w1897:cluster{"row":i32, "column":i32}, 14:"start of last occupied row"=w1894:string, "error out"=w1899:errorcluster)  [unwired: 4 in, 3 out]
                    n829 = Array Subset(array=w1901, index (col)=2 ("index")) -> ()  [unwired: 3 in, 1 out]
                    n830 = local write "row max value"(w1896) -> ()
                    n831 = local write "last occupied cell's name"(w1894) -> ()
                  }
                }
              }
            }
          }
          frame "DO Calibration Standard" {
            n832 = invoke on="Record Single Sample" class="Bool" method="Reinit To Default"(error in=w1985) -> (error out=w1984:errorcluster)  [unwired: 2 in, 2 out]
            n833 = call <vilib>:"Clear Errors.vi"("error in (no error)"=w1984) -> ("error out"=w1972:errorcluster)  [unwired: 5 in, 1 out]
            n834 = case shown="True" FALSE {
              tunnel: w1998 -> [w2000 w2009]
              tunnel: [w2001 w2005] -> w1997
              tunnel: [w2000 w2004] -> w1993
              tunnel: [w1999 w2003] -> w1991
              tunnel: w1972 -> [w2001 w2002]
              tunnel: w1962 -> [w1999 _]
              frame False {
              }
              frame True {
                n835 = call "get sample sheet data cells.vi"("error in (no error)"=w2002, "NI_report in"=w2009) -> ("error out"=w2006:errorcluster, "data"=w2008:string[][], "NI_report out"=w2004:refnum<class "NI_report.lvclass">, "left edge output cluster"=w2007:cluster{"row":i32, "column":i32})  [unwired: 5 in, 1 out]
                n836 = flat-sequence {
                  tunnel: w2006 -> [w2020]
                  tunnel: [w2013] -> _
                  tunnel: w2007 -> [w2018]
                  tunnel: [w2017] -> w2005
                  tunnel: [w2016] -> _
                  tunnel: [w2015] -> w2003
                  tunnel: w2008 -> [w2013]
                  frame #0 {
                    n837 = local read "Current Sample Sheet"() -> (w2012:string)
                    n838 = Array Subset(array=w2013, index (col)=2 ("index")) -> ()  [unwired: 3 in, 1 out]
                    n839 = call "find last occupied cell.vi"("data"=w2013, "Active Sheet"=w2012, "Header Rows to remove"=3, "sub array start"=w2018, "error in (no error)"=w2020) -> ("row max value"=w2016:i32, "column max value"=w2011:i32, 13:"start of last occupied row"=w2015:cluster{"row":i32, "column":i32}, 14:"start of last occupied row"=w2010:string, "error out"=w2017:errorcluster)  [unwired: 4 in, 2 out]
                    n840 = local write "last occupied cell's name"(w2010) -> ()
                    n841 = local write "row max value"(w2011) -> ()
                  }
                }
              }
            }
            n842 = local read "Found Quanta Sonde Com Port"() -> (w1987:refnum<visa-resource-name>)
            n843 = Equal?(x=w1987, y=refnum<visa-resource-name> refnum ("RS232 Port Out")) -> (x = y?=w1989:bool)
            n844 = case shown="False" w1989 {
              tunnel: w1987 -> [w2060 _]
              tunnel: [w2068 w2102] -> w1990
              tunnel: w1997 -> [w2058 w2105]
              tunnel: [w2071 w2105] -> w1994
              tunnel: w1979 -> [w2054 w2104]
              tunnel: [w2067 w2092] -> w1978
              tunnel: [w2066 w2091] -> w1977
              tunnel: w1976 -> [w2056 w2103]
              tunnel: w1975 -> [_ w2088]
              frame False {
                n845 = flat-sequence {
                  tunnel: w2060 -> [w2085]
                  tunnel: [w2084] -> w2059
                  tunnel: w2058 -> [w2082]
                  tunnel: [w2081] -> w2057
                  tunnel: w2056 -> [w2080]
                  tunnel: [w2079] -> w2055
                  tunnel: w2054 -> [w2078]
                  tunnel: [w2077] -> w2053
                  tunnel: [w2076] -> w2052
                  tunnel: [w2075] -> w2051
                  frame #0 {
                    w2075 = TRUE ("Save File")
                    n846 = local read "Sonde Calibration History File"() -> (w2076:path)
                    n847 = control-ref of="Sonde Data Display"() -> (w2084:refnum<vi>)
                    n848 = call "SDI-12 Single Operation with output cluster.vi"("RS232 Port In"=w2085, "Sensor Address In"="0", "Sonde Data Ctl Refnum"=w2084, "Error In (No Error)"=w2082, "file directory (dialog if empty)"=w2076, "Save File"=w2075, "Time Array In"=w2078, "Measurement Array In"=w2080) -> ("time array out"=w2077:dbl[], "Measurement  array Out"=w2079:dbl[][], "Error Out"=w2081:errorcluster)  [unwired: 10 in, 7 out]
                  }
                }
                n849 = call "Calibrate DO Sensor2.vi"("Calibration Standard"="DO Reference %", "Error In (No Error)"=w2057, "Sensor Address In"="0", "RS232 Port In"=w2060) -> ("Error Out"=w2065:errorcluster, "RS232 Port Out"=w2064:refnum<visa-resource-name>, "Calibration Response"=→"DO Reference % Calibration Response":T18)  [unwired: 2 in, 3 out]
                n850 = call "SDI-12 Single Operation with output cluster.vi"("RS232 Port In"=w2064, "Sensor Address In"="0", "Sonde Data Ctl Refnum"=w2059, "Error In (No Error)"=w2065, "file directory (dialog if empty)"=w2052, "Save File"=w2051, "Time Array In"=w2053, "Measurement Array In"=w2055) -> ("time array out"=w2067:dbl[], "Measurement  array Out"=w2066:dbl[][], "output cluster"=w2070:T4, "Temperature"=w2073:cluster{"Y":dbl[], "Y":dbl[]}[], "Sonde Data Display"=w2072:T16, "Error Out"=w2071:errorcluster)  [unwired: 10 in, 4 out]
                n851 = local read "Sample Sheet Data Row Cluster 2"() -> (w2069:T3)
                n852 = local write "Temperature"(w2073) -> ()
                n853 = local write "Sonde Data Display"(w2072) -> ()
                n854 = Bundle By Name(cluster=w2069, "Sonde Data Cluster"=w2070) -> (w2068:T3)
              }
              frame True {
                n855 = Get Date/Time In Seconds() -> (seconds since 1Jan1904=w2094:timestamp)
                n856 = To Double Precision Float(number=w2094) -> (double precision float=w2093:dbl)
                n857 = local read "Sample Sheet Data Row Cluster 2"() -> (w2102:T3)
                n858 = Subtract(x=w2093, y=w2088) -> (x-y=w2086:dbl)
                n859 = local write "Current Time (s)"(w2086) -> ()
                n860 = Unbundle By Name(w2102) -> ("Sonde Data Cluster.Temp deg C"=w2087:dbl, "Sonde Data Cluster.pH"=w2101:dbl, "Sonde Data Cluster.Specific\nCond (mS)"=w2100:dbl, "Sonde Data Cluster.Salinity"=w2099:dbl, "Sonde Data Cluster.Dissolved\nOxygen mg/L"=w2098:dbl, "Sonde Data Cluster.ORP"=w2097:dbl)  [unwired: 1 out]
                n861 = Build Array(w2087, w2101, w2100, w2099, w2098, 0.0 ("element"), w2097) -> (w2095:dbl[])
                n862 = Build Array (concatenate)(w2103, w2095) -> (w2091:dbl[][])
                n863 = Build Array (concatenate)(w2104, w2086) -> (w2092:dbl[])
                n864 = call "format into Sonde Vertical Graph Data Input.vi"("Sonde Measurement Array"=w2091, "Time Array"=w2092) -> ("Sonde Data Display"=w2090:T16, "Temperature"=w2089:cluster{"X":dbl[], "Y":dbl[]}[])  [unwired: 8 in]
                n865 = local write "Temperature"(w2089) -> ()
                n866 = local write "Sonde Data Display"(w2090) -> ()
              }
            }
            n867 = local write "Sample Sheet Data Row Cluster 2"(w1990) -> ()
            n868 = case shown="False" FALSE {
              tunnel: w1996 -> [_ w2037]
              tunnel: w1995 -> [_ w2036]
              tunnel: w1994 -> [w2023 w2035]
              tunnel: w1993 -> [w2024 w2034]
              tunnel: w1991 -> [w2022 w2033]
              tunnel: w1990 -> [_ w2032]
              tunnel: [w2024 w2029] -> w1986
              tunnel: [w2023 w2028] -> w1983
              tunnel: [w2022 w2027] -> w1982
              tunnel: w1981 -> [w2021 w2026]
              tunnel: [w2021 w2025] -> w1980
              frame False {
              }
              frame True {
                n869 = call "write out sonde row.vi"("NI_report in"=w2034, "Columns"=w2037, "Column of Volume"=w2036, "Sample Sheet Data Row Cluster"=w2032, "row index"=w2026, "error in (no error)"=w2035, "start of last occupied row"=w2033) -> ("NI_report out"=w2030:refnum<class "NI_report.lvclass">, "row index out"=w2025:i32, "error out"=w2031:errorcluster)  [unwired: 6 in]
                n870 = flat-sequence {
                  tunnel: w2031 -> [w2050]
                  tunnel: w2030 -> [w2049]
                  tunnel: [w2048] -> w2029
                  tunnel: [w2044] -> w2028
                  tunnel: [w2042] -> w2027
                  frame #0 {
                    n871 = call <vilib>:"Clear Errors.vi"("error in (no error)"=w2050) -> ("error out"=w2038:errorcluster)  [unwired: 5 in, 1 out]
                    n872 = local read "Current Sample Sheet"() -> (w2040:string)
                    n873 = call "get sample sheet data cells.vi"("error in (no error)"=w2038, "NI_report in"=w2049) -> ("error out"=w2045:errorcluster, "data"=w2046:string[][], "NI_report out"=w2048:refnum<class "NI_report.lvclass">, "left edge output cluster"=w2043:cluster{"row":i32, "column":i32})  [unwired: 5 in, 1 out]
                    n874 = call "find last occupied cell.vi"("data"=w2046, "Active Sheet"=w2040, "Header Rows to remove"=3, "sub array start"=w2043, "error in (no error)"=w2045) -> ("row max value"=w2041:i32, 13:"start of last occupied row"=w2042:cluster{"row":i32, "column":i32}, 14:"start of last occupied row"=w2039:string, "error out"=w2044:errorcluster)  [unwired: 4 in, 3 out]
                    n875 = local write "row max value"(w2041) -> ()
                    n876 = local write "last occupied cell's name"(w2039) -> ()
                  }
                }
              }
            }
          }
          frame "SC Calibration Standard" {
            n877 = invoke on="Record Single Sample" class="Bool" method="Reinit To Default"(error in=w2129) -> (error out=w2128:errorcluster)  [unwired: 2 in, 2 out]
            n878 = call <vilib>:"Clear Errors.vi"("error in (no error)"=w2128) -> ("error out"=w2116:errorcluster)  [unwired: 5 in, 1 out]
            n879 = case shown="True" FALSE {
              tunnel: w2142 -> [w2145 w2153]
              tunnel: [w2144 w2149] -> w2141
              tunnel: [w2145 w2148] -> w2137
              tunnel: [w2143 w2147] -> w2135
              tunnel: w2116 -> [w2144 w2146]
              tunnel: w2106 -> [w2143 _]
              frame False {
              }
              frame True {
                n880 = call "get sample sheet data cells.vi"("error in (no error)"=w2146, "NI_report in"=w2153) -> ("error out"=w2150:errorcluster, "data"=w2152:string[][], "NI_report out"=w2148:refnum<class "NI_report.lvclass">, "left edge output cluster"=w2151:cluster{"row":i32, "column":i32})  [unwired: 5 in, 1 out]
                n881 = flat-sequence {
                  tunnel: w2150 -> [w2163]
                  tunnel: w2151 -> [w2161]
                  tunnel: [w2160] -> w2149
                  tunnel: [w2159] -> _
                  tunnel: [w2158] -> w2147
                  tunnel: w2152 -> [w2157]
                  frame #0 {
                    n882 = local read "Current Sample Sheet"() -> (w2156:string)
                    n883 = call "find last occupied cell.vi"("data"=w2157, "Active Sheet"=w2156, "Header Rows to remove"=3, "sub array start"=w2161, "error in (no error)"=w2163) -> ("row max value"=w2159:i32, "column max value"=w2155:i32, 13:"start of last occupied row"=w2158:cluster{"row":i32, "column":i32}, 14:"start of last occupied row"=w2154:string, "error out"=w2160:errorcluster)  [unwired: 4 in, 2 out]
                    n884 = local write "last occupied cell's name"(w2154) -> ()
                    n885 = local write "row max value"(w2155) -> ()
                  }
                }
              }
            }
            n886 = local read "Found Quanta Sonde Com Port"() -> (w2131:refnum<visa-resource-name>)
            n887 = Equal?(x=w2131, y=refnum<visa-resource-name> refnum ("RS232 Port Out")) -> (x = y?=w2133:bool)
            n888 = case shown="False" w2133 {
              tunnel: w2131 -> [w2202 _]
              tunnel: [w2211 w2246] -> w2134
              tunnel: w2141 -> [w2201 w2249]
              tunnel: [w2214 w2249] -> w2138
              tunnel: w2123 -> [w2199 w2248]
              tunnel: [w2210 w2236] -> w2122
              tunnel: [w2209 w2235] -> w2121
              tunnel: w2120 -> [w2197 w2247]
              tunnel: w2119 -> [_ w2232]
              frame False {
                n889 = flat-sequence {
                  tunnel: w2202 -> [w2229]
                  tunnel: [w2228] -> _
                  tunnel: w2201 -> [w2226]
                  tunnel: [w2225] -> w2200
                  tunnel: w2197 -> [w2224]
                  tunnel: [w2223] -> w2196
                  tunnel: w2199 -> [w2222]
                  tunnel: [w2221] -> w2198
                  tunnel: [w2220] -> w2195
                  tunnel: [w2219] -> w2194
                  frame #0 {
                    w2219 = TRUE ("Save File")
                    n890 = local read "Sonde Calibration History File"() -> (w2220:path)
                    n891 = control-ref of="Sonde Data Display"() -> (w2228:refnum<vi>)
                    n892 = call "SDI-12 Single Operation with output cluster.vi"("RS232 Port In"=w2229, "Sensor Address In"="0", "Sonde Data Ctl Refnum"=w2228, "Error In (No Error)"=w2226, "file directory (dialog if empty)"=w2220, "Save File"=w2219, "Time Array In"=w2222, "Measurement Array In"=w2224) -> ("time array out"=w2221:dbl[], "Measurement  array Out"=w2223:dbl[][], "Error Out"=w2225:errorcluster)  [unwired: 10 in, 7 out]
                  }
                }
                n893 = call "Calibrate SC Sensor2.vi"("SC Calibration Standard uS/cm"="SC \nReference (uS/cm)", "Error In (No Error)"=w2200, "Sensor Address In"="0", "RS232 Port In"=w2202) -> ("Error Out"=w2206:errorcluster, "RS232 Port Out"=w2207:refnum<visa-resource-name>, "Calibration Response"=→"SC Reference (uS/cm) Calibration Response":T18)  [unwired: 2 in, 3 out]
                n894 = control-ref of="Sonde Data Display"() -> (w2215:refnum<vi>)
                n895 = local read "Sample Sheet Data Row Cluster 2"() -> (w2212:T3)
                n896 = call <vilib>:"Clear Errors.vi"("error in (no error)"=w2206) -> ("error out"=w2204:errorcluster)  [unwired: 5 in, 1 out]
                n897 = call "SDI-12 Single Operation with output cluster.vi"("RS232 Port In"=w2207, "Sensor Address In"="0", "Sonde Data Ctl Refnum"=w2215, "Error In (No Error)"=w2204, "file directory (dialog if empty)"=w2195, "Save File"=w2194, "Time Array In"=w2198, "Measurement Array In"=w2196) -> ("time array out"=w2210:dbl[], "Measurement  array Out"=w2209:dbl[][], "output cluster"=w2213:T4, "Temperature"=w2217:cluster{"Y":dbl[], "Y":dbl[]}[], "Sonde Data Display"=w2216:T16, "Error Out"=w2214:errorcluster)  [unwired: 10 in, 4 out]
                n898 = local write "Temperature"(w2217) -> ()
                n899 = local write "Sonde Data Display"(w2216) -> ()
                n900 = Bundle By Name(cluster=w2212, "Sonde Data Cluster"=w2213) -> (w2211:T3)
              }
              frame True {
                n901 = Get Date/Time In Seconds() -> (seconds since 1Jan1904=w2238:timestamp)
                n902 = To Double Precision Float(number=w2238) -> (double precision float=w2237:dbl)
                n903 = local read "Sample Sheet Data Row Cluster 2"() -> (w2246:T3)
                n904 = Subtract(x=w2237, y=w2232) -> (x-y=w2230:dbl)
                n905 = local write "Current Time (s)"(w2230) -> ()
                n906 = Unbundle By Name(w2246) -> ("Sonde Data Cluster.Temp deg C"=w2231:dbl, "Sonde Data Cluster.pH"=w2245:dbl, "Sonde Data Cluster.Specific\nCond (mS)"=w2244:dbl, "Sonde Data Cluster.Salinity"=w2243:dbl, "Sonde Data Cluster.Dissolved\nOxygen mg/L"=w2242:dbl, "Sonde Data Cluster.ORP"=w2241:dbl)  [unwired: 1 out]
                n907 = Build Array(w2231, w2245, w2244, w2243, w2242, 0.0 ("element"), w2241) -> (w2239:dbl[])
                n908 = Build Array (concatenate)(w2247, w2239) -> (w2235:dbl[][])
                n909 = Build Array (concatenate)(w2248, w2230) -> (w2236:dbl[])
                n910 = call "format into Sonde Vertical Graph Data Input.vi"("Sonde Measurement Array"=w2235, "Time Array"=w2236) -> ("Sonde Data Display"=w2234:T16, "Temperature"=w2233:cluster{"X":dbl[], "Y":dbl[]}[])  [unwired: 8 in]
                n911 = local write "Temperature"(w2233) -> ()
                n912 = local write "Sonde Data Display"(w2234) -> ()
              }
            }
            n913 = local write "Sample Sheet Data Row Cluster 2"(w2134) -> ()
            n914 = case shown="False" FALSE {
              tunnel: w2140 -> [_ w2180]
              tunnel: w2139 -> [_ w2179]
              tunnel: w2138 -> [w2166 w2178]
              tunnel: w2137 -> [w2165 w2177]
              tunnel: w2135 -> [w2164 w2176]
              tunnel: w2134 -> [_ w2175]
              tunnel: [w2165 w2172] -> w2130
              tunnel: [w2166 w2171] -> w2127
              tunnel: [w2164 w2170] -> w2126
              tunnel: w2125 -> [w2167 w2169]
              tunnel: [w2167 w2168] -> w2124
              frame False {
              }
              frame True {
                n915 = call "write out sonde row.vi"("NI_report in"=w2177, "Columns"=w2180, "Column of Volume"=w2179, "Sample Sheet Data Row Cluster"=w2175, "row index"=w2169, "error in (no error)"=w2178, "start of last occupied row"=w2176) -> ("NI_report out"=w2173:refnum<class "NI_report.lvclass">, "row index out"=w2168:i32, "error out"=w2174:errorcluster)  [unwired: 6 in]
                n916 = flat-sequence {
                  tunnel: w2174 -> [w2193]
                  tunnel: w2173 -> [w2192]
                  tunnel: [w2191] -> w2172
                  tunnel: [w2187] -> w2171
                  tunnel: [w2185] -> w2170
                  frame #0 {
                    (unwired) 2 ("index")
                    n917 = call <vilib>:"Clear Errors.vi"("error in (no error)"=w2193) -> ("error out"=w2181:errorcluster)  [unwired: 5 in, 1 out]
                    n918 = local read "Current Sample Sheet"() -> (w2183:string)
                    n919 = call "get sample sheet data cells.vi"("error in (no error)"=w2181, "NI_report in"=w2192) -> ("error out"=w2188:errorcluster, "data"=w2189:string[][], "NI_report out"=w2191:refnum<class "NI_report.lvclass">, "left edge output cluster"=w2186:cluster{"row":i32, "column":i32})  [unwired: 5 in, 1 out]
                    n920 = call "find last occupied cell.vi"("data"=w2189, "Active Sheet"=w2183, "Header Rows to remove"=3, "sub array start"=w2186, "error in (no error)"=w2188) -> ("row max value"=w2184:i32, 13:"start of last occupied row"=w2185:cluster{"row":i32, "column":i32}, 14:"start of last occupied row"=w2182:string, "error out"=w2187:errorcluster)  [unwired: 4 in, 3 out]
                    n921 = local write "row max value"(w2184) -> ()
                    n922 = local write "last occupied cell's name"(w2182) -> ()
                  }
                }
              }
            }
          }
          frame "Write Sonde Sample Sheet" {
            n923 = flat-sequence {
              tunnel: w2276 -> [w2295]
              tunnel: w2275 -> [w2282]
              tunnel: w2273 -> [w2292]
              tunnel: w2272 -> [w2291]
              tunnel: w2271 -> [w2290]
              tunnel: [w2289] -> w2270
              tunnel: w2269 -> [w2288]
              tunnel: w2268 -> [w2287]
              tunnel: w2250 -> [w2285]
              tunnel: [w2284] -> w2266
              tunnel: [w2283] -> w2265
              tunnel: [w2278] -> w2264
              tunnel: w2253 -> [w2280]
              frame #0 {
                n924 = call <vilib>:"Clear Errors.vi"("error in (no error)"=w2282) -> ("error out"=w2277:errorcluster)  [unwired: 5 in, 1 out]
                n925 = Not Equal?(x=w2288, y=w2287) -> (x != y?=w2286:bool)
                n926 = invoke on="Update Sonde" class="Bool (strict)" method="Reinit To Default"(error in=w2277) -> (error out=w2281:errorcluster)  [unwired: 2 in, 2 out]
                n927 = case shown="True" w2286 {
                  tunnel: w2295 -> [w2309 w2331]
                  tunnel: w2285 -> [_ w2330]
                  tunnel: w2281 -> [w2308 w2329]
                  tunnel: [w2308 w2317] -> w2294
                  tunnel: [w2309 w2328] -> w2293
                  tunnel: w2290 -> [w2307 w2313]
                  tunnel: [w2307 w2312] -> w2289
                  tunnel: w2280 -> [w2306 w2311]
                  tunnel: [w2306 w2316] -> w2278
                  frame False {
                  }
                  frame True {
                    n928 = local read "Sonde Data Array"() -> (w2315:T13)
                    n929 = Decrement(x=w2311) -> (x-1=w2310:i32)
                    "Sonde Array Size" <- w2310
                    n930 = flat-sequence {
                      tunnel: [w2345] -> w2328
                      tunnel: w2331 -> [w2344]
                      tunnel: w2330 -> [w2343]
                      tunnel: w2329 -> [w2342]
                      tunnel: [w2341] -> w2322
                      frame #0 {
                        n931 = case shown="True" FALSE {
                          tunnel: [w2347 w2354] -> w2345
                          tunnel: w2344 -> [w2347 w2353]
                          tunnel: w2343 -> [_ w2350]
                          tunnel: w2342 -> [w2346 w2349]
                          tunnel: [w2346 w2348] -> w2341
                          frame False {
                          }
                          frame True {
                            n932 = call "write comment cell with column offset.vi"("Column Relative?"=TRUE, "comment string"="done", "error in (no error)"=w2349, "start of last occupied row"=w2350, "NI_report in"=w2353) -> ("error out"=w2348:errorcluster, "NI_report out"=w2354:refnum<class "NI_report.lvclass">)  [unwired: 5 in]
                          }
                        }
                      }
                    }
                    n933 = Index Array(array=w2315, index=w2310) -> (element=w2327:T14)
                    n934 = Bundle By Name(cluster=w2327, "Final"=TRUE) -> (w2326:T14)
                    n935 = Replace Array Subset(array=w2315, new element=w2326, index=w2310) -> (w2324:T13)
                    n936 = local write "Sonde Data Array"(w2324) -> ()
                    n937 = for {
                      tunnel: w2324 -> [w2339] mode=indexing
                      tunnel: w2313 -> [w2338]
                      tunnel: [w2337] -> w2323 mode=indexing
                      n938 = call "convert sonde cluster to spreadsheet array.vi"("Cluster"=w2339, "Sheet"=w2338) -> ("Sonde Data Array (String)"=w2337:string[])  [unwired: 6 in, 3 out]
                    }
                    n939 = local read "Sonde Output File Path"() -> (w2319:path)
                    n940 = call <vilib>:"Clear Errors.vi"("error in (no error)"=w2322) -> ("error out"=w2314:errorcluster)  [unwired: 5 in, 1 out]
                    n941 = flat-sequence {
                      tunnel: w2318 -> [w2336]
                      tunnel: [w2335] -> w2317
                      tunnel: [0 ("row index")] -> w2316
                      tunnel: w2313 -> [w2333]
                      tunnel: [w2332] -> w2312
                      tunnel: w2310 -> [_]
                      frame #0 {
                        n942 = invoke on="Sonde Data Array" class="Arr (strict)" method="Reinit To Default"(error in=w2336) -> (error out=w2335:errorcluster)  [unwired: 2 in, 2 out]
                        n943 = Increment(x=w2333) -> (x+1=w2332:i32)
                      }
                    }
                    n944 = call-poly <vilib>:"Write Delimited Spreadsheet.vi"("file path (dialog if empty)"=w2319, "2D data"=w2323, "append to file? (new file:F)"=TRUE, "error in (no error)"=w2314, "delimiter (\\t)"="," ("delimiter (\\t)")) -> ("error out"=w2318:errorcluster)  [unwired: 9 in, 1 out]
                  }
                }
                n945 = case shown="True" FALSE {
                  tunnel: w2294 -> [w2297 w2305]
                  tunnel: w2293 -> [w2296 w2304]
                  tunnel: w2292 -> [_ w2303]
                  tunnel: w2291 -> [_ w2302]
                  tunnel: w2289 -> [_ w2301]
                  tunnel: [w2297 w2299] -> w2284
                  tunnel: [w2296 w2298] -> w2283
                  frame False {
                  }
                  frame True {
                    n946 = call "open select sample sheet.vi"("Number of Sample Sheets"=w2302, "error in (no error)"=w2305, "Worksheet Names"=w2303, "input 1"=w2301, "NI_report in"=w2304) -> ("error out"=w2299:errorcluster, "Current Sample Sheet"=w2300:string, "NI_report out"=w2298:refnum<class "NI_report.lvclass">)  [unwired: 4 in]
                    n947 = local write "Current Sample Sheet"(w2300) -> ()
                  }
                }
              }
            }
            n948 = flat-sequence {
              tunnel: [w2357] -> w2274
              tunnel: [w2361] -> w2267
              tunnel: w2266 -> [w2360]
              tunnel: w2265 -> [w2359]
              tunnel: [w2358] -> w2259
              tunnel: w2250 -> [w2355]
              frame #0 {
                n949 = case shown="True" FALSE {
                  tunnel: [w2364 w2376] -> w2361
                  tunnel: w2360 -> [w2362 w2375]
                  tunnel: w2359 -> [w2363 w2374]
                  tunnel: [w2362 w2366] -> w2358
                  tunnel: [w2363 w2365] -> w2357
                  tunnel: w2355 -> [w2364 _]
                  frame False {
                  }
                  frame True {
                    n950 = local read "Current Sample Sheet"() -> (w2368:string)
                    n951 = call "get sample sheet data cells.vi"("error in (no error)"=w2375, "NI_report in"=w2374) -> ("error out"=w2377:errorcluster, "data"=w2372:string[][], "NI_report out"=w2365:refnum<class "NI_report.lvclass">, "left edge output cluster"=w2370:cluster{"row":i32, "column":i32})  [unwired: 5 in, 1 out]
                    n952 = Array Subset(array=w2372, index (col)=2 ("index")) -> ()  [unwired: 3 in, 1 out]
                    n953 = call "find last occupied cell.vi"("Active Sheet"=w2368, "Header Rows to remove"=3, "sub array start"=w2370, "error in (no error)"=w2377) -> ("row max value"=w2369:i32, 13:"start of last occupied row"=w2376:cluster{"row":i32, "column":i32}, 14:"start of last occupied row"=w2367:string, "error out"=w2366:errorcluster)  [unwired: 5 in, 3 out]
                    n954 = local write "row max value"(w2369) -> ()
                    n955 = local write "last occupied cell's name"(w2367) -> ()
                  }
                }
              }
            }
          }
          frame "Init" {
            n956 = flat-sequence {
              tunnel: w2401 -> [w2818]
              tunnel: [w2800] -> w2378
              tunnel: [w2804] -> w2391
              frame #0 {
                w2799 = T26."Enabled" ("Disabled")
                n957 = property on="Start KPRO" class="Bool"("DisabledEnum"=w2799) -> ()  [unwired: 2 in, 2 out]
                n958 = property on="stop" class="Bool (strict)"("DisabledEnum"=w2799) -> ()  [unwired: 2 in, 2 out]
                n959 = call "create DAQ strings.vi"("error in (no error)"=w2818, "MCC USB-DAQ Setup"="MCC USB-DAQ Setup") -> ("error IO"=w2811:errorcluster, "Descriptions"=w2809:string[], "delimited string"=w2812:string, "Array"=w2810:string[], "Voltage Range"=w2817:dbl[])  [unwired: 5 in]
                "delimited string" <- w2812
                "Active Channel Array" <- w2810
                "Voltage Range" <- w2817
                "Descriptions" <- w2809
                n960 = call "Physical Channels to Number of channels.vi"("error in (no error)"=w2811, "Physical Channel in"=w2812) -> ("error out"=w2813:errorcluster, "Number of Channels"=w2815:i32)  [unwired: 7 in, 1 out]
                "Number \nof Channels" <- w2815
                n961 = call "Calculate Rate from Num Channels and Max Rate.vi"("error in (no error)"=w2813, "Channel Data Rate S/s"="DAQ \nData Rate S/s", "Number of Channels"=w2815) -> ("error out"=w2808:errorcluster, "Rate"=→"Rate":dbl)  [unwired: 7 in]
                n962 = for {
                  tunnel: w2810 -> [w2831] mode=indexing
                  tunnel: w2817 -> [w2830] mode=indexing
                  tunnel: [w2827] -> w2807 mode=indexing
                  shift-right: [w2828] -> w2806
                  shift-left: w2808 -> [w2826]
                  n963 = Negate(x=w2830) -> (-x=w2829:dbl)
                  n964 = call-poly <vilib>:"ULx Create Virtual Channel.vi"("maximum value"=w2830, "minimum value"=w2829, "physical channels"=w2831, "error in"=w2826) -> ("task out"=w2827:refnum<k24>, "error out"=w2828:errorcluster)  [unwired: 10 in]
                }
                n965 = call "get 9V monitor voltage.vi"("error in (no error)"=w2806, "Descriptions"=w2809, "Array"=w2810, "Array 2"=w2807) -> ("error out"=w2805:errorcluster, "9V Voltage Monitor"=w2803:dbl)  [unwired: 6 in]
                "DAQ Error" <- w2805
                "9V Voltage Monitor" <- w2803
                n966 = Greater Or Equal?(x=w2803, y=8.75) -> (x >= y?=→"DAQ":bool)
                n967 = flat-sequence {
                  tunnel: [w2824] -> w2804
                  tunnel: w2807 -> [w2822]
                  tunnel: w2805 -> [w2821]
                  frame #0 {
                    n968 = local read "Descriptions"() -> (w2825:string[])
                    n969 = call "Measure DAQ Voltages.vi"("error in (no error)"=w2821, "Descriptions"=w2825, "Array in"=w2822) -> ("Raw Voltages"=w2823:dbl[], "Array out"=w2824:refnum<k24>[], "Sensor Cluster"=w2820:T11)  [unwired: 6 in]
                    n970 = local write "Sensor Voltage Cluster"(w2820) -> ()
                    n971 = local write "Raw Voltages"(w2823) -> ()
                  }
                }
                n972 = call <vilib>:"Clear Errors.vi"("error in (no error)"=w2805) -> ("error out"=w2800:errorcluster)  [unwired: 5 in, 1 out]
              }
            }
            n973 = local write "Initialization"(-1 ("Initialization")) -> ()
            n974 = flat-sequence {
              tunnel: [w2789] -> w2399
              tunnel: w2378 -> [w2789]
              frame #0 {
                w2793 = T26."Enabled" ("Disabled")
                n975 = invoke on="IK Reason array" class="Arr (strict)" method="Reinit To Default"() -> (error out=w2788:errorcluster)  [unwired: 3 in, 2 out]
                n976 = property on="Write Data to Spreadsheet" class="Bool"("DisabledEnum"=w2793) -> (error out=w2796:errorcluster)  [unwired: 2 in, 1 out]
                n977 = invoke on="Recording Reason Sonde array" class="Arr (strict)" method="Reinit To Default"(error in=w2788) -> ()  [unwired: 2 in, 3 out]
                n978 = property on="Record Continuous Samples" class="Bool"(error in=w2796, "DisabledEnum"=T26."Disabled and Grayed Out" ("Disabled")) -> (error out=w2795:errorcluster)  [unwired: 1 in, 1 out]
                n979 = local write "Sonde Data Array"(T29 [{"Head"=1.0, "Depth"=-5.5, "Time"="17:08:31", "Cumulative\nVolume"=100.0, "Sp. Conductance"={"Value"=2.0, "%"=0.0, "Tol."=TRUE}, "Dissolved Oxygen"={"Value"=3.0, "%"=0.0, "Tol."=TRUE}, "pH"={"Value"=4.0, "%"=0.0, "Tol."=TRUE}, "ORP"={"Value"=5.0, "%"=0.0, "Tol."=TRUE}, "Temperature"={"Value"=26.0, "%"=0.0, "Tol."=TRUE}, "Salinity"={"Value"=7.0, "%"=0.0, "Tol."=TRUE}, "Final Tol."=TRUE, "Final"=FALSE, "Time 2"=timestamp(3588613711.7180486 s since 1904-01-01), "Aux 1"=0.0, "Aux 2"=0.0, "Aux 3"=0.0}, {"Head"=1.0, "Depth"=-5.5, "Time"="17:08:34", "Cumulative\nVolume"=100.0, "Sp. Conductance"={"Value"=2.0, "%"=0.0, "Tol."=TRUE}, "Dissolved Oxygen"={"Value"=3.0, "%"=0.0, "Tol."=TRUE}, "pH"={"Value"=4.0, "%"=0.0, "Tol."=TRUE}, "ORP"={"Value"=5.0, "%"=0.0, "Tol."=TRUE}, "Temperature"={"Value"=26.0, "%"=0.0, "Tol."=TRUE}, "Salinity"={"Value"=7.0, "%"=0.0, "Tol."=TRUE}, "Final Tol."=TRUE, "Final"=FALSE, "Time 2"=timestamp(3588613714.1021852 s since 1904-01-01), "Aux 1"=0.0, "Aux 2"=0.0, "Aux 3"=0.0}, {"Head"=1.0, "Depth"=-5.5, "Time"="17:08:35", "Cumulative\nVolume"=100.0, "Sp. Conductance"={"Value"=2.0, "%"=0.0, "Tol."=TRUE}, "Dissolved Oxygen"={"Value"=3.0, "%"=0.0, "Tol."=TRUE}, "pH"={"Value"=4.0, "%"=0.0, "Tol."=TRUE}, "ORP"={"Value"=5.0, "%"=0.0, "Tol."=TRUE}, "Temperature"={"Value"=26.0, "%"=0.0, "Tol."=TRUE}, "Salinity"={"Value"=7.0, "%"=0.0, "Tol."=TRUE}, "Final Tol."=TRUE, "Final"=FALSE, "Time 2"=timestamp(3588613715.709277 s since 1904-01-01), "Aux 1"=0.0, "Aux 2"=0.0, "Aux 3"=0.0}, {"Head"=1.0, "Depth"=-5.5, "Time"="17:08:37", "Cumulative\nVolume"=100.0, "Sp. Conductance"={"Value"=2.0, "%"=0.0, "Tol."=TRUE}, "Dissolved Oxygen"={"Value"=3.0, "%"=0.0, "Tol."=TRUE}, "pH"={"Value"=4.0, "%"=0.0, "Tol."=TRUE}, "ORP"={"Value"=5.0, "%"=0.0, "Tol."=TRUE}, "Temperature"={"Value"=26.0, "%"=0.0, "Tol."=TRUE}, "Salinity"={"Value"=7.0, "%"=0.0, "Tol."=TRUE}, "Final Tol."=TRUE, "Final"=FALSE, "Time 2"=timestamp(3588613717.7793956 s since 1904-01-01), "Aux 1"=0.0, "Aux 2"=0.0, "Aux 3"=0.0}, {"Head"=1.0, "Depth"=-5.5, "Time"="17:08:39", "Cumulative\nVolume"=100.0, "Sp. Conductance"={"Value"=2.0, "%"=0.0, "Tol."=TRUE}, "Dissolved Oxygen"={"Value"=3.0, "%"=0.0, "Tol."=TRUE}, "pH"={"Value"=4.0, "%"=0.0, "Tol."=TRUE}, "ORP"={"Value"=5.0, "%"=0.0, "Tol."=TRUE}, "Temperature"={"Value"=26.0, "%"=0.0, "Tol."=TRUE}, "Salinity"={"Value"=7.0, "%"=0.0, "Tol."=TRUE}, "Final Tol."=TRUE, "Final"=FALSE, "Time 2"=timestamp(3588613719.696505 s since 1904-01-01), "Aux 1"=0.0, "Aux 2"=0.0, "Aux 3"=0.0}, {"Head"=1.0, "Depth"=-5.5, "Time"="17:09:28", "Cumulative\nVolume"=100.0, "Sp. Conductance"={"Value"=2.0, "%"=0.0, "Tol."=TRUE}, "Dissolved Oxygen"={"Value"=3.0, "%"=0.0, "Tol."=TRUE}, "pH"={"Value"=4.0, "%"=0.0, "Tol."=TRUE}, "ORP"={"Value"=5.0, "%"=0.0, "Tol."=TRUE}, "Temperature"={"Value"=26.0, "%"=0.0, "Tol."=TRUE}, "Salinity"={"Value"=7.0, "%"=0.0, "Tol."=TRUE}, "Final Tol."=TRUE, "Final"=FALSE, "Time 2"=timestamp(3588613768.340287 s since 1904-01-01), "Aux 1"=0.0, "Aux 2"=0.0, "Aux 3"=0.0}] ("Sonde Data Array")) -> ()
                n980 = property on="Record Single Sample" class="Bool"(error in=w2795, "DisabledEnum"=w2793) -> (error out=w2794:errorcluster)  [unwired: 1 in, 1 out]
                n981 = property on="Sonde Sample Not Collected" class="Bool"(error in=w2794, "DisabledEnum"=w2793) -> (error out=w2792:errorcluster)  [unwired: 1 in, 1 out]
                n982 = invoke on="Sonde Data Array" class="Arr (strict)" method="Reinit To Default"(error in=w2792) -> ()  [unwired: 2 in, 3 out]
                "Initialization Finished" <- TRUE
                "Zero Pressure\nIndicator" <- FALSE ("Zero Pressure\nIndicator")
              }
            }
            n983 = call <vilib>:"Clear Errors.vi"("error in (no error)"=w2378) -> ("error out"=w2379:errorcluster)  [unwired: 5 in, 1 out]
            n984 = local read "Descriptions"() -> (w2380:string[])
            n985 = stacked-sequence {
              seq-local: [w2408 _ _ _ _ _ _ _ _ _] -> [_ w2437 _ _ _ _ _ _ _ _]
              seq-local: [_ w2438 _ _ _ _ _ _ _ _] -> [_ _ w2459 _ _ _ _ _ _ _]
              seq-local: [_ _ w2458 _ _ _ _ _ _ _] -> [_ _ _ _ _ _ _ _ _ w2737]
              tunnel: [_ _ w2463 _ _ _ _ _ _ _] -> _
              tunnel: w2393 -> [_ _ _ _ _ _ _ _ _ w2740]
              tunnel: [_ _ _ _ _ _ _ _ _ w2739] -> w2392
              tunnel: w2379 -> [w2410 _ _ _ _ _ _ _ _ _]
              tunnel: w2391 -> [_ _ w2461 w2642 w2671 _ _ _ w2708 _]
              tunnel: w2380 -> [_ _ w2460 w2643 w2670 _ _ _ w2707 _]
              tunnel: [_ _ _ w2644 _ _ _ _ _ _] -> _
              tunnel: [_ _ _ _ _ _ _ _ _ w2737] -> w2394
              tunnel: w2383 -> [_ _ w2457 _ _ _ _ _ _ _]
              tunnel: [_ _ w2456 _ _ _ _ _ _ _] -> w2382
              frame #0 {
                n986 = flat-sequence {
                  tunnel: [w2415] -> w2408
                  tunnel: w2410 -> [w2416]
                  frame #0 {
                    n987 = local read "Groundwater Header"() -> (w2422:T12)
                    n988 = Unbundle By Name(w2422) -> ("Kpro box Serial"=w2412:string)
                    n989 = Scan From String(format string="%d", input string=w2412, error in=w2416, default 1=800.0 ("default value 1")) -> (error out=w2417:errorcluster, output 1=w2421:dbl)  [unwired: 1 in, 2 out]
                    n990 = Equal?(x=w2412, y="") -> (x = y?=w2413:bool)
                    n991 = case shown="True" w2413 {
                      tunnel: "KPRO Box Number\n\nEnter the number of the KPRO box you are using." ("prompt") -> [_ w2436]
                      tunnel: w2422 -> [w2426 w2435]
                      tunnel: w2421 -> [w2424 w2434]
                      tunnel: [w2424 w2433] -> w2420
                      tunnel: [w2426 w2431] -> w2418
                      tunnel: w2417 -> [w2425 w2429]
                      tunnel: [w2425 w2428] -> w2415
                      frame False {
                      }
                      frame True {
                        n992 = call "prompt_and_enter_value2.vi"("prompt_IN"=w2436, "Enter value"=w2434) -> ("Numeric"=w2433:dbl)  [unwired: 9 in]
                        n993 = call <vilib>:"Clear Errors.vi"("error in (no error)"=w2429) -> ("error out"=w2427:errorcluster)  [unwired: 5 in, 1 out]
                        n994 = Format Into String(format string="%d", error in=w2427, w2433) -> (resulting string=w2430:string, error out=w2428:errorcluster)  [unwired: 1 in]
                        n995 = Bundle By Name(cluster=w2435, "Kpro box Serial"=w2430) -> (w2431:T12)
                      }
                    }
                    n996 = global write "Kpro Globals.vi" "KPRO Box Number"(w2420) -> ()
                    n997 = local write "Groundwater Header"(w2418) -> ()
                  }
                }
                "Initialization" <- 0
              }
              frame #1 {
                n998 = local write "Initialization"(1 ("Initialization")) -> ()
                n999 = flat-sequence {
                  tunnel: w2437 -> [w2441]
                  tunnel: [w2440] -> w2438
                  frame #0 {
                    n1000 = local read "Groundwater Header"() -> (w2449:T12)
                    n1001 = local read "Temporary Data Files Directory"() -> (w2445:path)
                    n1002 = Unbundle By Name(w2449) -> ("Profile ID"=w2448:string)
                    n1003 = Equal?(x=w2448, y="") -> ()  [unwired: 1 out]
                    n1004 = case shown="True" TRUE {
                      tunnel: "Profile ID\n\nEnter the profile ID.  This will create a directoryto store csv files and the excel file" ("prompt") -> [_ w2455]
                      tunnel: [w2452 w2454] -> w2444
                      tunnel: w2448 -> [w2452 w2453]
                      frame False {
                      }
                      frame True {
                        n1005 = call "prompt_string.vi"("prompt_IN"=w2455, "Enter value"=w2453) -> ("String"=w2454:string)  [unwired: 9 in]
                        n1006 = global write "Kpro Globals.vi" "Profile ID"(w2454) -> ()
                      }
                    }
                    n1007 = Bundle By Name(cluster=w2449, "Profile ID"=w2444) -> (w2450:T12)
                    n1008 = call-poly <userlib>:"Build Path__ogtk.vi"("name or relative path"=w2444, "base path"=w2445) -> ("appended path"=w2443:path)
                    n1009 = local write "Groundwater Header"(w2450) -> ()
                    n1010 = call <userlib>:"Create Dir if Non-Existant__ogtk.vi"("error in (no error)"=w2441, "Directory Path"=w2443) -> ("error out"=w2440:errorcluster, "dup Directory Path"=w2442:path)  [unwired: 7 in, 1 out]
                    n1011 = local write "Output File Path"(w2442) -> ()
                  }
                }
              }
              frame #2 {
                n1012 = flat-sequence {
                  tunnel: [w2488] -> w2463
                  tunnel: w2459 -> [w2469]
                  tunnel: w2461 -> [w2490]
                  tunnel: w2460 -> [w2489]
                  tunnel: [w2475] -> w2458
                  tunnel: w2457 -> [w2485]
                  tunnel: [w2484] -> w2456
                  frame #0 {
                    n1013 = flat-sequence {
                      tunnel: [w2499] -> w2468
                      frame #0 {
                        w2499 = string[] ["Measurement Time", "Current Absolute Depth (Uncorrected)", "Corrected Depth", "Depth Rate", "Flow", "Feet of Stainless Steel Used", "In line Pressure Sensor", "IK", "Corrected Headloss", "Atmospheric Pressure (global)", "Depth to Water Table (global)", "Height of Box (global)", "Resevoir Pressure (global)", "Seconds since Jan 1 1904", "Marker", "Downhole Pressure Sensor (ft/H20)", "Downhole Pressure Sensor (V)", "DHT Depth to Water", "DHT IK"] ("Array")
                        n1014 = local write "KPRO Culmulative \ntest report header 2"(w2499) -> ()
                        n1015 = local write "KPRO session report header"(w2499) -> ()
                      }
                    }
                    n1016 = local read "Input Variables and Slopes"() -> (w2495:T2)
                    n1017 = call <vilib>:"Clear Errors.vi"("error in (no error)"=w2469) -> ("error out"=w2486:errorcluster)  [unwired: 5 in, 1 out]
                    n1018 = local read "Temporary Data Files Directory"() -> (w2491:path)
                    n1019 = Unbundle By Name(w2495) -> ("Up Hole Pressure Slope"=w2498:dbl, "String Pot Slope"=w2497:dbl, "Flow Slope"=w2496:dbl)
                    n1020 = call "FILE_DIALOG 2016.vi"("flow_slope_IN"=w2496, "pressure_slope_IN"=w2498, "string_pot_slope_IN"=w2497, "Descriptions"=w2489, "error in (no error)"=w2486, "start path"=w2491, "Array in"=w2490) -> ("Output path"=w2470:path, "exists"=w2466:bool, "flow_slope_OUT"=w2493:dbl, "pressure_slope_OUT"=w2492:dbl, "Record Output Slopes to  Record File"=w2482:path, "string_pot_slope_OUT"=w2494:dbl, "Record Output Slopes for slopes.csv File"=w2483:path, "error out"=w2474:errorcluster)  [unwired: 10 in, 3 out]
                    n1021 = stacked-sequence {
                      seq-local: [_ w2524 _ _ _ _ _ _ _ _ _] -> [_ _ w2538 _ _ _ _ _ _ _ _]
                      seq-local: [w2503 _ _ _ _ _ _ _ _ _ _] -> [_ w2526 w2539 w2547 _ w2561 w2570 w2582 w2590 w2595 _]
                      tunnel: [_ w2525 _ _ _ _ _ _ _ _ _] -> w2481
                      tunnel: [_ _ w2544 _ _ _ _ _ _ _ _] -> w2480
                      tunnel: [_ _ _ w2548 _ _ _ _ _ _ _] -> w2479
                      tunnel: [_ _ _ _ _ _ w2571 _ _ _ _] -> w2478
                      tunnel: [_ _ _ _ _ _ _ w2583 _ _ _] -> w2477
                      tunnel: [_ _ _ _ _ _ _ _ _ _ w2600] -> w2476
                      tunnel: [_ w2527 _ _ _ _ _ _ _ _ _] -> w2471
                      tunnel: w2470 -> [w2502 _ _ _ _ _ _ _ _ _ _]
                      tunnel: w2468 -> [_ w2524 _ _ _ _ _ _ _ _ _]
                      tunnel: w2466 -> [w2500 _ _ _ _ _ _ _ _ _ _]
                      frame #0 {
                        n1022 = case shown="True" w2500 {
                          tunnel: w2502 -> [w2510 w2512]
                          tunnel: [w2510 w2511] -> w2501
                          frame False {
                          }
                          frame True {
                            n1023 = call-poly <userlib>:"File Exists__ogtk.vi"("file path"=w2512) -> ("is directory"=w2513:bool)  [unwired: 6 in, 1 out]
                            n1024 = case shown="False" w2513 {
                              tunnel: w2512 -> [w2514 w2516]
                              tunnel: [w2515 w2517] -> w2511
                              frame False {
                                n1025 = call-poly <userlib>:"Strip Path__ogtk.vi"("path"=w2514) -> ("stripped path"=w2515:path)  [unwired: 1 out]
                                n1026 = local write "KPRO Cumulative Output File Path"(w2514) -> ()
                              }
                              frame True {
                                n1027 = local read "Temporary Data Files Directory"() -> (w2520:path)
                                n1028 = call-poly <userlib>:"Strip Path__ogtk.vi"("path"=w2516) -> ("stripped path"=w2518:path)  [unwired: 1 out]
                                n1029 = Not Equal?(x=w2518, y=w2520) -> (x != y?=w2519:bool)
                                n1030 = Select(t=w2518, s=w2519, f=w2516) -> (s? t:f=w2517:path)
                              }
                            }
                          }
                        }
                        n1031 = Path To String(path=w2501) -> (string=w2506:string)
                        n1032 = Concatenate Strings(w2506, "\\" ("string")) -> (w2508:string)
                        n1033 = String To Path(string=w2508) -> (path=w2507:path)
                        "Output File Path" <- w2507
                        n1034 = call-poly <userlib>:"Strip Path__ogtk.vi"("path"=w2507) -> ("name"=w2504:string)  [unwired: 1 out]
                        n1035 = Concatenate Strings(w2508, w2504) -> (w2505:string)
                        n1036 = String To Path(string=w2505) -> (path=w2503:path)
                        "appended path" <- w2503
                      }
                      frame #1 {
                        n1037 = Path To String(path=w2526) -> (string=w2528:string)
                        n1038 = Concatenate Strings(w2528, "_KPROcumulative.csv") -> (w2530:string)
                        n1039 = String To Path(string=w2530) -> (path=w2523:path)
                        "KPRO Cumulative Output File Path" <- w2523
                        n1040 = call <vilib>:"Check if File or Folder Exists.vi"("path"=w2523) -> ("file or folder exists?"=w2521:bool, "dup path"=w2522:path)  [unwired: 8 in, 1 out]
                        n1041 = case shown="False" w2521 {
                          tunnel: [w2534 _] -> w2525
                          tunnel: w2522 -> [w2533 w2537]
                          tunnel: [w2532 w2537] -> w2527
                          tunnel: w2524 -> [w2531 _]
                          frame False {
                            n1042 = call-poly <vilib>:"Write Delimited Spreadsheet.vi"("file path (dialog if empty)"=w2533, "1D data"=w2531, "append to file? (new file:F)"=FALSE, "delimiter (\\t)"="," ("delimiter (\\t)")) -> ("new file path (Not A Path if cancelled)"=w2532:path, "error out"=w2534:errorcluster)  [unwired: 10 in]
                          }
                          frame True {
                          }
                        }
                      }
                      frame #2 {
                        n1043 = Path To String(path=w2539) -> (string=w2542:string)
                        n1044 = Concatenate Strings(w2542, "_KPROsession.csv") -> (w2543:string)
                        n1045 = String To Path(string=w2543) -> (path=w2540:path)
                        "KPRO SessionOutput File Path" <- w2540
                        n1046 = call-poly <vilib>:"Write Delimited Spreadsheet.vi"("file path (dialog if empty)"=w2540, "1D data"=w2538, "append to file? (new file:F)"=FALSE, "delimiter (\\t)"="," ("delimiter (\\t)")) -> ("error out"=w2544:errorcluster)  [unwired: 10 in, 1 out]
                      }
                      frame #3 {
                        n1047 = Path To String(path=w2547) -> (string=w2553:string)
                        n1048 = Concatenate Strings(w2553, "_SondeData.csv" ("string")) -> (w2554:string)
                        n1049 = String To Path(string=w2554) -> (path=w2550:path)
                        "Sonde Output File Path" <- w2550
                        n1050 = local write "Sonde Output File Path"(w2550) -> ()
                        n1051 = call "convert sonde cluster to spreadsheet array.vi"() -> ("sonde labels"=w2552:string[])  [unwired: 8 in, 3 out]
                        n1052 = call-poly <vilib>:"Write Delimited Spreadsheet.vi"("file path (dialog if empty)"=w2550, "1D data"=w2552, "append to file? (new file:F)"=FALSE, "delimiter (\\t)"="," ("delimiter (\\t)")) -> ("error out"=w2548:errorcluster)  [unwired: 10 in, 1 out]
                      }
                      frame #4 {
                        n1053 = local read "Temporary Data Files Directory"() -> (w2556:path)
                        n1054 = Path To String(path=w2556) -> (string=w2558:string)
                        n1055 = Concatenate Strings(w2558, "Sonde_Calibration_History.csv" ("string")) -> (w2559:string)
                        n1056 = String To Path(string=w2559) -> (path=w2557:path)
                        n1057 = local write "Sonde Calibration History File"(w2557) -> ()
                      }
                      frame #5 {
                        n1058 = Path To String(path=w2561) -> (string=w2563:string)
                        n1059 = Concatenate Strings(w2563, "_Groundwater Profiling Log.xlsx" ("string")) -> (w2564:string)
                        n1060 = String To Path(string=w2564) -> (path=w2562:path)
                        n1061 = local write "Excel report file path"(w2562) -> ()
                      }
                      frame #6 {
                        w2567 = string[] ["Time", "Head Pressure", "Depth", "Select Entry Value", "Select Entry String"]
                        n1062 = local read "Recording Reason Sonde array"() -> (w2568:string[][])
                        n1063 = Path To String(path=w2570) -> (string=w2572:string)
                        n1064 = Concatenate Strings(w2572, "_Sample failure.csv" ("new ending (none)")) -> (w2575:string)
                        n1065 = String To Path(string=w2575) -> (path=w2573:path)
                        "Sonde Recording Failure Path" <- w2573
                        "Sonde Recording Error file" <- w2573
                        n1066 = Insert Into Array(array=w2568, index (row)=0, new element=w2567) -> (w2569:string[][])  [unwired: 1 in]
                        n1067 = local write "Recording Reason Sonde array"(w2569) -> ()
                        n1068 = call-poly <vilib>:"Write Delimited Spreadsheet.vi"("file path (dialog if empty)"=w2573, "1D data"=w2567, "append to file? (new file:F)"=FALSE, "delimiter (\\t)"="," ("delimiter (\\t)")) -> ("error out"=w2571:errorcluster)  [unwired: 10 in, 1 out]
                      }
                      frame #7 {
                        w2579 = string[] ["Time", "Head Pressure", "Depth", "Select Entry Value", "Select Entry String", "Flow", "Corrected Pressure ", "Feet of Stainless Steel Used", "Ik"]
                        n1069 = local read "IK Reason array"() -> (w2580:string[][])
                        n1070 = local write "appended path"(w2582) -> ()
                        n1071 = Path To String(path=w2582) -> (string=w2585:string)
                        n1072 = Concatenate Strings(w2585, "_IK failure.csv" ("new ending (none)")) -> (w2586:string)
                        n1073 = String To Path(string=w2586) -> (path=w2584:path)
                        "IK Recording Error file" <- w2584
                        n1074 = local write "Sonde IK Recording Failure Path"(w2584) -> ()
                        n1075 = Insert Into Array(array=w2580, index (row)=0, new element=w2579) -> (w2581:string[][])  [unwired: 1 in]
                        n1076 = local write "IK Reason array"(w2581) -> ()
                        n1077 = call-poly <vilib>:"Write Delimited Spreadsheet.vi"("file path (dialog if empty)"=w2584, "1D data"=w2579, "append to file? (new file:F)"=FALSE, "delimiter (\\t)"="," ("delimiter (\\t)")) -> ("error out"=w2583:errorcluster)  [unwired: 10 in, 1 out]
                      }
                      frame #8 {
                        n1078 = local write "appended path"(w2590) -> ()
                        n1079 = Path To String(path=w2590) -> (string=w2592:string)
                        n1080 = Concatenate Strings(w2592, "_DHT Data.csv" ("new ending (none)")) -> (w2593:string)
                        n1081 = String To Path(string=w2593) -> (path=→"Down hole Pressure Transducer CSV data  path":path)
                      }
                      frame #9 {
                        n1082 = Path To String(path=w2595) -> (string=w2596:string)
                        n1083 = Concatenate Strings(w2596, "_Static Ik.csv" ("string")) -> (w2598:string)
                        n1084 = String To Path(string=w2598) -> (path=w2597:path)
                        n1085 = local write "Static IK path"(w2597) -> ()
                      }
                      frame #10 {
                        n1086 = Build Array("Profile ID   " ("string"), "Depth    " ("string"), "Flow " ("string"), "Ik    " ("string")) -> (w2602:string[])
                        n1087 = call-poly <vilib>:"Write Delimited Spreadsheet.vi"("file path (dialog if empty)"="Static IK path", "1D data"=w2602, "append to file? (new file:F)"=FALSE, "delimiter (\\t)"="," ("delimiter (\\t)")) -> ("error out"=w2600:errorcluster)  [unwired: 10 in, 1 out]
                      }
                    }
                    n1088 = global write "Kpro Globals.vi" "Pressure \nSlope"(w2492) -> ()
                    n1089 = global write "Kpro Globals.vi" "Flow Slope"(w2493) -> ()
                    n1090 = global write "Kpro Globals.vi" "String Pot \nSlope"(w2494) -> ()
                    n1091 = Bundle By Name(cluster=w2495, "String Pot Slope"=w2494, "Flow Slope"=w2493, "Up Hole Pressure Slope"=w2492) -> (w2465:T2)
                    n1092 = local write "Slopes History File Path"(w2482) -> ()
                    n1093 = local write "Slopes File Path"(w2483) -> ()
                    n1094 = Unbundle By Name(w2465) -> ("Depth to Water Table"=w2464:dbl)
                    n1095 = local write "Depth to Water"(w2464) -> ()
                    n1096 = local write "Input Variables and Slopes"(w2465) -> ()
                    n1097 = Merge Errors(w2474, w2481, w2480, w2479, w2478, w2477, w2476) -> (w2473:errorcluster)
                    n1098 = call <vilib>:"Check if File or Folder Exists.vi"("error in (no error)"=w2473, "path"=w2471) -> ("error out"=w2472:errorcluster, "file or folder exists?"=w2467:bool, "dup path"=w2487:path)  [unwired: 7 in]
                    n1099 = case shown="True" w2467 {
                      selector: w2467 -> [_ w2616]
                      tunnel: w2487 -> [_ w2626]
                      tunnel: w2465 -> [w2611 w2621]
                      tunnel: [w2611 w2620] -> w2488
                      tunnel: w2472 -> [w2610 w2617]
                      tunnel: [w2610 w2617] -> w2475
                      tunnel: w2485 -> [w2609 w2615]
                      tunnel: [w2609 w2614] -> w2484
                      frame False {
                      }
                      frame True {
                        n1100 = call "Get_KPRO_data_from_file 2016.vi"("Output File KPRO Test"=w2626) -> ("Last_height_of_box"=w2619:dbl, "Last_depth_to_water"=w2612:dbl, "Last_depth"=w2618:dbl, "Output_array"=w2613:sgl[][])  [unwired: 7 in]
                        "Cumulative_data_from_file" <- w2613
                        "Depth to Water" <- w2612
                        n1101 = Bundle By Name(cluster=w2621, "Depth to Water Table"=w2612, "Height of Sample Box"=w2619) -> (w2620:T2)
                        n1102 = Bundle By Name(cluster=w2615, "Absolute Depth In"=w2618, "Current Absolute Depth"=w2618) -> (w2614:T21)
                        n1103 = call "Array to Plot 2016.vi"("Input Cumulative Array"=w2613) -> ("Cumulative - Depth vs.Drive Rate"=w2622:cluster{dbl[], dbl[]}, "Cumulative - Depth vs. Ik"=w2623:cluster{dbl[], dbl[]})  [unwired: 3 in, 4 out]
                        n1104 = local read "Culmulative Graph Cluster"() -> (w2625:T24)
                        n1105 = Bundle By Name(cluster=w2625, "Cumulative - Depth vs. Ik"=w2623, "Cumulative - Depth vs. Drive Rate"=w2622) -> (w2624:T24)
                        n1106 = local write "Input Variables and Slopes"(w2620) -> ()
                        n1107 = local write "Culmulative Graph Cluster"(w2624) -> ()
                        "Cumulative_data_ready" <- w2616
                      }
                    }
                  }
                }
                n1108 = local write "Initialization"(2 ("Initialization")) -> ()
              }
              frame #3 {
                # "Take offset and put\n into Pressure VI."
                n1109 = local write "Initialization"(3 ("Initialization")) -> ()
                n1110 = local read "Groundwater Header"() -> (w2634:T12)
                n1111 = global read "Kpro Globals.vi" "Pressure Offset"() -> (w2627:dbl)
                n1112 = local read "Input Variables and Slopes"() -> (w2632:T2)
                n1113 = Unbundle By Name(w2634) -> ("Atmospheric Pressure"=w2631:string)
                n1114 = case shown="True" TRUE {
                  tunnel: "ATMOSPHERIC PRESSURE READING\n\nHold Kpro effluent facing up and level with the pressure transducer.\nTurn on Kpro water, turn off when water flows with no air bubbles.\n\nPress OK when the reading equilibrates." ("message") -> [_ w2668]
                  tunnel: [w2659 w2667] -> w2649
                  tunnel: [w2658 w2661] -> w2646
                  tunnel: w2643 -> [_ w2666]
                  tunnel: w2642 -> [w2656 w2665]
                  tunnel: [w2657 w2664] -> w2641
                  tunnel: [w2653 w2663] -> w2636
                  tunnel: [w2656 w2662] -> w2635
                  tunnel: w2632 -> [w2658 w2661]
                  tunnel: w2631 -> [w2654 _]
                  tunnel: [w2652 w2660] -> w2628
                  tunnel: w2627 -> [w2652 w2660]
                  frame False {
                    n1115 = local read "Sensor Voltage Cluster"() -> (w2659:T11)
                    n1116 = Unbundle By Name(w2658) -> ("Up Hole Pressure Slope"=w2657:dbl)
                    n1117 = Scan From String(input string=w2654, default 1=35.0 ("default value 1")) -> (output 1=w2653:dbl)  [unwired: 3 in, 3 out]
                  }
                  frame True {
                    n1118 = local read "Sensor Voltage Cluster"() -> (w2667:T11)
                    n1119 = Unbundle By Name(w2661) -> ("Up Hole Pressure Slope"=w2664:dbl)
                    n1120 = call "Up Hole PRESSURE_CAL 2016.vi"("Pressure \nOffset"=w2660, "Descriptions"=w2666, "Array in"=w2665, "Pressure \nSlope"=w2664, "Sensor Cluster"=w2667, "Prompt_IN"=w2668) -> ("PRESSURE\nFt of water"=w2663:dbl, "Array out"=w2662:refnum<k24>[])  [unwired: 4 in]
                  }
                }
                n1121 = Equal?(x=w2631, y="") -> ()  [unwired: 1 out]
                n1122 = local read "Corrected Pressure Cluster"() -> (w2648:T1)
                n1123 = Bundle By Name(cluster=w2646, "Atmospheric Pressure"=w2636, "Up Hole  Pressure Offset"=w2628) -> (w2645:T2)
                n1124 = global write "Kpro Globals.vi" "Atmospheric Pressure"(w2636) -> ()
                n1125 = Format Into String(w2636) -> (resulting string=w2637:string)  [unwired: 3 in, 1 out]
                n1126 = call "up hole Pressure 2016.vi"("Sensor Cluster"=w2649, "Pressure Offset"=w2636, "Array in"=w2635, "Pressure \nSlope"=w2641, "Descriptions"=w2643, "Zero Pressure\n(F = leave as is)"=TRUE) -> ("Array out"=w2644:refnum<k24>[], "Uphole Pressure"=w2629:dbl, "Sensor Cluster 2"=w2639:T11)  [unwired: 6 in, 1 out]
                n1127 = Bundle By Name(cluster=w2634, "Atmospheric Pressure"=w2637) -> (w2638:T12)
                n1128 = Bundle By Name(cluster=w2648, "Up hole Corrected Pressure"=w2629) -> (w2647:T1)
                n1129 = local write "Sensor Voltage Cluster"(w2639) -> ()
                n1130 = local write "Input Variables and Slopes"(w2645) -> ()
                n1131 = local write "Groundwater Header"(w2638) -> ()
                n1132 = local write "Corrected\n Pressure (ft)"(w2629) -> ()
                n1133 = local write "Corrected Pressure Cluster"(w2647) -> ()
              }
              frame #4 {
                n1134 = local write "Initialization"(5 ("Initialization")) -> ()
                n1135 = flat-sequence {
                  tunnel: w2671 -> [w2680]
                  tunnel: w2670 -> [w2679]
                  frame #0 {
                    n1136 = local read "Input Variables and Slopes"() -> (w2678:T2)
                    n1137 = Unbundle By Name(w2678) -> ("Up Hole Pressure Slope"=w2677:dbl)
                    n1138 = local read "Sensor Voltage Cluster"() -> (w2683:T11)
                    n1139 = global read "Kpro Globals.vi" "Pressure Offset"() -> (w2676:dbl)
                    n1140 = call "Up Hole PRESSURE_CAL 2016.vi"("Pressure \nOffset"=w2676, "Descriptions"=w2679, "Array in"=w2680, "Pressure \nSlope"=w2677, "Sensor Cluster"=w2683, "Prompt_IN"="CHECK RESERVOIR PRESSURE\n\nTurn on Kpro. Unplug Kpro Out quick connect from sample box.\nReservoir pressure should be 69.2 +/- 5%(65.7 - 72.7).\n\nPress OK when the reading equilibrates within range." ("message")) -> ("PRESSURE\nFt of water"=w2673:dbl)  [unwired: 4 in, 1 out]
                    n1141 = local read "Groundwater Header"() -> (w2675:T12)
                    n1142 = Format Into String(w2673) -> (resulting string=w2672:string)  [unwired: 3 in, 1 out]
                    n1143 = global write "Kpro Globals.vi" "Reservoir Pressure"(w2673) -> ()
                    n1144 = Bundle By Name(cluster=w2678, "Reservoir Pressure"=w2673) -> (w2681:T2)
                    n1145 = Bundle By Name(cluster=w2675, "KPRO N2 Pressure"=w2672) -> (w2674:T12)
                    n1146 = local write "Input Variables and Slopes"(w2681) -> ()
                    n1147 = local write "Groundwater Header"(w2674) -> ()
                  }
                }
              }
              frame #5 {
                n1148 = flat-sequence {
                  frame #0 {
                    n1149 = local read "Input Depths \nand Parameters Cluster"() -> (w2688:T19)
                    n1150 = Unbundle By Name(w2688) -> ("Start Depth"=w2685:sgl)
                    n1151 = call "prompt_and_enter_value 2016.vi"("prompt_IN"="ENTER START DEPTH", "Enter value"=w2685) -> ("Numeric"=w2690:dbl)  [unwired: 9 in]
                    n1152 = Absolute Value(x=w2690) -> (abs(x)=w2689:dbl)
                    n1153 = Negate(x=w2689) -> (-x=w2686:dbl)
                    n1154 = Bundle By Name(cluster=w2688, "Start Depth"=w2686) -> (w2687:T19)
                    n1155 = local write "Input Depths \nand Parameters Cluster"(w2687) -> ()
                  }
                }
                n1156 = local write "Initialization"(6 ("Initialization")) -> ()
              }
              frame #6 {
                n1157 = local write "Initialization"(7 ("Initialization")) -> ()
                n1158 = local read "Input Variables and Slopes"() -> (w2696:T2)
                n1159 = Unbundle By Name(w2696) -> ("Height of Sample Box"=w2694:dbl)
                n1160 = call "prompt_and_enter_value 2016.vi"("prompt_IN"="HEIGHT FROM GROUND SURFACE TO SAMPLE BOX\n\nMeasure the vertical distance between the ground surface and the pressure transducer." ("prompt"), "Enter value"=w2694) -> ("Numeric"=w2693:dbl)  [unwired: 9 in]
                n1161 = Bundle By Name(cluster=w2696, "Height of Sample Box"=w2693) -> (w2695:T2)
                n1162 = global write "Kpro Globals.vi" "height_of_box"(w2693) -> ()
                n1163 = local write "Input Variables and Slopes"(w2695) -> ()
              }
              frame #7 {
                n1164 = local write "Initialization"(8 ("Initialization")) -> ()
                n1165 = flat-sequence {
                  frame #0 {
                    n1166 = local read "Input Variables and Slopes"() -> (w2701:T2)
                    n1167 = Unbundle By Name(w2701) -> ("Depth to Water Table"=w2702:dbl)
                    n1168 = call "prompt_and_enter_value 2016.vi"("prompt_IN"="DEPTH TO WATER TABLE\n\nEnter the depth to the water table." ("prompt"), "Enter value"=w2702) -> ("Numeric"=w2704:dbl)  [unwired: 9 in]
                    n1169 = Absolute Value(x=w2704) -> (abs(x)=w2703:dbl)
                    n1170 = Negate(x=w2703) -> (-x=w2700:dbl)
                    n1171 = global write "Kpro Globals.vi" "Depth to Water Table"(w2700) -> ()
                    n1172 = Bundle By Name(cluster=w2701, "Depth to Water Table"=w2700) -> (w2699:T2)
                    n1173 = local write "Input Variables and Slopes"(w2699) -> ()
                  }
                }
              }
              frame #8 {
                n1174 = local write "Initialization"(9 ("Initialization")) -> ()
                n1175 = stacked-sequence {
                  tunnel: [w2709 _] -> _
                  tunnel: w2707 -> [w2713 w2732]
                  tunnel: w2708 -> [w2712 w2729]
                  tunnel: w2707 -> [_ w2730]
                  frame #0 {
                    # "Set to raw pressure mode"
                    n1176 = local read "Input Variables and Slopes"() -> (w2710:T2)
                    n1177 = local read "Sensor Voltage Cluster"() -> (w2717:T11)
                    n1178 = Unbundle By Name(w2710) -> ("Up Hole Pressure Slope"=w2709:dbl)
                    n1179 = local read "Corrected Pressure Cluster"() -> (w2715:T1)
                    n1180 = call "up hole Pressure 2016.vi"("Sensor Cluster"=w2717, "Pressure Offset"=0.0, "Array in"=w2712, "Pressure \nSlope"=w2709, "Descriptions"=w2713, "Zero Pressure\n(F = leave as is)"=TRUE) -> ("Uphole Pressure"=w2716:dbl)  [unwired: 6 in, 3 out]
                    n1181 = Bundle By Name(cluster=w2715, "Up hole Corrected Pressure"=w2716) -> (w2714:T1)
                    n1182 = local write "Corrected Pressure Cluster"(w2714) -> ()
                    n1183 = local read "Input Variables and Slopes 2"() -> (w2711:T2)
                    n1184 = Unbundle By Name(w2711) -> ()  [unwired: 1 out]
                  }
                  frame #1 {
                    # "adjust for 1 foot head"
                    # "Take offset and put\n into Pressure VI."
                    n1185 = local read "Input Variables and Slopes"() -> (w2724:T2)
                    n1186 = Unbundle By Name(w2724) -> ("Up Hole Pressure Slope"=w2723:dbl)
                    n1187 = local read "Sensor Voltage Cluster"() -> (w2733:T11)
                    n1188 = global read "Kpro Globals.vi" "Pressure Offset"() -> (w2731:dbl)
                    n1189 = local read "Corrected Pressure Cluster"() -> (w2721:T1)
                    n1190 = call "Up Hole PRESSURE_CAL 2016.vi"("Pressure \nOffset"=w2731, "Descriptions"=w2730, "Array in"=w2729, "Pressure \nSlope"=w2723, "Sensor Cluster"=w2733, "Prompt_IN"="ZERO TO GROUND SURFACE\n\nFill a grad cylinder to 750mL.\nPlace it on the ground at the profile location.\nImmerse the Kpro effluent and turn on Kpro flow.\nTurn off after water is flowing with no bubbles\nand the water has reached 800mL (1 foot).\n\nPress OK when the reading equilibrates." ("message")) -> ("PRESSURE\nFt of water"=w2734:dbl)  [unwired: 4 in, 1 out]
                    n1191 = Decrement(x=w2734) -> (x-1=w2728:dbl)
                    n1192 = call "up hole Pressure 2016.vi"("Sensor Cluster"=w2733, "Pressure Offset"=w2728, "Array in"=w2729, "Pressure \nSlope"=w2723, "Descriptions"=w2732, "Zero Pressure\n(F = leave as is)"=TRUE) -> ("Uphole Pressure"=w2720:dbl, "Pressure Offset 2"=w2725:dbl)  [unwired: 6 in, 2 out]
                    n1193 = Bundle By Name(cluster=w2721, "Up hole Corrected Pressure"=w2720) -> (w2722:T1)
                    n1194 = local read "Input Variables and Slopes"() -> (w2727:T2)
                    n1195 = Bundle By Name(cluster=w2727, "Up Hole  Pressure Offset"=w2725) -> (w2726:T2)
                    n1196 = local write "Input Variables and Slopes"(w2726) -> ()
                    n1197 = local write "Corrected Pressure Cluster"(w2722) -> ()
                  }
                }
              }
              frame #9 {
                n1198 = local write "Initialization"(10 ("Initialization")) -> ()
                n1199 = local read "Cumulative_data_ready"() -> (w2741:bool)
                n1200 = case shown="True" w2741 {
                  tunnel: w2740 -> [w2742 _]
                  tunnel: [w2742 w2743] -> w2739
                  frame False {
                  }
                  frame True {
                    n1201 = local write "Cumulative_data_ready"(TRUE ("Get_KPRO_data")) -> ()
                    n1202 = local read "Cumulative_data_from_file"() -> (w2743:sgl[][])
                  }
                }
              }
            }
            n1203 = flat-sequence {
              tunnel: "Read String Pot" -> [_]
              tunnel: [w2782] -> w2388
              tunnel: w2394 -> [w2766]
              tunnel: w2391 -> [w2767]
              frame #0 {
                w2772 = 0.0
                w2773 = TRUE
                # "Initialize Incrementer if using hand incrementer,\nDon't use Debug,\nPut use string pot into shift register first pass to avoid allowing\na change in which method is the source of the depth reading."
                n1204 = global write "Global_SIM_switch.vi" "enable_kpro_file"("enable_kpro_file") -> ()
                n1205 = global write "Global_SIM_switch.vi" "Simulate AD6B"("Simulate AD6B") -> ()
                n1206 = global write "Global_SIM_switch.vi" "enable_slug_file"("enable_slug_file") -> ()
                n1207 = local read "Input Variables and Slopes"() -> (w2780:T2)
                n1208 = global write "Global_SIM_switch.vi" "enable_IKMGS_file"("enable_IKMGS_file") -> ()
                n1209 = Unbundle By Name(w2780) -> ("String Pot Slope"=w2779:dbl, "Up Hole Pressure Slope"=w2775:dbl)  [unwired: 1 out]
                n1210 = local read "Sensor Voltage Cluster"() -> (w2774:T11)
                n1211 = local read "Descriptions"() -> (w2765:string[])
                n1212 = local read "Sensor Voltage Cluster"() -> (w2781:T11)
                n1213 = call "In-Line-Pressure 2016.vi"("Zero Pressure\n(F = leave as is)"=w2773, "In-Line Pressure Slope"=w2775, "Sensor Voltages Cluster"=w2774, "In-Line Pressure Offset"=w2772) -> ("Pressure"=w2776:dbl)  [unwired: 7 in]
                n1214 = call "up hole Pressure 2016.vi"("Sensor Cluster"=w2774, "Pressure Offset"=w2772, "Array in"=w2767, "Pressure \nSlope"=w2775, "Descriptions"=w2765, "Zero Pressure\n(F = leave as is)"=w2773) -> ("Array out"=w2764:refnum<k24>[], "Uphole Pressure"=w2761:dbl)  [unwired: 6 in, 2 out]
                n1215 = Bundle By Name(cluster="Corrected Pressure Cluster", "Up hole Corrected Pressure"=w2761, "Down hole Corrected Pressure"=w2776) -> (w2777:T1)
                n1216 = call "depth read from string pot 2016.vi"("Descriptions"=w2765, "error in (no error)"=w2766, "String Pot \nSlope"=w2779, "Array in"=w2764, "Sensor Cluster In"=w2781) -> ("Depth"=w2783:dbl)  [unwired: 11 in, 3 out]
                n1217 = local read "Sample Sheet Data Row Cluster 2"() -> (w2763:T3)
                n1218 = local write "Corrected Pressure Cluster"(w2777) -> ()
                n1219 = flat-sequence {
                  tunnel: w2783 -> [w2785]
                  tunnel: [w2784] -> w2782
                  frame #0 {
                    w2786 = 15  # Filter Size
                    # "Functional Global in \nBoxcar Integrator\nInitialize filter array to \ncurrent string pot value"
                    n1220 = call "Boxcar filter2016.vi"("Initialize"=TRUE, "Filter Size"=w2786, "Filter Input"=w2785) -> ("Filter Output"=w2784:dbl)
                  }
                }
                n1221 = Bundle By Name(cluster=w2763, "Head\nPressure"=w2761) -> (w2762:T3)
                n1222 = local write "Sample Sheet Data Row Cluster 2"(w2762) -> ()
              }
            }
            n1223 = flat-sequence {
              tunnel: [w2748] -> w2395
              tunnel: [w2747] -> w2389
              tunnel: w2388 -> [w2745]
              tunnel: [w2745] -> w2385
              frame #0 {
                n1224 = local read "Input Depths \nand Parameters Cluster"() -> (w2746:T19)
                n1225 = Unbundle By Name(w2746) -> ("Start Depth"=w2749:sgl)
                n1226 = Less Or Equal To 0?(x=w2749) -> (x <= 0?=w2751:bool)
                n1227 = Negate(x=w2749) -> (-x=w2750:sgl)
                n1228 = Select(t=w2749, s=w2751, f=w2750) -> (s? t:f=w2747:sgl)
                n1229 = Bundle By Name(cluster=w2746, "Abs Start Depth"=w2747, "Current Depth"=w2745) -> (w2748:T19)
                n1230 = local write "Input Depths \nand Parameters Cluster"(w2748) -> ()
              }
            }
            n1231 = flat-sequence {
              tunnel: [w2758] -> w2397
              frame #0 {
                n1232 = Tick Count (ms)() -> (millisecond timer value=w2760:u32)
                n1233 = Divide(x=w2760, y=u32 1000) -> (x/y=w2758:dbl)
              }
            }
            n1234 = flat-sequence {
              tunnel: [w2753] -> w2396
              tunnel: w2397 -> [w2756]
              tunnel: [w2755] -> _
              tunnel: w2389 -> [w2755]
              tunnel: w2385 -> [w2754]
              tunnel: w2382 -> [w2752]
              frame #0 {
                n1235 = Bundle By Name(cluster=w2752, "Absolute Depth In"=w2755, "Previous Relative Depth"=w2754, "Current Relative Depth"=w2754, "First Relative Depth"=w2754, "Current Absolute Depth"=w2755, "Last Filed Depth"=0.0, "Current Measurement Time"=w2756, "Previous Measurement Time"=w2756, "First Absolute Depth"=w2755) -> (w2753:T21)
              }
            }
          }
          frame "Acq. DAQ data" {
            n1236 = flat-sequence {
              tunnel: w2841 -> [w2858]
              tunnel: w2840 -> [w2857]
              tunnel: [w2854] -> w2839
              frame #0 {
                n1237 = local read "Descriptions"() -> (w2855:string[])
                n1238 = local read "Sensor  Real \nMeasurements"() -> (w2853:T8)
                n1239 = local read "Input Variables and Slopes"() -> (w2851:T2)
                n1240 = call "Measure DAQ Voltages.vi"("error in (no error)"=w2857, "Descriptions"=w2855, "Array in"=w2858) -> ("Raw Voltages"=→"Raw Voltages":dbl[], "Array out"=w2854:refnum<k24>[], "Sensor Cluster"=w2850:T11)  [unwired: 6 in]
                "Sensor Voltage Cluster" <- w2850
                n1241 = call "convert sensor voltage to real measurements.vi"("Input Variables and Slopes"=w2851, "Sensor  Real Measurements in"=w2853, "Sensor Cluster"=w2850) -> ("Sensor  Real Measurements out"=w2852:T11)  [unwired: 8 in]
                n1242 = local write "Sensor  Real \nMeasurements"(w2852) -> ()
              }
            }
          }
          frame "Exit" {
            n1243 = case shown="No Error" w2872 {
              tunnel: w2868 -> [w2905 _]
              tunnel: w2872 -> [w2904 w2916]
              tunnel: [w2903 w2916] -> w2870
              frame No Error {
                n1244 = for {
                  shift-right: [w2907] -> w2903
                  shift-left: w2904 -> [w2908]
                  tunnel: w2905 -> [w2906] mode=indexing
                  n1245 = while {
                    shift-right: [w2915] -> w2910
                    shift-left: w2908 -> [w2913]
                    shift-right: [w2914] -> w2909
                    shift-left: w2906 -> [w2912]
                    stop <- w2911 stop-if-true
                    n1246 = call <vilib>:"ULx Is Task Done.vi"("task in"=w2912, "error in"=w2913) -> ("task out"=w2914:refnum<k24>, "task done?"=w2911:bool, "error out"=w2915:errorcluster)  [unwired: 11 in]
                  }
                  n1247 = call <vilib>:"ULx Clear Task.vi"("task in"=w2909, "error in"=w2910) -> ("error out"=w2907:errorcluster)  [unwired: 13 in]
                }
              }
              frame Error {
              }
            }
            n1248 = flat-sequence {
              tunnel: [w2922] -> w2879
              tunnel: [w2921] -> w2880
              tunnel: w2860 -> [w2919]
              tunnel: w2859 -> [w2918]
              frame #0 {
                n1249 = local read "Excel report file path"() -> (w2917:path)
                n1250 = call-dynamic "Save Report to File.vi"("report in"=w2918, "report file path"=w2917, "prompt to replace? (F)"=FALSE, "error in (no error)"=w2919) -> ("report out"=w2922:refnum<class "NI_report.lvclass">, "error out"=w2921:errorcluster)  [unwired: 10 in]
              }
            }
            n1251 = call <userlib>:"Wait (ms)__ogtk.vi"("error in (no error)"=w2880, "milliseconds to wait"=u32 5) -> ("error out"=w2881:errorcluster)  [unwired: 8 in, 1 out]
            n1252 = flat-sequence {
              tunnel: w2881 -> [w2891]
              tunnel: w2879 -> [w2889]
              tunnel: [w2887] -> w2873
              frame #0 {
                (unwired) FALSE ("Write Ini")
                n1253 = call-dynamic "Dispose Report.vi"("report in"=w2889, "save changes? (F)"=FALSE, "error in (no error)"=w2891) -> ("error out"=w2886:errorcluster)  [unwired: 12 in]
                n1254 = case shown="False" "Save Configuration File?" {
                  tunnel: [errorcluster {"status"=FALSE, "code"=0, "source"=""} ("error IO") w2900] -> w2888
                  frame False {
                  }
                  frame True {
                    n1255 = local read "Config File Path"() -> (w2899:path)
                    n1256 = call <vilib>:"Open Config Data.vi"("create file if necessary (T)"=TRUE ("Read Ini"), "configuration file path"=w2899) -> ("error out"=w2897:errorcluster, "refnum"=w2894:T25)  [unwired: 7 in, 1 out]
                    n1257 = control-ref of="This VI"() -> (w2893:refnum<vi>)
                    n1258 = call <userlib>:"Write Panel to INI__ogtk.vi"("error in (no error)"=w2897, "VI ref"=w2893, "refnum"=w2894) -> ("error out"=w2896:errorcluster, "refnum out"=w2895:T25)  [unwired: 7 in]
                    n1259 = call <vilib>:"Clear Errors.vi"("error in (no error)"=w2896) -> ("error out"=w2902:errorcluster)  [unwired: 5 in, 1 out]
                    n1260 = call <vilib>:"Close Config Data.vi"("error in (no error)"=w2902, "refnum"=w2895) -> ("error out"=w2901:errorcluster)  [unwired: 8 in, 1 out]
                    n1261 = Merge Errors(w2901, w2896) -> (w2900:errorcluster)
                  }
                }
                n1262 = Merge Errors(w2888, w2886) -> (w2887:errorcluster)
              }
            }
            n1263 = flat-sequence {
              tunnel: [w2883] -> w2871
              tunnel: [w2884] -> w2869
              tunnel: w2870 -> [w2884]
              frame #0 {
                w2883 = TRUE ("aborted?")
                "Stop 2" <- w2883
              }
            }
          }
          frame "Create Excel Files" {
            n1264 = flat-sequence {
              tunnel: [w2956] -> w2925
              tunnel: w2924 -> [w2952]
              tunnel: [w2951] -> w2923
              frame #0 {
                n1265 = Get Date/Time In Seconds() -> (seconds since 1Jan1904=w2945:timestamp)
                n1266 = Get Date/Time String(seconds (now)=w2945) -> (date string=w2946:string, time string=w2943:string)  [unwired: 2 in]
                n1267 = local read "Output File Path"() -> (w2949:path)
                n1268 = Concatenate Strings(w2946, " " ("string"), w2943) -> (w2944:string)
                n1269 = Bundle By Name(cluster="Groundwater Header", "Date Finished"=w2944) -> (w2947:T12)
                n1270 = call "Write Excel Files.vi"("template file path"="template file path", "Header path"="Header path", "error IO"=w2952, "Run  Loop"=FALSE, "Output path to Directory"=w2949, "Groundwater Header"=w2947) -> ("error out"=w2956:errorcluster, "Excel report file path"=w2950:path, "NI_report out 2"=w2951:refnum<class "NI_report.lvclass">)  [unwired: 3 in]
                "NI_report out" <- w2951
                n1271 = local write "Excel report file path"(w2950) -> ()
              }
            }
            n1272 = flat-sequence {
              tunnel: [FALSE ("aborted?")] -> w2936
              tunnel: [w2958] -> w2935
              tunnel: w2926 -> [w2958]
              frame #0 {
              }
            }
          }
        }
        n1273 = local write "Depth Cluster"(w451) -> ()
        "Tab Page" <- "Tab Control"
      }
    }
  }
  n1274 = Merge Errors(w17, w16) -> (→"error out":errorcluster)
